vi "EC_Applied_XYZ_MM_BR_RES_2_NC_GR_pxi_Acc3_preset_LIM4.vi"() -> ()   [LabVIEW 2009]
uses:
  <vilib>/Utility/file.llb/Read From Spreadsheet File (I64).vi
  <vilib>/Utility/file.llb/Read From Spreadsheet File (string).vi
  <vilib>/Instr/_visa.llb/VISA Configure Serial Port (Instr).vi
  <vilib>/Utility/file.llb/Write To Spreadsheet File (I64).vi
  <vilib>/Utility/file.llb/Write To Spreadsheet File (string).vi
panel:
  out "R Velocity MVdeg/sec":dbl format="%.3f"
  out "R Position MV deg":dbl
  out "Z Velocity MV mm/sec":dbl format="%.3f"
  out "Z Position MV mm":dbl
  out "Y Velocity MV mm/sec":dbl format="%.3f"
  out "Y Position MV mm":dbl
  out "X Velocity MV mm/sec":dbl format="%.3f"
  out "X Position MV mm":dbl
  out "Presets":i32[][](array[numeric])
  in  "stop":bool
  in  "Tab Control 3":enum32{"Status", "Reset"}(tab)
  out "Y in Range":bool
  out "Y Scan":bool
  out "Y in Motion":bool
  out "Y Backlash corr":bool
  out "X  in Range":bool
  out "X Scan":bool
  out "X  in Motion":bool
  out "X Backlash corr":bool
  out "Z in Range":bool
  out "Z Scan":bool
  out "Z in Motion":bool
  out "Z Backlash corr":bool
  out "R in Range":bool
  out "R Scan":bool
  out "R in Motion":bool
  out "R Backlash corr":bool
  out "X Ready":bool
  out "Y Ready":bool
  out "Z Ready":bool
  out "R Ready":bool
  in  "Reset Y Position mm":dbl
  out "Reset Y Motor Steps":i32
  in  "Reset X Position mm":dbl
  out "Reset X Motor Steps":i32
  in  "Reset Z Position mm":dbl
  out "Reset Z Motor Steps":i32
  in  "Reset R Position deg":dbl
  out "Reset R Motor Steps":i32
  in  "Reset":bool
  in  "Tab Control 2":enum32{"mm", "step"}(tab)
  in  "X Scan Length SP mm":dbl
  in  "X Scan Velocity SP mm/sec":dbl
  in  "X Scan set":bool
  in  "Y Scan Length SP mm":dbl
  in  "Y Scan Velocity SP mm/sec":dbl
  in  "Y Scan set":bool
  in  "Z Scan Length SP mm":dbl
  in  "Z Scan Velocity SP mm/sec":dbl
  in  "Z Scan set":bool
  in  "R Scan Length SP deg":dbl
  in  "R Scan Velocity SP deg/sec":dbl
  in  "R Scan set":bool
  in  "X Scan Velocity SP steps/sec":i32=1 min=1 max=102400 step=1
  in  "X Scan Length SP steps":i32 min=-500000 max=500000 step=100
  out "X Scan length MV mm":dbl
  out "X Scan velocity MV mm/sec":dbl format="%#_6f"
  in  "Y Scan Velocity SP steps/sec":i32=1 min=1 max=102400 step=1
  in  "Y Scan Length SP steps":i32 min=-1000000 max=0 step=100
  out "Y Scan length MV mm":dbl
  out "Y Scan velocity MV mm/sec":dbl format="%#_6f"
  in  "Z Scan Velocity SP steps/sec":i32=1 min=1 max=102400 step=1
  in  "Z Scan Length SP steps":i32 min=-204724 max=102195276 step=100
  out "Z Scan length MV mm":dbl
  out "Z Scan velocity MV mm/sec":dbl format="%#_6f"
  in  "R Scan Velocity SP steps/sec":i32=1 min=1 max=102400 step=1
  in  "R Scan Length SP steps":i32 min=-6144000 max=0 step=100
  out "R Scan length MV deg":dbl
  out "R Scan velocity MV deg/sec":dbl format="%#_6f"
  out "atan Y/Z":dbl
  in  "Tab Control":enum32{"mm", "preset", "step"}(tab)
  in  "X Position SP mm":dbl
  in  "X Velocity SP mm/sec":dbl
  in  "X Move Set":bool
  in  "Y Move Set":bool
  in  "Y Position SP mm":dbl
  in  "Y Velocity SP mm/sec":dbl
  in  "Z Position SP mm":dbl
  in  "Z Velocity SP mm/sec":dbl
  in  "Z Move Set":bool
  in  "R Position SP deg":dbl
  in  "R Velocity SP deg/sec":dbl
  in  "R Move Set":bool
  in  "Add Button":bool
  in  "String":string
  in  "Delete Button":bool
  in  "Preset positions":i32(ring)
  in  "Set Button":bool
  in  "X Velocity SP step/sec":i32 min=1 max=50000
  in  "Y Velocity SP step/sec":i32 min=1 max=50000
  in  "Z Velocity SP step/sec":i32 min=1 max=5000
  in  "R Velocity SP step/sec":i32 min=1 max=10000
  in  "Y Step SP":i32=-20000 min=-750000 max=750000 step=500
  in  "X Step SP":i32=-20000 min=-750000 max=750000 step=500
  in  "Z Step SP":i32=-20000 min=0 max=102400000 step=500
  in  "R Step SP":i32=-20000 min=-6144000 max=0 step=500
  out "X Step PV":i32 max=2000
  out "Y Step PV":i32 max=2000
  out "Z Step PV":i32 max=2000
  out "R Step PV":i32 max=2000
  out "X Scan Duration":dbl
  out "Y Scan Duration":dbl
  out "Z Scan Duration":dbl
  out "R Scan Duration":dbl
  out "R Backlash steps/sec":i32
  out "R Backlash":i32
  out "R Holding Current %":i32
  out "R Run Current %":i32
  out "R offset deg":dbl
  out "R deg/rev":dbl
  out "R steps/rev":u32
  out "R velocity PV step/sec":i32
  out "R MINPOS":i32=-94296
  out "R MAXPOS":i32=-34296
  out "R COM PORT":refnum<visa-resource-name>="COM5"
  in  "R Scan OK":bool
  in  "R Go":bool
  out "R Position deg PV":dbl
  out "Z COM PORT":refnum<visa-resource-name>="COM5"
  out "Z Backlash steps/sec":i32
  out "Z Backlash":i32
  out "Z Holding Current %":i32
  out "Z Run Current %":i32
  out "Z offset mm":dbl
  out "Z mm/rev":dbl
  out "Z steps/rev":u32
  out "Z  velocity PV step/sec":i32
  out "Z MINPOS":i32=-94296
  out "Z MAXPOS":i32=-34296
  in  "Z Scan OK":bool
  in  "Z Go":bool
  out "Z Position mm PV":dbl
  out "X Position mm PV":dbl
  out "X velocity PV step/sec":i32
  in  "X Scan OK":bool
  in  "X Go":bool
  out "X Backlash steps/sec":i32
  out "X Backlash":i32
  out "X Holding Current %":i32
  out "X Run Current %":i32
  out "X offset mm":dbl
  out "X mm/rev":dbl
  out "X steps/rev":u32
  out "X MAXPOS":i32=-34296
  out "X MINPOS":i32=-94296
  out "X COM PORT":refnum<visa-resource-name>="COM5"
  out "Y Backlash steps/sec":i32
  out "Y Backlash":i32
  out "Y Holding Current %":i32
  out "Y Run Current %":i32
  in  "Scan Cancel":bool
  out "Y Position mm PV":dbl
  out "Y offset mm":dbl
  out "Y mm/rev":dbl
  out "Y steps/rev":u32
  out "Y velocity PV step/sec":i32
  in  "Y Scan OK":bool
  in  "Scan Go":bool
  in  "Stop":bool
  in  "Y Go":bool
  out "Y MINPOS":i32=-94296
  out "Y MAXPOS":i32=-34296
  out "Y COM PORT":refnum<visa-resource-name>="COM5"
  # "Current position"
  # "Goto position"
  # "RX"
  # "RY"
  # "RZ"
  # "RR"
  # "L"
  # "M"
  # "B"
  # "S"
  # "R"
  # "Preset position"
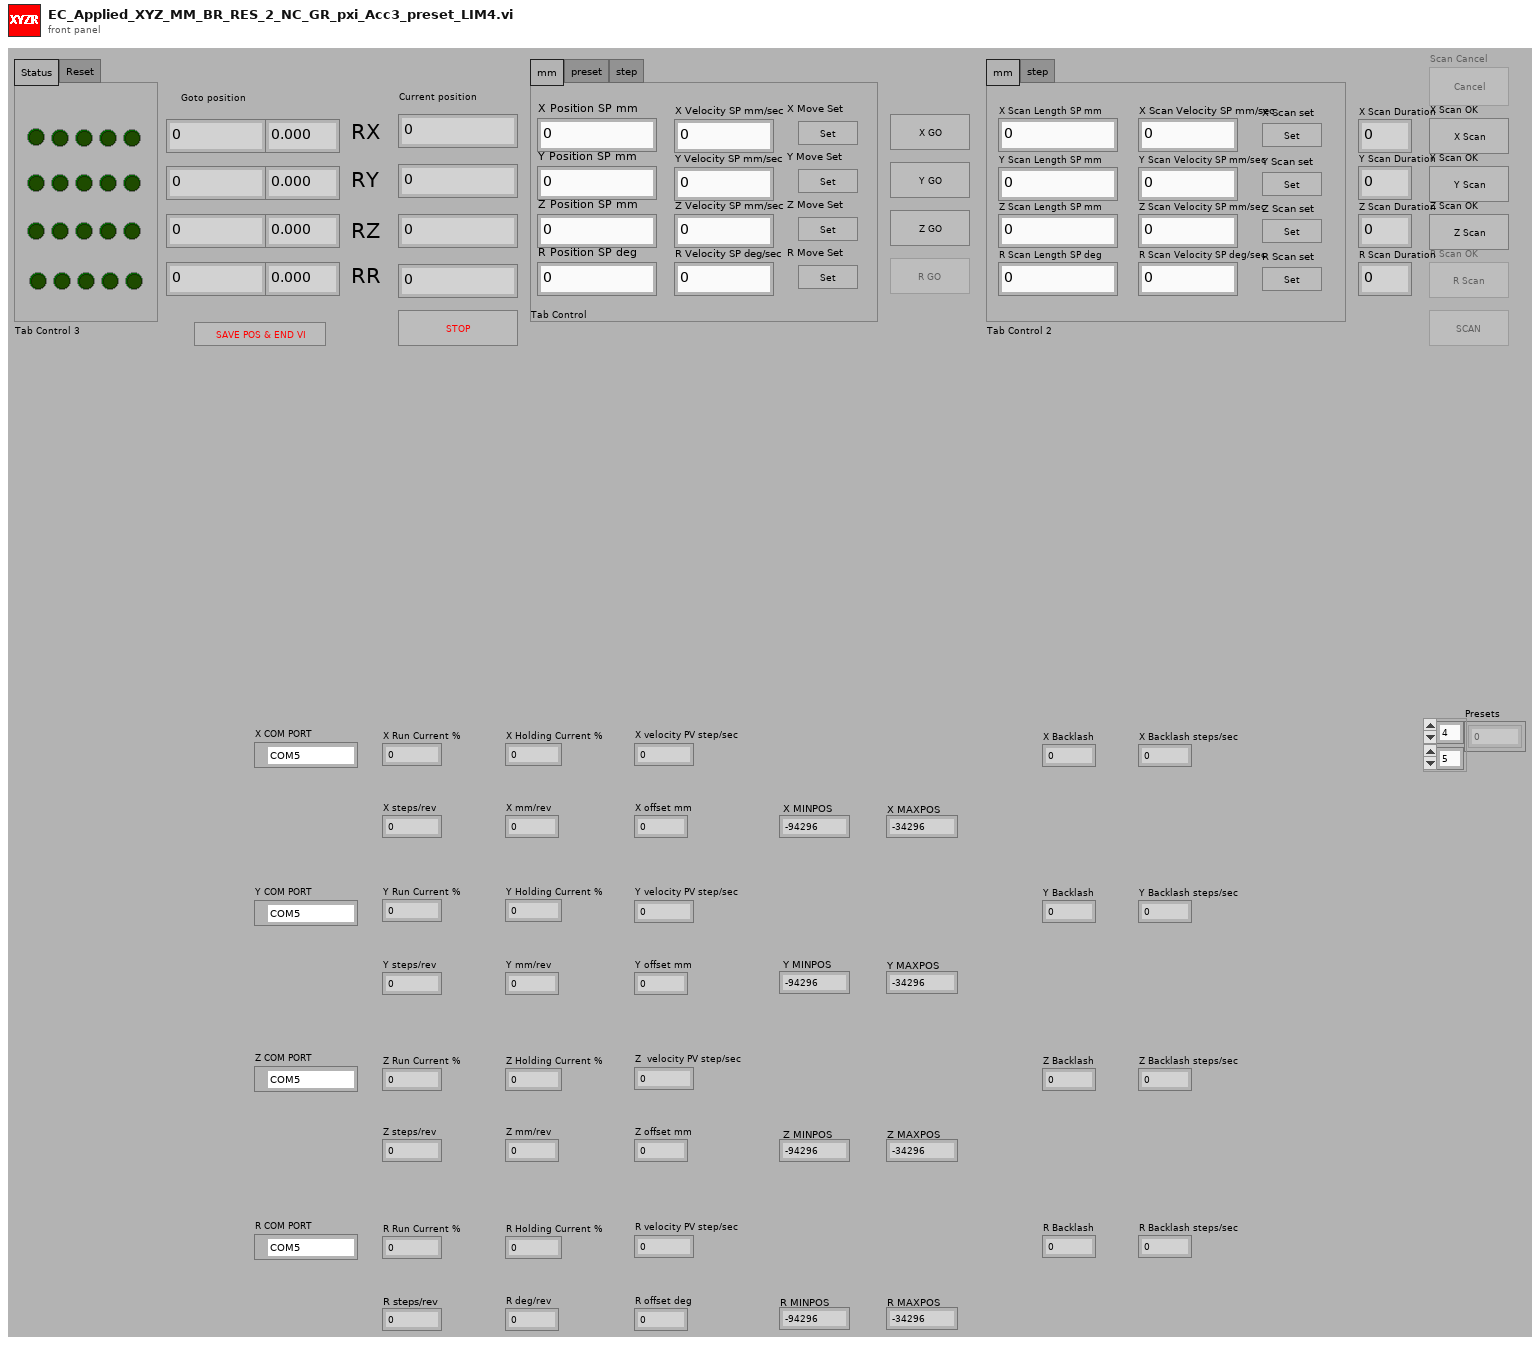
[diagram p1: front panel]
types:
  T1 = enum16{"Power-up Signature", "Accel Rate", "Accel Max", "Bit Rate", "Buffer Status", "Change Current", "Commence Jogging", "Change Jog Speed", "Continue", "Define Address", "Distance for FC,FM,FO,FY", "Decel Rate", "Distance or Position", "Define Limits", "Encoder Deadband", "Encoder Function", "Encoder Position", "Encoder Ratio", "Feed to Length with Speed Change", "Feed to Length", "Feed to Sensor with Mask Dist", "Feed to Length & Set Output", "Feed to Position", "Feed to Sensor", "Feed to Sensor w/safety", "Follow Handwheel", "Immediate Distance?", "Immediate Encoder?", "Immediate Low Output", "Immediate High Output", "Immediate Position?", "Input Status?", "Jog Accel/Decel", "Jog Disable", "Jog Enable", "Jog Speed", "Motor Disable", "Motor Enable", "Microstep Resolution", "Power up Current", "Power up Mode", "Pause", "Request Status", "Revision Level?", "Seek Home", "Stop Jogging", "Stop & Kill Buffer", "Set Output", "Set ABS Position", "Send String", "Stop", "Velocity for Speed Change", "Velocity Setting", "Wait for Input", "Wait Time"}
  T2 = enum8{"Enabled", "Disabled", "Disabled and Grayed Out"}
  T3 = cluster{"first row[0]":i64, "first row[1]":i64, "first row[2]":i64, "first row[3]":i64, "first row[4]":i64, "first row[5]":i64, "first row[6]":i64, "first row[7]":i64, "first row[8]":i64}
  T4 = cluster{"Value[0]":i32, "Value[1]":i32, "Value[2]":i32, "Value[3]":i32, "Value[4]":i32, "Value[5]":i32, "Value[6]":i32, "Value[7]":i32, "Value[8]":i32}
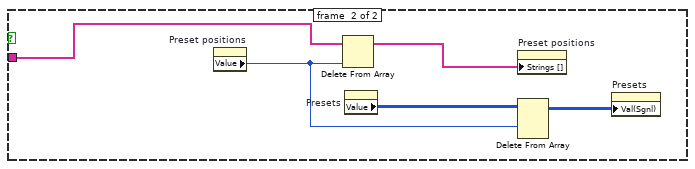
[diagram p2: hidden frame]
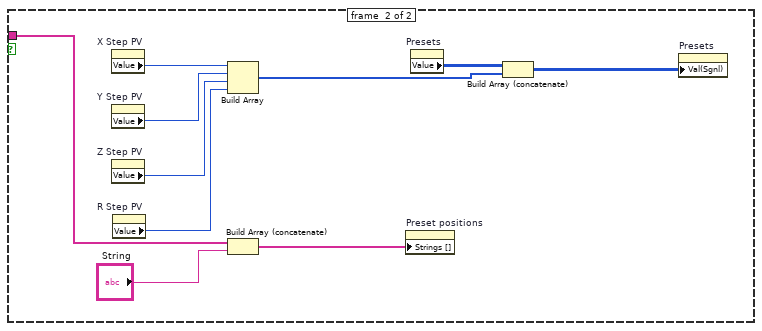
[diagram p3: hidden frame]
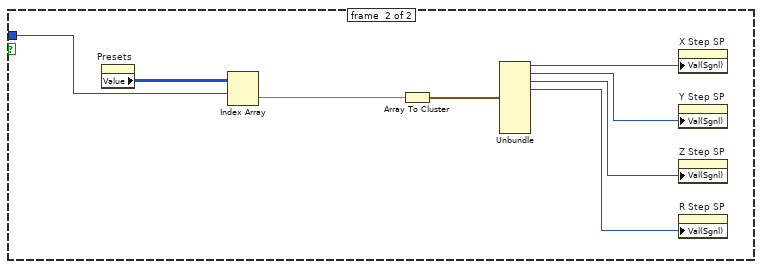
[diagram p4: hidden frame]
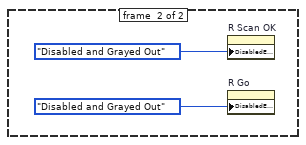
[diagram p5: hidden frame]
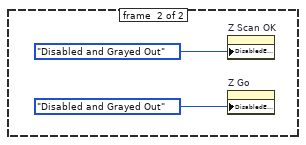
[diagram p8: hidden frame]
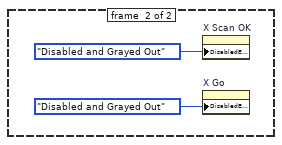
[diagram p11: hidden frame]
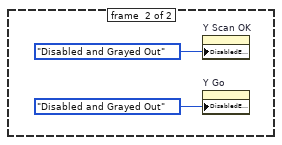
[diagram p14: hidden frame]
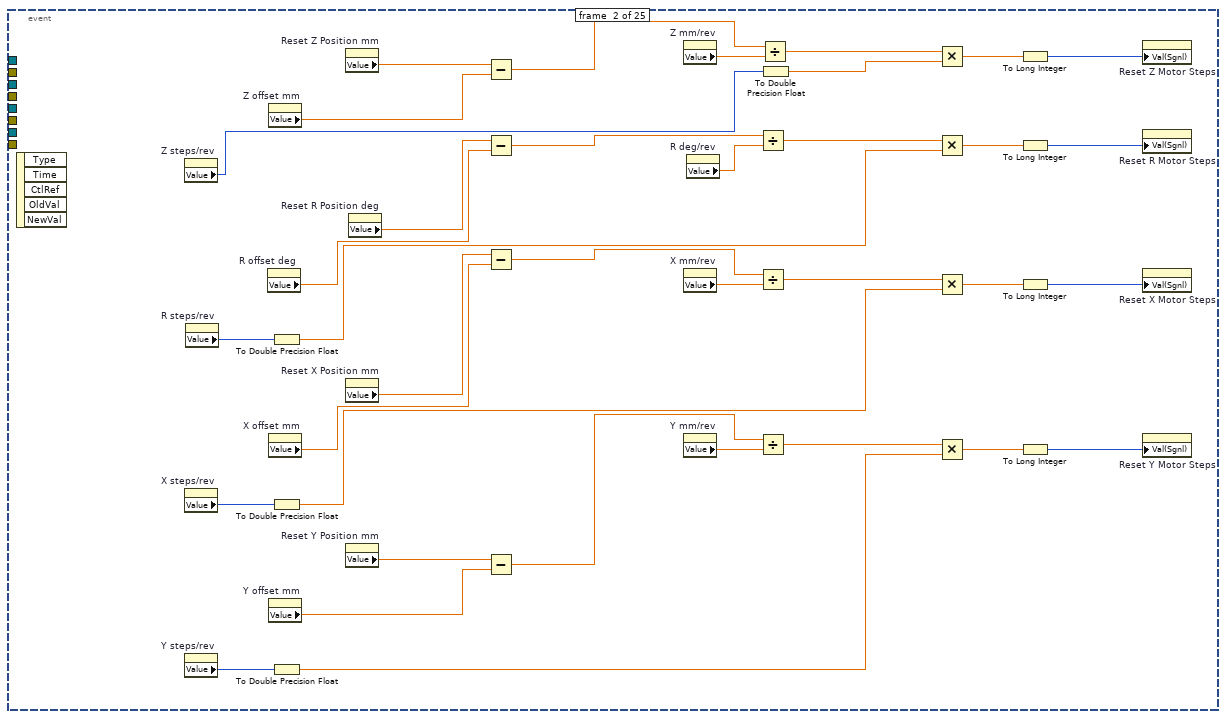
[diagram p17: hidden frame]
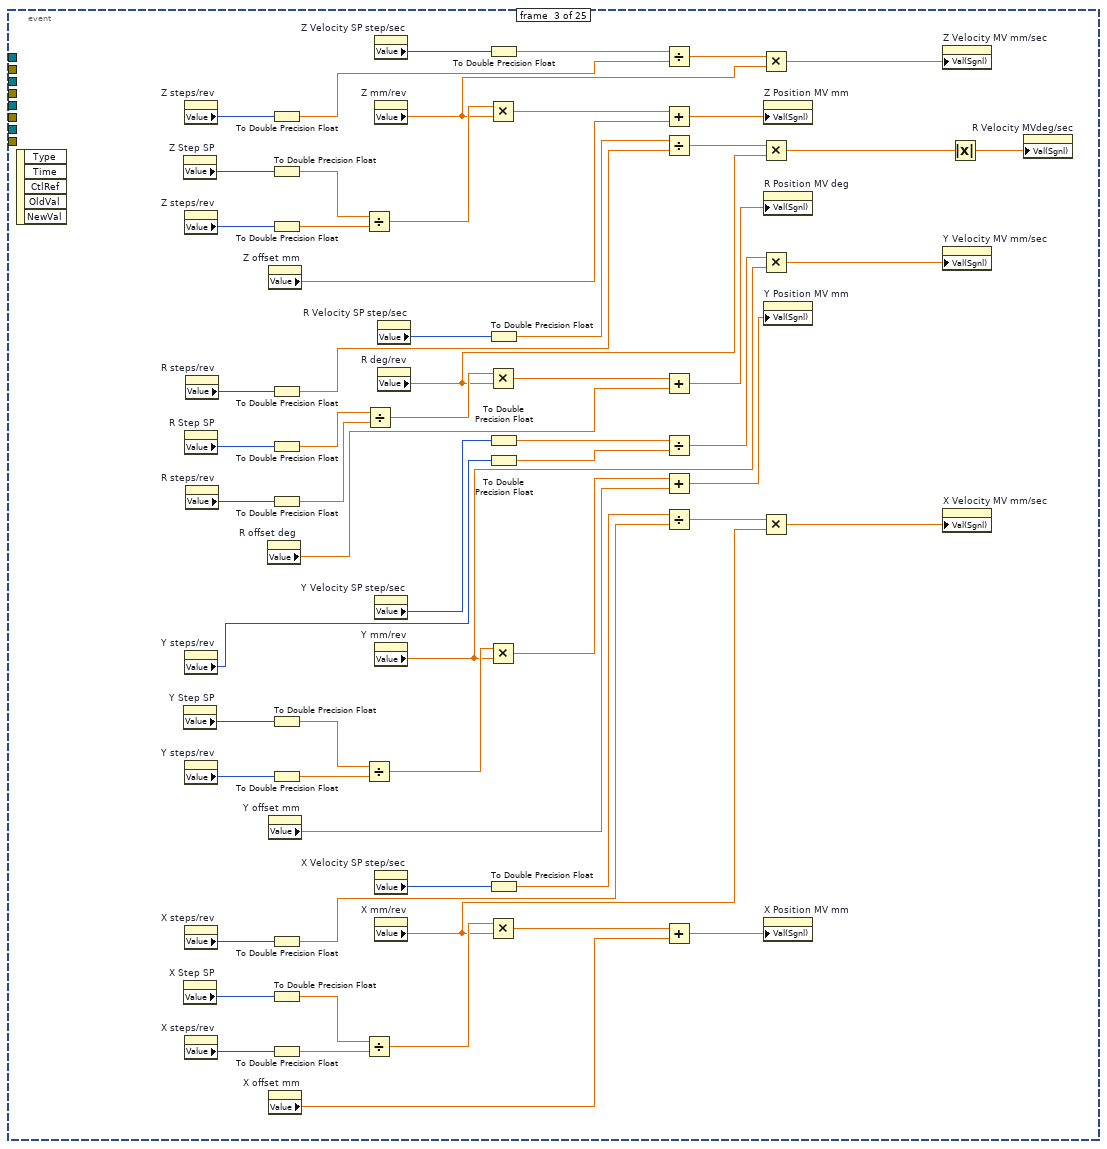
[diagram p18: hidden frame]
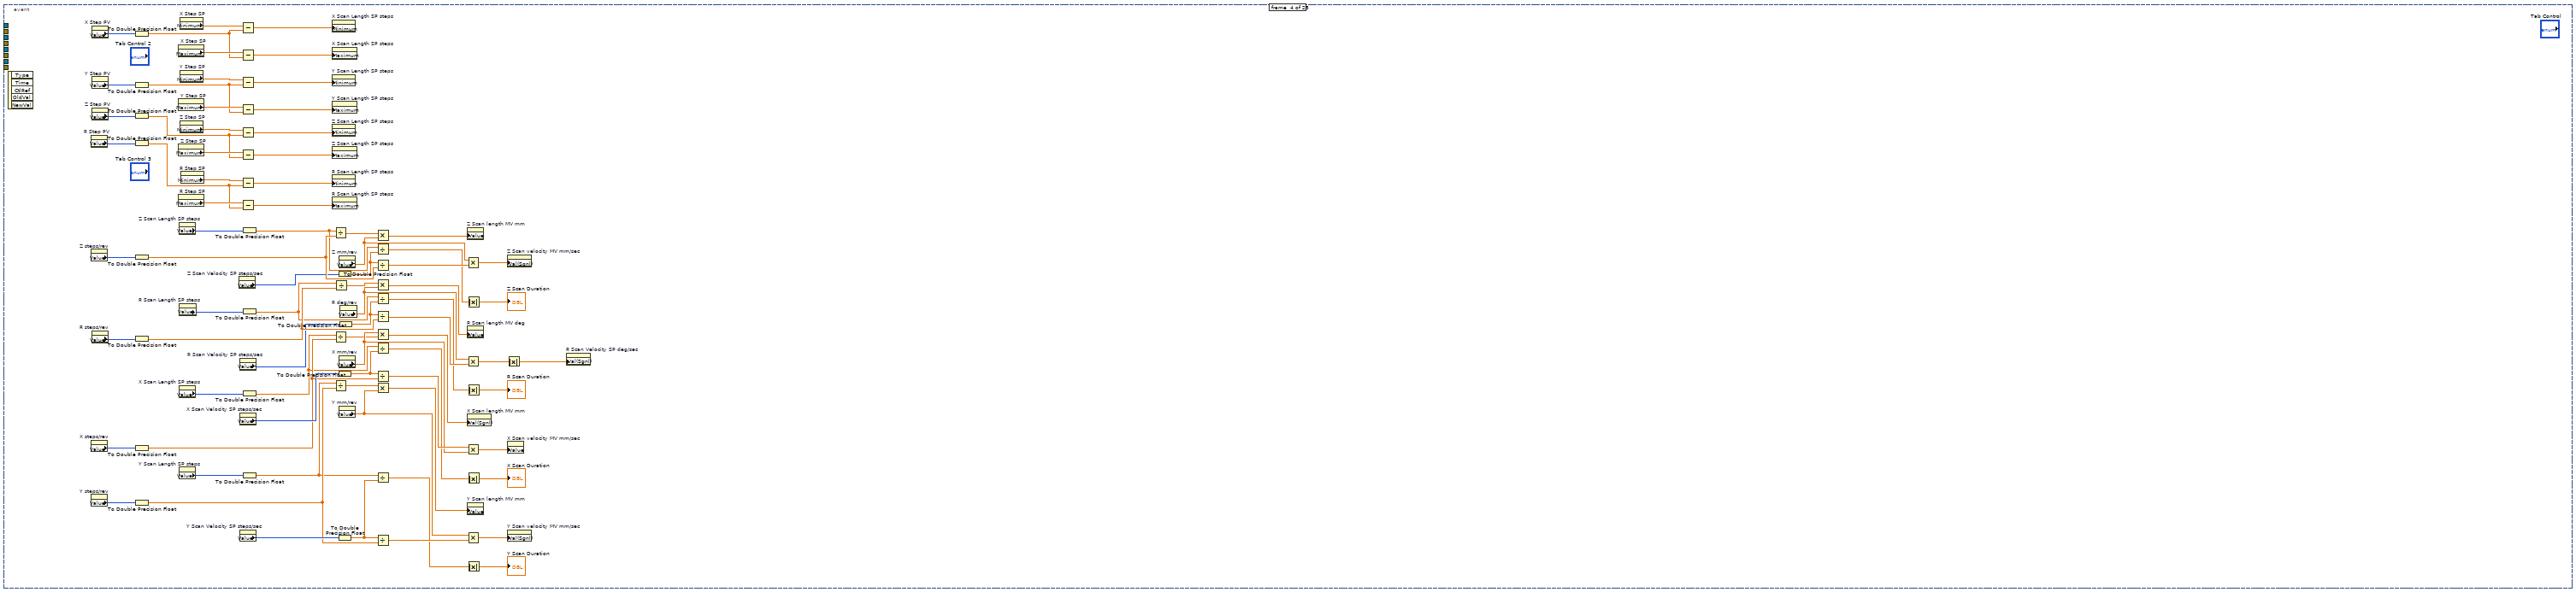
[diagram p19: hidden frame]
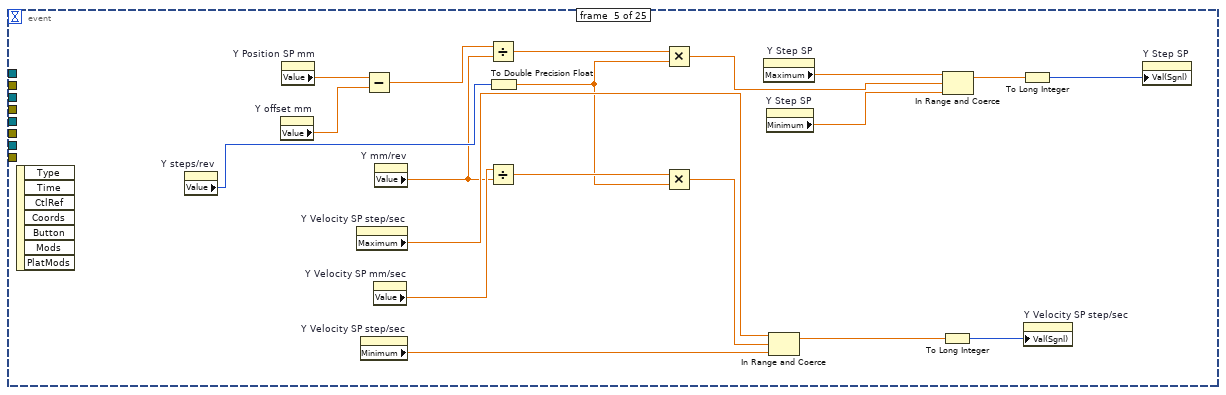
[diagram p20: hidden frame]
diagram:
  w24 = 0 ("dimension size")
  n1 = flat-sequence {
    tunnel: [w93] -> w10
    tunnel: [w92] -> w9
    tunnel: w10 -> [w107]
    tunnel: w9 -> [w106]
    tunnel: [w105] -> w8
    tunnel: [w104] -> w7
    tunnel: [w115] -> w64
    tunnel: [w114] -> w63
    tunnel: w8 -> [w117]
    tunnel: w7 -> [w116]
    tunnel: w64 -> [w132]
    tunnel: w63 -> [w131]
    tunnel: [w133] -> w62
    tunnel: [w134] -> w61
    tunnel: [w135] -> w6
    tunnel: [w146] -> w55
    tunnel: [w147] -> w56
    tunnel: w62 -> [w147]
    tunnel: w61 -> [w146]
    tunnel: w6 -> [w144]
    frame #0 {
      "Z Run Current %" <- 100 ("Z Run Current %")
      "Z Holding Current %" <- 50 ("Z Holding Current %")
    }
    frame #1 {
      "Z Backlash steps/sec" <- 1000 ("Z Backlash steps/sec")
      "Z Backlash" <- -5000 ("Z Backlash")
    }
    frame #2 {
      w83 = 2.54 ("Z mm/rev")
      w82 = u32 20000 ("step/rev")
      w84 = 5000 ("Value (Signaling)")
      n2 = property on="Z Scan Velocity SP mm/sec" class="DigNum (strict)"("Val(Sgnl)"=0.1 ("Value (Signaling)")) -> ()  [unwired: 2 in, 2 out]
      n3 = property on="Z Velocity SP step/sec" class="DigNum (strict)"("Val(Sgnl)"=w84) -> ()  [unwired: 2 in, 2 out]
      n4 = property on="Z Velocity SP step/sec" class="DigNum (strict)"("Minimum"=1.0 ("Data Entry Limits:Minimum")) -> ()  [unwired: 2 in, 2 out]
      n5 = To Double Precision Float(number=w84) -> (double precision float=w88:dbl)
      n6 = To Double Precision Float(number=w82) -> (double precision float=w87:dbl)
      n7 = property on="Z Velocity SP step/sec" class="DigNum (strict)"("Maximum"=w88) -> ()  [unwired: 2 in, 2 out]
      n8 = Divide(x=w88, y=w87) -> (x/y=w85:dbl)
      n9 = Multiply(x=w85, y=w83) -> (x*y=w86:dbl)
      n10 = property on="Z Velocity SP mm/sec" class="DigNum (strict)"("Val(Sgnl)"=w86) -> ()  [unwired: 2 in, 2 out]
      "Z mm/rev" <- w83
      "Z steps/rev" <- w82
    }
    frame #3 {
      w90 = 0 ("lower limit")
      w89 = 102400000 ("upper limit")
      n11 = property on="Z Step SP" class="DigNum (strict)"("Minimum"=w90) -> ()  [unwired: 2 in, 2 out]
      n12 = property on="Z Step SP" class="DigNum (strict)"("Maximum"=w89) -> ()  [unwired: 2 in, 2 out]
      "Z offset mm" <- 0.0 ("Z offset mm")
      "Z MINPOS" <- w90
      "Z MAXPOS" <- w89
    }
    frame #4 {
      w100 = refnum<visa-resource-name> "COM15" ("COM PORT")
      w98 = u16 0 items=["None", "XON/XOFF", "RTS/CTS", "XON/XOFF & RTS/CTS", "DTR/DSR", "XON/XOFF & DTR/DSR"] ("flow control (0:none)")
      w97 = u16 10 items=["1.0"=10, "1.5"=15, "2.0"=20] ("stop bits (10: 1 bit)")
      # "Stop bits"
      n13 = call-poly "VISA Configure Serial Port"("VISA resource name"=w100, "timeout (10sec)"=u32 10000, "baud rate (9600)"=u32 9600, "data bits (8)"=u16 8, "parity (0:none)"=enum16{"None", "Odd", "Even", "Mark", "Space"}."None", "stop bits (10: 1 bit)"=w97, "flow control (0:none)"=w98) -> ("VISA resource name out"=w93:refnum<visa-resource-name>, "error out"=w92:errorcluster)  [unwired: 7 in]
      "Z COM PORT" <- w100
    }
    frame #5 {
      # "Run Current %"
      n14 = property on="Z Run Current %" class="DigNum (strict)"() -> ("Value"=w108:i32)  [unwired: 2 in, 2 out]
      n15 = Divide(x=w108, y=100) -> (x/y=w109:dbl)
      n16 = Multiply(x=w109, y=3.5) -> (x*y=w103:dbl)
      n17 = Number To Fractional String(number=w103) -> (F-format string=w110:string)  [unwired: 3 in]
      n18 = call "Applied Send Command.vi"("error in (no error)"=w106, "Extra"=w110, "Command"=T1."Change Current", "VISA resource name"=w107) -> ("error out"=w104:errorcluster, "VISA resource name out"=w105:refnum<visa-resource-name>)  [unwired: 3 in, 1 out]
    }
    frame #6 {
      # "VELOCITY"
      n19 = property on="Z steps/rev" class="DigNum (strict)"() -> ("Value"=w113:u32)  [unwired: 2 in, 2 out]
      n20 = property on="Z Velocity SP step/sec" class="DigNum (strict)"() -> ("Value"=w112:i32)  [unwired: 2 in, 2 out]
      n21 = Divide(x=w112, y=w113) -> (x/y=w120:dbl)
      n22 = Number To Fractional String(number=w120) -> (F-format string=w122:string)  [unwired: 3 in]
      n23 = call "Applied Send Command.vi"("error in (no error)"=w116, "Extra"=w122, "Command"=T1."Velocity Setting", "VISA resource name"=w117) -> ("error out"=w123:errorcluster, "VISA resource name out"=w130:refnum<visa-resource-name>)  [unwired: 3 in, 1 out]
      n24 = call "Time Delay2"("error in (no error)"=w123, "Delay Time (s)"=0.1) -> ("error out"=w128:errorcluster)  [unwired: 9 in]
      n25 = call "Applied Send Command.vi"("error in (no error)"=w128, "Extra"="", "Command"=T1."Velocity Setting", "VISA resource name"=w130) -> ("error out"=w114:errorcluster, "read buffer"=w126:string, "VISA resource name out"=w115:refnum<visa-resource-name>)  [unwired: 3 in]
      n26 = Fract/Exp String To Number(string=w126, offset=3) -> (number=w121:dbl)  [unwired: 2 in, 1 out]
      n27 = Multiply(x=w121, y=w113) -> (x*y=w118:dbl)
      n28 = property on="Z  velocity PV step/sec" class="DigNum (strict)"("Val(Sgnl)"=w118) -> ()  [unwired: 2 in, 2 out]
    }
    frame #7 {
      # "GET CURRENT POSITION"
      n29 = call "Applied Send Command.vi"("error in (no error)"=w131, "Extra"="", "Command"=T1."Immediate Position?", "VISA resource name"=w132) -> ("error out"=w137:errorcluster, "read buffer"=w139:string, "VISA resource name out"=w133:refnum<visa-resource-name>)  [unwired: 3 in]
      n30 = call "Time Delay8"("error in (no error)"=w137, "Delay Time (s)"=0.1) -> ("error out"=w134:errorcluster)  [unwired: 9 in]
      n31 = Hexadecimal String To Number(string=w139, offset=3) -> (number=w135:u32)  [unwired: 1 in, 1 out]
    }
    frame #8 {
      n32 = property on="Z Step SP" class="DigNum (strict)"() -> ("Maximum"=w143:dbl)  [unwired: 2 in, 2 out]
      n33 = property on="Z Step SP" class="DigNum (strict)"("Val(Sgnl)"=w144) -> ()  [unwired: 2 in, 2 out]
      n34 = property on="Z Step SP" class="DigNum (strict)"() -> ("Minimum"=w142:dbl)  [unwired: 2 in, 2 out]
      n35 = In Range and Coerce(upper limit=w143, x=w144, lower limit=w142) -> (In Range?=w145:bool)  [unwired: 1 out]
      n36 = property on="Z in Range" class="Bool (strict)"("Val(Sgnl)"=w145) -> ()  [unwired: 2 in, 2 out]
    }
  }
  n37 = flat-sequence {
    tunnel: [w166] -> w3
    tunnel: [w165] -> w2
    tunnel: [w180] -> w5
    tunnel: [w179] -> w4
    tunnel: w3 -> [w178]
    tunnel: w2 -> [w177]
    tunnel: [w187] -> w60
    tunnel: [w188] -> w59
    tunnel: w5 -> [w185]
    tunnel: w4 -> [w186]
    tunnel: w60 -> [w205]
    tunnel: w59 -> [w204]
    tunnel: [w206] -> w58
    tunnel: [w208] -> w57
    tunnel: [w207] -> w1
    tunnel: [w219] -> w53
    tunnel: [w220] -> w54
    tunnel: w58 -> [w219]
    tunnel: w57 -> [w217]
    tunnel: w1 -> [w220]
    frame #0 {
      "R Run Current %" <- 100 ("R Run Current %")
      "R Holding Current %" <- 50 ("R Holding Current %")
    }
    frame #1 {
      "R Backlash" <- -12800 ("R Backlash")
      "R Backlash steps/sec" <- 6400 ("R Backlash steps/sec")
    }
    frame #2 {
      w156 = -3.0 ("R deg/rev")
      w158 = u32 20000 ("step/rev")
      w154 = 10000 ("Value (Signaling)")
      n38 = property on="R Velocity SP step/sec" class="DigNum (strict)"("Minimum"=1.0 ("Data Entry Limits:Minimum")) -> ()  [unwired: 2 in, 2 out]
      n39 = property on="R Velocity SP step/sec" class="DigNum (strict)"("Val(Sgnl)"=w154) -> ()  [unwired: 2 in, 2 out]
      n40 = property on="R Velocity SP deg/sec" class="DigNum (strict)"("Val(Sgnl)"=0.1 ("Value (Signaling)")) -> ()  [unwired: 2 in, 2 out]
      n41 = To Double Precision Float(number=w154) -> (double precision float=w152:dbl)
      n42 = To Double Precision Float(number=w158) -> (double precision float=w157:dbl)
      n43 = property on="R Velocity SP step/sec" class="DigNum (strict)"("Maximum"=w152) -> ()  [unwired: 2 in, 2 out]
      n44 = Divide(x=w152, y=w157) -> (x/y=w153:dbl)
      n45 = Multiply(x=w153, y=w156) -> (x*y=w155:dbl)
      n46 = Absolute Value(x=w155) -> (abs(x)=w160:dbl)
      n47 = property on="R Velocity SP deg/sec" class="DigNum (strict)"("Val(Sgnl)"=w160) -> ()  [unwired: 2 in, 2 out]
      "R deg/rev" <- w156
      "R steps/rev" <- w158
    }
    frame #3 {
      w163 = 0 ("upper limit")
      w164 = -6144000 ("lower limit")
      n48 = property on="R Step SP" class="DigNum (strict)"("Minimum"=w164) -> ()  [unwired: 2 in, 2 out]
      n49 = property on="R Step SP" class="DigNum (strict)"("Maximum"=w163) -> ()  [unwired: 2 in, 2 out]
      "R MINPOS" <- w163
      "R MAXPOS" <- w164
      "R offset deg" <- 0.0 ("R offset deg")
    }
    frame #4 {
      w173 = refnum<visa-resource-name> "COM12" ("COM PORT")
      w171 = u16 0 items=["None", "XON/XOFF", "RTS/CTS", "XON/XOFF & RTS/CTS", "DTR/DSR", "XON/XOFF & DTR/DSR"] ("flow control (0:none)")
      w170 = u16 10 items=["1.0"=10, "1.5"=15, "2.0"=20] ("stop bits (10: 1 bit)")
      # "Stop bits"
      n50 = call-poly "VISA Configure Serial Port"("VISA resource name"=w173, "timeout (10sec)"=u32 10000, "baud rate (9600)"=u32 9600, "data bits (8)"=u16 8, "parity (0:none)"=enum16{"None", "Odd", "Even", "Mark", "Space"}."None", "stop bits (10: 1 bit)"=w170, "flow control (0:none)"=w171) -> ("VISA resource name out"=w166:refnum<visa-resource-name>, "error out"=w165:errorcluster)  [unwired: 7 in]
      "R COM PORT" <- w173
    }
    frame #5 {
      # "Run Current %"
      n51 = property on="R Run Current %" class="DigNum (strict)"() -> ("Value"=w181:i32)  [unwired: 2 in, 2 out]
      n52 = Divide(x=w181, y=100) -> (x/y=w182:dbl)
      n53 = Multiply(x=w182, y=3.5) -> (x*y=w176:dbl)
      n54 = Number To Fractional String(number=w176) -> (F-format string=w183:string)  [unwired: 3 in]
      n55 = call "Applied Send Command.vi"("error in (no error)"=w177, "Extra"=w183, "Command"=T1."Change Current", "VISA resource name"=w178) -> ("error out"=w179:errorcluster, "VISA resource name out"=w180:refnum<visa-resource-name>)  [unwired: 3 in, 1 out]
    }
    frame #6 {
      # "VELOCITY"
      n56 = property on="R steps/rev" class="DigNum (strict)"() -> ("Value"=w191:u32)  [unwired: 2 in, 2 out]
      n57 = property on="R Velocity SP step/sec" class="DigNum (strict)"() -> ("Value"=w189:i32)  [unwired: 2 in, 2 out]
      n58 = Divide(x=w189, y=w191) -> (x/y=w193:dbl)
      n59 = Number To Fractional String(number=w193) -> (F-format string=w195:string)  [unwired: 3 in]
      n60 = call "Applied Send Command.vi"("error in (no error)"=w186, "Extra"=w195, "Command"=T1."Velocity Setting", "VISA resource name"=w185) -> ("error out"=w196:errorcluster, "VISA resource name out"=w203:refnum<visa-resource-name>)  [unwired: 3 in, 1 out]
      n61 = call "Time Delay43"("error in (no error)"=w196, "Delay Time (s)"=0.1) -> ("error out"=w201:errorcluster)  [unwired: 9 in]
      n62 = call "Applied Send Command.vi"("error in (no error)"=w201, "Extra"="", "Command"=T1."Velocity Setting", "VISA resource name"=w203) -> ("error out"=w188:errorcluster, "read buffer"=w199:string, "VISA resource name out"=w187:refnum<visa-resource-name>)  [unwired: 3 in]
      n63 = Fract/Exp String To Number(string=w199, offset=3) -> (number=w194:dbl)  [unwired: 2 in, 1 out]
      n64 = Multiply(x=w194, y=w191) -> (x*y=w190:dbl)
      n65 = property on="R velocity PV step/sec" class="DigNum (strict)"("Val(Sgnl)"=w190) -> ()  [unwired: 2 in, 2 out]
    }
    frame #7 {
      # "GET CURRENT POSITION"
      n66 = call "Applied Send Command.vi"("error in (no error)"=w204, "Extra"="", "Command"=T1."Immediate Position?", "VISA resource name"=w205) -> ("error out"=w210:errorcluster, "read buffer"=w212:string, "VISA resource name out"=w207:refnum<visa-resource-name>)  [unwired: 3 in]
      n67 = call "Time Delay42"("error in (no error)"=w210, "Delay Time (s)"=0.1) -> ("error out"=w206:errorcluster)  [unwired: 9 in]
      n68 = Hexadecimal String To Number(string=w212, offset=3) -> (number=w208:u32)  [unwired: 1 in, 1 out]
    }
    frame #8 {
      n69 = property on="R Step SP" class="DigNum (strict)"() -> ("Maximum"=w215:dbl)  [unwired: 2 in, 2 out]
      n70 = property on="R Step SP" class="DigNum (strict)"("Val(Sgnl)"=w217) -> ()  [unwired: 2 in, 2 out]
      n71 = property on="R Step SP" class="DigNum (strict)"() -> ("Minimum"=w216:dbl)  [unwired: 2 in, 2 out]
      n72 = In Range and Coerce(upper limit=w215, x=w217, lower limit=w216) -> (In Range?=w218:bool)  [unwired: 1 out]
      n73 = property on="R in Range" class="Bool (strict)"("Val(Sgnl)"=w218) -> ()  [unwired: 2 in, 2 out]
    }
  }
  n74 = flat-sequence {
    frame #0 {
      n75 = property on="X Scan" class="Bool (strict)"("Val(Sgnl)"=FALSE ("Value (Signaling)")) -> ()  [unwired: 2 in, 2 out]
      n76 = property on="Y Scan" class="Bool (strict)"("Val(Sgnl)"=FALSE ("Value (Signaling)")) -> ()  [unwired: 2 in, 2 out]
      n77 = property on="Z Scan" class="Bool (strict)"("Val(Sgnl)"=FALSE ("Value (Signaling)")) -> ()  [unwired: 2 in, 2 out]
      n78 = property on="R Scan" class="Bool (strict)"("Val(Sgnl)"=FALSE ("Value (Signaling)")) -> ()  [unwired: 2 in, 2 out]
      n79 = property on="Scan Go" class="Bool"("DisabledEnum"=T2."Disabled and Grayed Out" ("Disabled")) -> ()  [unwired: 2 in, 2 out]
      n80 = property on="Scan Cancel" class="Bool"("DisabledEnum"=T2."Disabled and Grayed Out" ("Disabled")) -> ()  [unwired: 2 in, 2 out]
    }
    frame #1 {
      n81 = property on="Y Backlash corr" class="Bool (strict)"("Val(Sgnl)"=FALSE ("Value (Signaling)")) -> ()  [unwired: 2 in, 2 out]
      n82 = property on="R Backlash corr" class="Bool (strict)"("Val(Sgnl)"=FALSE ("Value (Signaling)")) -> ()  [unwired: 2 in, 2 out]
      n83 = property on="X Backlash corr" class="Bool (strict)"("Val(Sgnl)"=FALSE ("Value (Signaling)")) -> ()  [unwired: 2 in, 2 out]
      n84 = property on="Z Backlash corr" class="Bool (strict)"("Val(Sgnl)"=FALSE ("Value (Signaling)")) -> ()  [unwired: 2 in, 2 out]
    }
  }
  n85 = flat-sequence {
    tunnel: [w248] -> w18
    tunnel: [w247] -> w17
    tunnel: w18 -> [w262]
    tunnel: w17 -> [w261]
    tunnel: [w260] -> w16
    tunnel: [w259] -> w15
    tunnel: w16 -> [w270]
    tunnel: w15 -> [w269]
    tunnel: [w268] -> w14
    tunnel: [w267] -> w13
    tunnel: [w287] -> w68
    tunnel: w14 -> [w290]
    tunnel: w13 -> [w289]
    tunnel: [w288] -> w12
    tunnel: [w286] -> w11
    tunnel: [w299] -> w74
    tunnel: [w302] -> w75
    tunnel: w68 -> [w299]
    tunnel: w12 -> [w302]
    tunnel: w11 -> [w300]
    frame #0 {
      "Y Run Current %" <- 100 ("Run Current %")
      "Y Holding Current %" <- 50 ("Holding Current %")
    }
    frame #1 {
      "Y Backlash" <- 5000 ("Backlash2")
      "Y Backlash steps/sec" <- 10000 ("Value (Signaling)")
    }
    frame #2 {
      w238 = 0.21167 ("MM/rev")
      w241 = u32 20000 ("step/rev")
      w236 = 50000 ("Value (Signaling)")
      n86 = property on="Y Velocity SP step/sec" class="DigNum (strict)"("Minimum"=1.0 ("Data Entry Limits:Minimum")) -> ()  [unwired: 2 in, 2 out]
      n87 = property on="Y Scan Velocity SP mm/sec" class="DigNum (strict)"("Val(Sgnl)"=0.1 ("Value (Signaling)")) -> ()  [unwired: 2 in, 2 out]
      n88 = property on="Y Velocity SP step/sec" class="DigNum (strict)"("Val(Sgnl)"=w236) -> ()  [unwired: 2 in, 2 out]
      n89 = To Double Precision Float(number=w236) -> (double precision float=w242:dbl)
      n90 = To Double Precision Float(number=w241) -> (double precision float=w240:dbl)
      n91 = property on="Y Velocity SP step/sec" class="DigNum (strict)"("Maximum"=w242) -> ()  [unwired: 2 in, 2 out]
      n92 = Divide(x=w242, y=w240) -> (x/y=w237:dbl)
      n93 = Multiply(x=w237, y=w238) -> (x*y=w239:dbl)
      n94 = property on="Y Velocity SP mm/sec" class="DigNum (strict)"("Val(Sgnl)"=w239) -> ()  [unwired: 2 in, 2 out]
      "Y steps/rev" <- w241
      "Y mm/rev" <- w238
    }
    frame #3 {
      w245 = -800000 ("lower limit")
      w246 = 800000 ("upper limit")
      n95 = property on="Y Step SP" class="DigNum (strict)"("Minimum"=w245) -> ()  [unwired: 2 in, 2 out]
      n96 = property on="Y Step SP" class="DigNum (strict)"("Maximum"=w246) -> ()  [unwired: 2 in, 2 out]
      "Y MAXPOS" <- w246
      "Y MINPOS" <- w245
      "Y offset mm" <- 0.0 ("offset")
    }
    frame #4 {
      w255 = refnum<visa-resource-name> "COM14" ("COM PORT")
      w253 = u16 0 items=["None", "XON/XOFF", "RTS/CTS", "XON/XOFF & RTS/CTS", "DTR/DSR", "XON/XOFF & DTR/DSR"] ("flow control (0:none)")
      w252 = u16 10 items=["1.0"=10, "1.5"=15, "2.0"=20] ("stop bits (10: 1 bit)")
      # "Stop bits"
      n97 = call-poly "VISA Configure Serial Port"("VISA resource name"=w255, "timeout (10sec)"=u32 10000, "baud rate (9600)"=u32 9600, "data bits (8)"=u16 8, "parity (0:none)"=enum16{"None", "Odd", "Even", "Mark", "Space"}."None", "stop bits (10: 1 bit)"=w252, "flow control (0:none)"=w253) -> ("VISA resource name out"=w248:refnum<visa-resource-name>, "error out"=w247:errorcluster)  [unwired: 7 in]
      "Y COM PORT" <- w255
    }
    frame #5 {
      n98 = property on="Y Run Current %" class="DigNum (strict)"() -> ("Value"=w263:i32)  [unwired: 2 in, 2 out]
      n99 = Divide(x=w263, y=100) -> (x/y=w264:dbl)
      n100 = Multiply(x=w264, y=3.5) -> (x*y=w258:dbl)
      n101 = Number To Fractional String(number=w258) -> (F-format string=w265:string)  [unwired: 3 in]
      n102 = call "Applied Send Command.vi"("error in (no error)"=w261, "Extra"=w265, "Command"=T1."Change Current", "VISA resource name"=w262) -> ("error out"=w259:errorcluster, "VISA resource name out"=w260:refnum<visa-resource-name>)  [unwired: 3 in, 1 out]
    }
    frame #6 {
      # "VELOCITY"
      n103 = property on="Y steps/rev" class="DigNum (strict)"() -> ("Value"=w274:u32)  [unwired: 2 in, 2 out]
      n104 = property on="Y Velocity SP step/sec" class="DigNum (strict)"() -> ("Value"=w271:i32)  [unwired: 2 in, 2 out]
      n105 = Divide(x=w271, y=w274) -> (x/y=w273:dbl)
      n106 = Number To Fractional String(number=w273) -> (F-format string=w277:string)  [unwired: 3 in]
      n107 = call "Applied Send Command.vi"("error in (no error)"=w269, "Extra"=w277, "Command"=T1."Velocity Setting", "VISA resource name"=w270) -> ("error out"=w278:errorcluster, "VISA resource name out"=w285:refnum<visa-resource-name>)  [unwired: 3 in, 1 out]
      n108 = call "Time Delay36"("error in (no error)"=w278, "Delay Time (s)"=0.1) -> ("error out"=w283:errorcluster)  [unwired: 9 in]
      n109 = call "Applied Send Command.vi"("error in (no error)"=w283, "Extra"="", "Command"=T1."Velocity Setting", "VISA resource name"=w285) -> ("error out"=w267:errorcluster, "read buffer"=w281:string, "VISA resource name out"=w268:refnum<visa-resource-name>)  [unwired: 3 in]
      n110 = Fract/Exp String To Number(string=w281, offset=3) -> (number=w276:dbl)  [unwired: 2 in, 1 out]
      n111 = Multiply(x=w276, y=w274) -> (x*y=w275:dbl)
      n112 = property on="Y velocity PV step/sec" class="DigNum (strict)"("Val(Sgnl)"=w275) -> ()  [unwired: 2 in, 2 out]
    }
    frame #7 {
      # "GET CURRENT POSITION"
      n113 = call "Applied Send Command.vi"("error in (no error)"=w289, "Extra"="", "Command"=T1."Immediate Position?", "VISA resource name"=w290) -> ("error out"=w292:errorcluster, "read buffer"=w294:string, "VISA resource name out"=w288:refnum<visa-resource-name>)  [unwired: 3 in]
      n114 = call "Time Delay37"("error in (no error)"=w292, "Delay Time (s)"=0.1) -> ("error out"=w287:errorcluster)  [unwired: 9 in]
      n115 = Hexadecimal String To Number(string=w294, offset=3) -> (number=w286:u32)  [unwired: 1 in, 1 out]
    }
    frame #8 {
      n116 = property on="Y Step SP" class="DigNum (strict)"() -> ("Maximum"=w298:dbl)  [unwired: 2 in, 2 out]
      n117 = property on="Y Step SP" class="DigNum (strict)"("Val(Sgnl)"=w300) -> ()  [unwired: 2 in, 2 out]
      n118 = property on="Y Step SP" class="DigNum (strict)"() -> ("Minimum"=w297:dbl)  [unwired: 2 in, 2 out]
      n119 = In Range and Coerce(upper limit=w298, x=w300, lower limit=w297) -> (In Range?=w301:bool)  [unwired: 1 out]
      n120 = property on="Y in Range" class="Bool (strict)"("Val(Sgnl)"=w301) -> ()  [unwired: 2 in, 2 out]
    }
  }
  n121 = flat-sequence {
    tunnel: [w320] -> w23
    tunnel: [w319] -> w22
    tunnel: w23 -> [w337]
    tunnel: w22 -> [w336]
    tunnel: [w335] -> w21
    tunnel: [w334] -> w20
    tunnel: [w340] -> w73
    tunnel: w21 -> [w348]
    tunnel: w20 -> [w347]
    tunnel: [w341] -> w19
    tunnel: w73 -> [w362]
    tunnel: [w361] -> w67
    tunnel: [w359] -> w66
    tunnel: [w364] -> w65
    tunnel: w19 -> [w363]
    tunnel: [w373] -> w71
    tunnel: [w374] -> w72
    tunnel: w67 -> [w374]
    tunnel: w66 -> [w373]
    tunnel: w65 -> [w369]
    frame #0 {
      "X Run Current %" <- 100 ("Run Current %")
      "X Holding Current %" <- 50 ("Holding Current %")
    }
    frame #1 {
      "X Backlash steps/sec" <- 10000 ("Value (Signaling)")
      "X Backlash" <- 5000 ("Backlash2")
    }
    frame #2 {
      w309 = 0.21167 ("MM/rev")
      w312 = u32 20000 ("step/rev")
      w307 = 50000 ("Value (Signaling)")
      n122 = property on="X Velocity SP step/sec" class="DigNum (strict)"("Minimum"=1.0 ("Data Entry Limits:Minimum")) -> ()  [unwired: 2 in, 2 out]
      n123 = property on="X Velocity SP step/sec" class="DigNum (strict)"("Val(Sgnl)"=w307) -> ()  [unwired: 2 in, 2 out]
      n124 = property on="X Scan Velocity SP mm/sec" class="DigNum (strict)"("Val(Sgnl)"=0.1 ("Value (Signaling)")) -> ()  [unwired: 2 in, 2 out]
      n125 = To Double Precision Float(number=w307) -> (double precision float=w313:dbl)
      n126 = To Double Precision Float(number=w312) -> (double precision float=w311:dbl)
      n127 = property on="X Velocity SP step/sec" class="DigNum (strict)"("Maximum"=w313) -> ()  [unwired: 2 in, 2 out]
      n128 = Divide(x=w313, y=w311) -> (x/y=w308:dbl)
      n129 = Multiply(x=w308, y=w309) -> (x*y=w310:dbl)
      n130 = property on="X Velocity SP mm/sec" class="DigNum (strict)"("Val(Sgnl)"=w310) -> ()  [unwired: 2 in, 2 out]
      "X steps/rev" <- w312
      "X mm/rev" <- w309
    }
    frame #3 {
      w318 = -750000 ("lower limit")
      w317 = 750000 ("upper limit")
      n131 = property on="X Step SP" class="DigNum (strict)"("Minimum"=w318) -> ()  [unwired: 2 in, 2 out]
      n132 = property on="X Step SP" class="DigNum (strict)"("Maximum"=w317) -> ()  [unwired: 2 in, 2 out]
      "X offset mm" <- 0.0 ("offset")
      "X MAXPOS" <- w317
      "X MINPOS" <- w318
    }
    frame #4 {
      w327 = refnum<visa-resource-name> "COM13" ("COM PORT")
      w325 = u16 0 items=["None", "XON/XOFF", "RTS/CTS", "XON/XOFF & RTS/CTS", "DTR/DSR", "XON/XOFF & DTR/DSR"] ("flow control (0:none)")
      w324 = u16 10 items=["1.0"=10, "1.5"=15, "2.0"=20] ("stop bits (10: 1 bit)")
      # "Stop bits"
      n133 = call-poly "VISA Configure Serial Port"("VISA resource name"=w327, "timeout (10sec)"=u32 10000, "baud rate (9600)"=u32 9600, "data bits (8)"=u16 8, "parity (0:none)"=enum16{"None", "Odd", "Even", "Mark", "Space"}."None", "stop bits (10: 1 bit)"=w324, "flow control (0:none)"=w325) -> ("VISA resource name out"=w320:refnum<visa-resource-name>, "error out"=w319:errorcluster)  [unwired: 7 in]
      "X COM PORT" <- w327
    }
    frame #5 {
      n134 = property on="X Run Current" class="DigNum (strict)"() -> ("Value"=w332:i32)  [unwired: 2 in, 2 out]
      n135 = Divide(x=w332, y=100) -> (x/y=w329:dbl)
      n136 = Multiply(x=3.5 ("y"), y=w329) -> (x*y=w331:dbl)
      n137 = Number To Fractional String(number=w331) -> (F-format string=w333:string)  [unwired: 3 in]
      n138 = call "Applied Send Command.vi"("error in (no error)"=w336, "Extra"=w333, "Command"=T1."Change Current", "VISA resource name"=w337) -> ("error out"=w335:errorcluster, "VISA resource name out"=w334:refnum<visa-resource-name>)  [unwired: 3 in, 1 out]
    }
    frame #6 {
      # "VELOCITY"
      n139 = property on="X steps/rev" class="DigNum (strict)"() -> ("Value"=w343:u32)  [unwired: 2 in, 2 out]
      n140 = property on="X Velocity SP step/sec" class="DigNum (strict)"() -> ("Value"=w344:i32)  [unwired: 2 in, 2 out]
      n141 = Divide(x=w344, y=w343) -> (x/y=w342:dbl)
      n142 = Number To Fractional String(number=w342) -> (F-format string=w349:string)  [unwired: 3 in]
      n143 = call "Applied Send Command.vi"("error in (no error)"=w348, "Extra"=w349, "Command"=T1."Velocity Setting", "VISA resource name"=w347) -> ("error out"=w350:errorcluster, "VISA resource name out"=w357:refnum<visa-resource-name>)  [unwired: 3 in, 1 out]
      n144 = call "Time Delay30"("error in (no error)"=w350, "Delay Time (s)"=0.1) -> ("error out"=w355:errorcluster)  [unwired: 9 in]
      n145 = call "Applied Send Command.vi"("error in (no error)"=w355, "Extra"="", "Command"=T1."Velocity Setting", "VISA resource name"=w357) -> ("error out"=w340:errorcluster, "read buffer"=w353:string, "VISA resource name out"=w341:refnum<visa-resource-name>)  [unwired: 3 in]
      n146 = Fract/Exp String To Number(string=w353, offset=3) -> (number=w346:dbl)  [unwired: 2 in, 1 out]
      n147 = Multiply(x=w346, y=w343) -> (x*y=w345:dbl)
      n148 = property on="X velocity PV step/sec" class="DigNum (strict)"("Val(Sgnl)"=w345) -> ()  [unwired: 2 in, 2 out]
    }
    frame #7 {
      # "GET CURRENT POSITION"
      n149 = call "Applied Send Command.vi"("error in (no error)"=w362, "Extra"="", "Command"=T1."Immediate Position?", "VISA resource name"=w363) -> ("error out"=w360:errorcluster, "read buffer"=w366:string, "VISA resource name out"=w361:refnum<visa-resource-name>)  [unwired: 3 in]
      n150 = call "Time Delay13"("error in (no error)"=w360, "Delay Time (s)"=0.1) -> ("error out"=w359:errorcluster)  [unwired: 9 in]
      n151 = Hexadecimal String To Number(string=w366, offset=3) -> (number=w364:u32)  [unwired: 1 in, 1 out]
    }
    frame #8 {
      n152 = property on="X Step SP" class="DigNum (strict)"() -> ("Maximum"=w372:dbl)  [unwired: 2 in, 2 out]
      n153 = property on="X Step SP" class="DigNum (strict)"("Val(Sgnl)"=w369) -> ()  [unwired: 2 in, 2 out]
      n154 = property on="X Step SP" class="DigNum (strict)"() -> ("Minimum"=w371:dbl)  [unwired: 2 in, 2 out]
      n155 = In Range and Coerce(upper limit=w372, x=w369, lower limit=w371) -> (In Range?=w370:bool)  [unwired: 1 out]
      n156 = property on="X  in Range" class="Bool (strict)"("Val(Sgnl)"=w370) -> ()  [unwired: 2 in, 2 out]
    }
  }
  n157 = call-poly <vilib>:"Read From Spreadsheet File.vi"("file path (dialog if empty)"=path "S:/LV codes/SCL2/POS.TXT") -> ("first row"=w42:i64[])  [unwired: 6 in, 4 out]
  n158 = call-poly <vilib>:"Read From Spreadsheet File.vi"("file path (dialog if empty)"=path "S:/LV codes/SCL2/PRESET.TXT") -> ("all rows"=w30:string[][])  [unwired: 6 in, 4 out]
  n159 = Array To Cluster(array=w42) -> (cluster=w41:T3)
  n160 = Transpose 2D Array(2D array=w30) -> (transposed array=w31:string[][])
  n161 = Unbundle(w41) -> ("first row[0]"=w39:i64, "first row[1]"=w38:i64, "first row[2]"=w37:i64, "first row[3]"=w36:i64)  [unwired: 5 out]
  n162 = Delete From Array(array=w31, index (row)=0) -> (deleted portion=w32:string[], array with subset deleted=w34:string[][])  [unwired: 2 in]
  n163 = property on="Reset X Motor Steps" class="DigNum (strict)"("Val(Sgnl)"=w39) -> ()  [unwired: 2 in, 2 out]
  n164 = property on="Reset Y Motor Steps" class="DigNum (strict)"("Val(Sgnl)"=w38) -> ()  [unwired: 2 in, 2 out]
  n165 = property on="Reset Z Motor Steps" class="DigNum (strict)"("Val(Sgnl)"=w37) -> ()  [unwired: 2 in, 2 out]
  n166 = property on="Reset R Motor Steps" class="DigNum (strict)"("Val(Sgnl)"=w36) -> ()  [unwired: 2 in, 2 out]
  n167 = Transpose 2D Array(2D array=w34) -> (transposed array=w35:string[][])
  n168 = property on="Preset positions" class="Ring (strict)"("Strings []"=w32) -> ()  [unwired: 2 in, 2 out]
  n169 = Decimal String To Number(string=w35) -> (number=w33:i32[][])  [unwired: 2 in, 1 out]
  n170 = Initialize Array(w24, w24, 4 ("dimension size")) -> (w27:i32[][])
  n171 = Build Array (concatenate)(w27, w33) -> (→"Presets":i32[][])
  n172 = while {
    tunnel: w75 -> [w393]
    tunnel: w74 -> [w396]
    tunnel: [w397] -> w49
    tunnel: [w395] -> w50
    tunnel: w72 -> [w392]
    tunnel: w71 -> [w391]
    tunnel: [w390] -> w70
    tunnel: [w389] -> w69
    tunnel: w56 -> [w388]
    tunnel: w55 -> [w387]
    tunnel: [w386] -> w52
    tunnel: [w385] -> w51
    tunnel: w54 -> [w384]
    tunnel: w53 -> [w383]
    tunnel: [w382] -> w48
    tunnel: [w381] -> w47
    stop <- "stop" stop-if-true
    n173 = flat-sequence {
      frame #0 {
      }
      frame #1 {
      }
    }
    n174 = flat-sequence {
      frame #0 {
      }
      frame #1 {
      }
    }
    n175 = property on="Preset positions" class="Ring (strict)"() -> ("Strings []"=w377:string[])  [unwired: 2 in, 2 out]
    n176 = event shown="[0] Timeout" {
      selector: _ -> [_ _ _ _ _ _ _ _ _ _ _ _ _ _ _ _ _ _ _ _ _ _ _ _ _]
      dyn-events: _ -> [_ _ _ _ _ _ _ _ _ _ _ _ _ _ _ _ _ _ _ _ _ _ _ _ _]
      timeout: 200 -> [_ _ _ _ _ _ _ _ _ _ _ _ _ _ _ _ _ _ _ _ _ _ _ _ _]
      tunnel: w396 -> [w507 _ _ _ _ _ _ _ _ _ _ _ w1237 _ _ _ _ w1530 _ _ w1634 w1650 w1694 w1782 w1927]
      tunnel: [w506 _ _ _ _ _ _ _ _ _ _ _ w1243 _ _ _ _ w1528 _ _ w1634 w1648 w1696 w1776 w1925] -> w397
      tunnel: w393 -> [w449 _ _ _ _ _ _ _ _ _ _ _ w1238 _ _ _ _ w1529 _ _ w1635 w1651 w1695 w1783 w1928]
      tunnel: [w505 _ _ _ _ _ _ _ _ _ _ _ w1244 _ _ _ _ w1525 _ _ w1635 w1649 w1697 w1777 w1926] -> w395
      tunnel: w392 -> [w448 _ _ _ _ _ _ _ _ _ _ _ _ _ _ w1431 w1491 _ _ _ _ w1645 w1687 w1785 w1924]
      tunnel: w391 -> [w482 _ _ _ _ _ _ _ _ _ _ _ _ _ _ w1430 w1490 _ _ _ _ w1644 w1686 w1784 w1923]
      tunnel: [w481 _ _ _ _ _ _ _ _ _ _ _ _ _ _ w1429 w1489 _ _ _ _ w1647 w1685 w1771 w1922] -> w390
      tunnel: [w480 _ _ _ _ _ _ _ _ _ _ _ _ _ _ w1428 w1488 _ _ _ _ w1646 w1684 w1770 w1921] -> w389
      tunnel: w388 -> [w454 _ _ _ _ _ _ _ _ _ _ _ _ w1300 _ _ _ _ w1563 _ _ w1643 w1681 w1781 w1920]
      tunnel: w387 -> [w457 _ _ _ _ _ _ _ _ _ _ _ _ w1299 _ _ _ _ w1562 _ _ w1642 w1680 w1780 w1919]
      tunnel: [w456 _ _ _ _ _ _ _ _ _ _ _ _ w1297 _ _ _ _ w1560 _ _ w1641 w1679 w1775 w1916] -> w386
      tunnel: [w455 _ _ _ _ _ _ _ _ _ _ _ _ w1298 _ _ _ _ w1561 _ _ w1640 w1678 w1774 w1915] -> w385
      tunnel: w384 -> [w453 _ _ _ _ _ _ _ _ _ _ _ _ _ w1364 _ _ _ _ w1600 _ w1639 w1675 w1779 w1918]
      tunnel: w383 -> [w452 _ _ _ _ _ _ _ _ _ _ _ _ _ w1363 _ _ _ _ w1599 _ w1638 w1674 w1778 w1917]
      tunnel: [w451 _ _ _ _ _ _ _ _ _ _ _ _ _ w1361 _ _ _ _ w1598 _ w1637 w1673 w1773 w1914] -> w382
      tunnel: [w450 _ _ _ _ _ _ _ _ _ _ _ _ _ w1362 _ _ _ _ w1597 _ w1636 w1672 w1772 w1913] -> w381
      event #0 {
        n177 = event-data() -> ()  [unwired: 1 in, 2 out]
        n178 = property on="X Step SP" class="DigNum (strict)"() -> ("Maximum"=w432:dbl)  [unwired: 2 in, 2 out]
        n179 = property on="Y Step SP" class="DigNum (strict)"() -> ("Maximum"=w437:dbl)  [unwired: 2 in, 2 out]
        n180 = flat-sequence {
          tunnel: [w616] -> w479
          tunnel: [w629] -> w478
          tunnel: [w639] -> w477
          tunnel: [w609] -> w476
          tunnel: w454 -> [w624]
          tunnel: w457 -> [w625]
          tunnel: w479 -> [w649]
          tunnel: [w649] -> w475
          tunnel: w478 -> [w648]
          tunnel: [w648] -> w474
          tunnel: w477 -> [w647]
          tunnel: [w647] -> w473
          tunnel: w476 -> [w644]
          tunnel: [w644] -> w472
          tunnel: w475 -> [w656]
          tunnel: [w657] -> w471
          tunnel: w474 -> [w659]
          tunnel: [w658] -> w470
          tunnel: w473 -> [w655]
          tunnel: [w654] -> w469
          tunnel: w472 -> [w654]
          tunnel: w471 -> [w669]
          tunnel: w470 -> [w670]
          tunnel: w469 -> [w672]
          tunnel: [w668] -> w455
          tunnel: [w667] -> w456
          frame #0 {
            w628 = 0.2 ("Delay Time (s)")
            n181 = property on="Z Step SP" class="DigNum (strict)"() -> ("Maximum"=w641:dbl)  [unwired: 2 in, 2 out]
            n182 = property on="Z Step SP" class="DigNum (strict)"() -> ("Minimum"=w643:dbl)  [unwired: 2 in, 2 out]
            n183 = property on="Z steps/rev" class="DigNum (strict)"() -> ("Value"=w637:u32)  [unwired: 2 in, 2 out]
            n184 = property on="Z offset mm" class="DigNum (strict)"() -> ("Value"=w633:dbl)  [unwired: 2 in, 2 out]
            n185 = To Long Integer(number=w641) -> (32bit integer=w640:i32)
            n186 = To Long Integer(number=w643) -> (32bit integer=w642:i32)
            n187 = To Double Precision Float(number=w637) -> (double precision float=w638:dbl)
            n188 = call "Applied Send Command.vi"("error in (no error)"=w625, "Command"=T1."Immediate Position?", "VISA resource name"=w624) -> ("error out"=w623:errorcluster, "read buffer"=w620:string, "VISA resource name out"=w618:refnum<visa-resource-name>)  [unwired: 4 in]
            n189 = call "Time Delay17"("error in (no error)"=w623, "Delay Time (s)"=w628) -> ("error out"=w608:errorcluster)  [unwired: 9 in]
            n190 = Hexadecimal String To Number(string=w620, offset=3) -> (number=w621:u32)  [unwired: 1 in, 1 out]
            n191 = To Long Integer(number=w621) -> (32bit integer=w631:i32)
            n192 = call "Applied Send Command.vi"("error in (no error)"=w608, "Command"=T1."Request Status", "VISA resource name"=w618) -> ("error out"=w617:errorcluster, "read buffer"=w613:string, "VISA resource name out"=w616:refnum<visa-resource-name>)  [unwired: 4 in]
            n193 = property on="Z Step PV" class="DigNum (strict)"("Val(Sgnl)"=w631) -> ()  [unwired: 2 in, 2 out]
            n194 = call "Time Delay16"("error in (no error)"=w617, "Delay Time (s)"=w628) -> ("error out"=w629:errorcluster)  [unwired: 9 in]
            n195 = String Subset(string=w613, offset (0)=0, length (rest)=1 ("length (rest)")) -> (substring=w610:string)
            n196 = In Range and Coerce(upper limit=w640, x=w631, lower limit=w642) -> (In Range?=w639:bool)  [unwired: 1 out]
            n197 = To Double Precision Float(number=w631) -> (double precision float=w632:dbl)
            n198 = Not Equal?(x=w610, y="R") -> (x != y?=w609:bool)
            n199 = Equal?(x=w610, y="R") -> (x = y?=w627:bool)
            n200 = property on="Z in Motion" class="Bool (strict)"("Val(Sgnl)"=w609) -> ()  [unwired: 2 in, 2 out]
            n201 = property on="Z in Range" class="Bool (strict)"("Val(Sgnl)"=w639) -> ()  [unwired: 2 in, 2 out]
            n202 = property on="Z Ready" class="Bool (strict)"("Val(Sgnl)"=w627) -> ()  [unwired: 2 in, 2 out]
            n203 = Divide(x=w632, y=w638) -> (x/y=w636:dbl)
            n204 = property on="Z mm/rev" class="DigNum (strict)"() -> ("Value"=w635:dbl)  [unwired: 2 in, 2 out]
            n205 = Multiply(x=w636, y=w635) -> (x*y=w634:dbl)
            n206 = Add(x=w634, y=w633) -> (x+y=w630:dbl)
            n207 = property on="Z Position mm PV" class="DigNum (strict)"("Val(Sgnl)"=w630) -> ()  [unwired: 2 in, 2 out]
          }
          frame #1 {
            n208 = property on="Z Scan" class="Bool (strict)"() -> ("Value"=w645:bool)  [unwired: 2 in, 2 out]
            n209 = Or(x=w644, y=w645) -> (x .or. y?=w646:bool)
            n210 = case shown="True" w646 {
              frame #0 {
                n211 = property on="Z Scan OK" class="Bool"("DisabledEnum"=T2."Enabled" ("Disabled")) -> ()  [unwired: 2 in, 2 out]
                n212 = property on="Z Go" class="Bool"("DisabledEnum"=T2."Enabled" ("Disabled")) -> ()  [unwired: 2 in, 2 out]
              }
              frame #1 {
                n213 = property on="Z Scan OK" class="Bool"("DisabledEnum"=T2."Disabled and Grayed Out" ("Disabled")) -> ()  [unwired: 2 in, 2 out]
                n214 = property on="Z Go" class="Bool"("DisabledEnum"=T2."Disabled and Grayed Out" ("Disabled")) -> ()  [unwired: 2 in, 2 out]
              }
            }
          }
          frame #2 {
            n215 = case shown="False" w655 {
              tunnel: w656 -> [w663 w666]
              tunnel: [w661 w666] -> w657
              tunnel: [w660 w665] -> w658
              tunnel: w659 -> [w662 w665]
              frame #0 {
                n216 = call "Applied Send Command.vi"("error in (no error)"=w662, "Command"=T1."Stop & Kill Buffer", "VISA resource name"=w663) -> ("error out"=w660:errorcluster, "VISA resource name out"=w661:refnum<visa-resource-name>)  [unwired: 4 in, 1 out]
              }
              frame #1 {
              }
            }
          }
          frame #3 {
            n217 = property on="Z Backlash corr" class="Bool (strict)"() -> ("Value"=w673:bool)  [unwired: 2 in, 2 out]
            n218 = Implies(1:w672, 2:w673) -> (0:w671:bool)
            n219 = case shown="False" w671 {
              tunnel: w670 -> [w674 w706]
              tunnel: w669 -> [w675 w707]
              tunnel: [w676 w706] -> w668
              tunnel: [w677 w707] -> w667
              frame #0 {
                w703 = 0.1 ("Delay Time (s)")
                # "Backlash"
                # "Backlash"
                n220 = property on="Z Backlash" class="DigNum (strict)"() -> ("Value"=w681:i32)  [unwired: 2 in, 2 out]
                n221 = To Long Integer(number=w681) -> (32bit integer=w684:i32)
                n222 = property on="Z Backlash corr" class="Bool (strict)"("Val(Sgnl)"=FALSE ("Value (Signaling)")) -> ()  [unwired: 2 in, 2 out]
                n223 = Number To Decimal String(number=w681) -> (decimal integer string=w689:string)  [unwired: 1 in]
                n224 = Negate(x=w684) -> (-x=w683:i32)
                n225 = property on="Z Backlash steps/sec" class="DigNum (strict)"() -> ("Value"=w680:i32)  [unwired: 2 in, 2 out]
                n226 = Number To Decimal String(number=w683) -> (decimal integer string=w690:string)  [unwired: 1 in]
                n227 = property on="Z steps/rev" class="DigNum (strict)"() -> ("Value"=w679:u32)  [unwired: 2 in, 2 out]
                n228 = Divide(x=w680, y=w679) -> (x/y=w704:dbl)
                n229 = Number To Fractional String(number=w704) -> (F-format string=w705:string)  [unwired: 3 in]
                n230 = call "Applied Send Command.vi"("error in (no error)"=w674, "Extra"=w705, "Command"=T1."Velocity Setting", "VISA resource name"=w675) -> ("error out"=w701:errorcluster, "VISA resource name out"=w694:refnum<visa-resource-name>)  [unwired: 3 in, 1 out]
                n231 = call "Time Delay47"("error in (no error)"=w701, "Delay Time (s)"=w703) -> ("error out"=w702:errorcluster)  [unwired: 9 in]
                n232 = call "Applied Send Command.vi"("error in (no error)"=w702, "Extra"=w689, "Command"=T1."Distance or Position", "VISA resource name"=w694) -> ("error out"=w695:errorcluster, "VISA resource name out"=w688:refnum<visa-resource-name>)  [unwired: 3 in, 1 out]
                n233 = call "Time Delay44"("error in (no error)"=w695, "Delay Time (s)"=w703) -> ("error out"=w696:errorcluster)  [unwired: 9 in]
                n234 = call "Applied Send Command.vi"("error in (no error)"=w696, "Command"=T1."Feed to Length", "VISA resource name"=w688) -> ("error out"=w697:errorcluster, "VISA resource name out"=w691:refnum<visa-resource-name>)  [unwired: 4 in, 1 out]
                n235 = call "Time Delay45"("error in (no error)"=w697, "Delay Time (s)"=w703) -> ("error out"=w698:errorcluster)  [unwired: 9 in]
                n236 = call "Applied Send Command.vi"("error in (no error)"=w698, "Extra"=w690, "Command"=T1."Distance or Position", "VISA resource name"=w691) -> ("error out"=w699:errorcluster, "VISA resource name out"=w692:refnum<visa-resource-name>)  [unwired: 3 in, 1 out]
                n237 = call "Time Delay46"("error in (no error)"=w699, "Delay Time (s)"=w703) -> ("error out"=w700:errorcluster)  [unwired: 9 in]
                n238 = call "Applied Send Command.vi"("error in (no error)"=w700, "Command"=T1."Feed to Length", "VISA resource name"=w692) -> ("error out"=w676:errorcluster, "VISA resource name out"=w677:refnum<visa-resource-name>)  [unwired: 4 in, 1 out]
              }
              frame #1 {
              }
            }
          }
        }
        n239 = flat-sequence {
          tunnel: [w517] -> w468
          tunnel: [w529] -> w467
          tunnel: [w539] -> w466
          tunnel: [w508] -> w465
          tunnel: w453 -> [w526]
          tunnel: w452 -> [w525]
          tunnel: w468 -> [w549]
          tunnel: [w549] -> w464
          tunnel: w467 -> [w548]
          tunnel: [w548] -> w463
          tunnel: w466 -> [w547]
          tunnel: [w547] -> w462
          tunnel: w465 -> [w544]
          tunnel: [w544] -> w461
          tunnel: w464 -> [w556]
          tunnel: [w557] -> w460
          tunnel: w463 -> [w559]
          tunnel: [w558] -> w459
          tunnel: w462 -> [w555]
          tunnel: [w554] -> w458
          tunnel: w461 -> [w554]
          tunnel: w460 -> [w569]
          tunnel: w459 -> [w570]
          tunnel: w458 -> [w572]
          tunnel: [w568] -> w450
          tunnel: [w567] -> w451
          frame #0 {
            w528 = 0.2 ("Delay Time (s)")
            n240 = property on="R Step SP" class="DigNum (strict)"() -> ("Maximum"=w541:dbl)  [unwired: 2 in, 2 out]
            n241 = property on="R Step SP" class="DigNum (strict)"() -> ("Minimum"=w543:dbl)  [unwired: 2 in, 2 out]
            n242 = property on="R steps/rev" class="DigNum (strict)"() -> ("Value"=w537:u32)  [unwired: 2 in, 2 out]
            n243 = property on="R offset deg" class="DigNum (strict)"() -> ("Value"=w533:dbl)  [unwired: 2 in, 2 out]
            n244 = To Long Integer(number=w541) -> (32bit integer=w540:i32)
            n245 = To Long Integer(number=w543) -> (32bit integer=w542:i32)
            n246 = To Double Precision Float(number=w537) -> (double precision float=w538:dbl)
            n247 = call "Applied Send Command.vi"("error in (no error)"=w525, "Command"=T1."Immediate Position?", "VISA resource name"=w526) -> ("error out"=w521:errorcluster, "read buffer"=w522:string, "VISA resource name out"=w519:refnum<visa-resource-name>)  [unwired: 4 in]
            n248 = call "Time Delay21"("error in (no error)"=w521, "Delay Time (s)"=w528) -> ("error out"=w518:errorcluster)  [unwired: 9 in]
            n249 = Hexadecimal String To Number(string=w522, offset=3) -> (number=w523:u32)  [unwired: 1 in, 1 out]
            n250 = To Long Integer(number=w523) -> (32bit integer=w531:i32)
            n251 = call "Applied Send Command.vi"("error in (no error)"=w518, "Command"=T1."Request Status", "VISA resource name"=w519) -> ("error out"=w516:errorcluster, "read buffer"=w513:string, "VISA resource name out"=w517:refnum<visa-resource-name>)  [unwired: 4 in]
            n252 = property on="R Step PV" class="DigNum (strict)"("Val(Sgnl)"=w531) -> ()  [unwired: 2 in, 2 out]
            n253 = call "Time Delay20"("error in (no error)"=w516, "Delay Time (s)"=w528) -> ("error out"=w529:errorcluster)  [unwired: 9 in]
            n254 = String Subset(string=w513, offset (0)=0, length (rest)=1 ("length (rest)")) -> (substring=w509:string)
            n255 = In Range and Coerce(upper limit=w540, x=w531, lower limit=w542) -> (In Range?=w539:bool)  [unwired: 1 out]
            n256 = To Double Precision Float(number=w531) -> (double precision float=w532:dbl)
            n257 = Not Equal?(x=w509, y="R") -> (x != y?=w508:bool)
            n258 = Equal?(x=w509, y="R") -> (x = y?=w510:bool)
            n259 = property on="R in Motion" class="Bool (strict)"("Val(Sgnl)"=w508) -> ()  [unwired: 2 in, 2 out]
            n260 = property on="R in Range" class="Bool (strict)"("Val(Sgnl)"=w539) -> ()  [unwired: 2 in, 2 out]
            n261 = property on="R Ready" class="Bool (strict)"("Val(Sgnl)"=w510) -> ()  [unwired: 2 in, 2 out]
            n262 = Divide(x=w532, y=w538) -> (x/y=w536:dbl)
            n263 = property on="R deg/rev" class="DigNum (strict)"() -> ("Value"=w535:dbl)  [unwired: 2 in, 2 out]
            n264 = Multiply(x=w536, y=w535) -> (x*y=w534:dbl)
            n265 = Add(x=w534, y=w533) -> (x+y=w530:dbl)
            n266 = property on="R Position deg PV" class="DigNum (strict)"("Val(Sgnl)"=w530) -> ()  [unwired: 2 in, 2 out]
          }
          frame #1 {
            n267 = property on="R Scan" class="Bool (strict)"() -> ("Value"=w545:bool)  [unwired: 2 in, 2 out]
            n268 = Or(x=w544, y=w545) -> (x .or. y?=w546:bool)
            n269 = case shown="True" w546 {
              frame #0 {
                n270 = property on="R Scan OK" class="Bool"("DisabledEnum"=T2."Enabled" ("Disabled")) -> ()  [unwired: 2 in, 2 out]
                n271 = property on="R Go" class="Bool"("DisabledEnum"=T2."Enabled" ("Disabled")) -> ()  [unwired: 2 in, 2 out]
              }
              frame #1 {
                n272 = property on="R Scan OK" class="Bool"("DisabledEnum"=T2."Disabled and Grayed Out" ("Disabled")) -> ()  [unwired: 2 in, 2 out]
                n273 = property on="R Go" class="Bool"("DisabledEnum"=T2."Disabled and Grayed Out" ("Disabled")) -> ()  [unwired: 2 in, 2 out]
              }
            }
          }
          frame #2 {
            n274 = case shown="False" w555 {
              tunnel: w556 -> [w563 w566]
              tunnel: [w561 w566] -> w557
              tunnel: [w560 w565] -> w558
              tunnel: w559 -> [w562 w565]
              frame #0 {
                n275 = call "Applied Send Command.vi"("error in (no error)"=w562, "Command"=T1."Stop & Kill Buffer", "VISA resource name"=w563) -> ("error out"=w560:errorcluster, "VISA resource name out"=w561:refnum<visa-resource-name>)  [unwired: 4 in, 1 out]
              }
              frame #1 {
              }
            }
          }
          frame #3 {
            n276 = property on="R Backlash corr" class="Bool (strict)"() -> ("Value"=w573:bool)  [unwired: 2 in, 2 out]
            n277 = Implies(1:w572, 2:w573) -> (0:w571:bool)
            n278 = case shown="False" w571 {
              tunnel: w570 -> [w577 w606]
              tunnel: w569 -> [w576 w607]
              tunnel: [w574 w606] -> w568
              tunnel: [w575 w607] -> w567
              frame #0 {
                w584 = 0.1 ("Delay Time (s)")
                # "Backlash"
                # "Backlash"
                n279 = property on="R Backlash" class="DigNum (strict)"() -> ("Value"=w578:i32)  [unwired: 2 in, 2 out]
                n280 = To Long Integer(number=w578) -> (32bit integer=w603:i32)
                n281 = property on="R Backlash corr" class="Bool (strict)"("Val(Sgnl)"=FALSE ("Value (Signaling)")) -> ()  [unwired: 2 in, 2 out]
                n282 = Number To Decimal String(number=w578) -> (decimal integer string=w598:string)  [unwired: 1 in]
                n283 = Negate(x=w603) -> (-x=w604:i32)
                n284 = property on="R Backlash steps/sec" class="DigNum (strict)"() -> ("Value"=w581:i32)  [unwired: 2 in, 2 out]
                n285 = Number To Decimal String(number=w604) -> (decimal integer string=w597:string)  [unwired: 1 in]
                n286 = property on="R steps/rev" class="DigNum (strict)"() -> ("Value"=w579:u32)  [unwired: 2 in, 2 out]
                n287 = Divide(x=w581, y=w579) -> (x/y=w580:dbl)
                n288 = Number To Fractional String(number=w580) -> (F-format string=w583:string)  [unwired: 3 in]
                n289 = call "Applied Send Command.vi"("error in (no error)"=w577, "Extra"=w583, "Command"=T1."Velocity Setting", "VISA resource name"=w576) -> ("error out"=w586:errorcluster, "VISA resource name out"=w593:refnum<visa-resource-name>)  [unwired: 3 in, 1 out]
                n290 = call "Time Delay49"("error in (no error)"=w586, "Delay Time (s)"=w584) -> ("error out"=w585:errorcluster)  [unwired: 9 in]
                n291 = call "Applied Send Command.vi"("error in (no error)"=w585, "Extra"=w598, "Command"=T1."Distance or Position", "VISA resource name"=w593) -> ("error out"=w592:errorcluster, "VISA resource name out"=w599:refnum<visa-resource-name>)  [unwired: 3 in, 1 out]
                n292 = call "Time Delay18"("error in (no error)"=w592, "Delay Time (s)"=w584) -> ("error out"=w591:errorcluster)  [unwired: 9 in]
                n293 = call "Applied Send Command.vi"("error in (no error)"=w591, "Command"=T1."Feed to Length", "VISA resource name"=w599) -> ("error out"=w590:errorcluster, "VISA resource name out"=w596:refnum<visa-resource-name>)  [unwired: 4 in, 1 out]
                n294 = call "Time Delay19"("error in (no error)"=w590, "Delay Time (s)"=w584) -> ("error out"=w589:errorcluster)  [unwired: 9 in]
                n295 = call "Applied Send Command.vi"("error in (no error)"=w589, "Extra"=w597, "Command"=T1."Distance or Position", "VISA resource name"=w596) -> ("error out"=w588:errorcluster, "VISA resource name out"=w595:refnum<visa-resource-name>)  [unwired: 3 in, 1 out]
                n296 = call "Time Delay48"("error in (no error)"=w588, "Delay Time (s)"=w584) -> ("error out"=w587:errorcluster)  [unwired: 9 in]
                n297 = call "Applied Send Command.vi"("error in (no error)"=w587, "Command"=T1."Feed to Length", "VISA resource name"=w595) -> ("error out"=w574:errorcluster, "VISA resource name out"=w575:refnum<visa-resource-name>)  [unwired: 4 in, 1 out]
              }
              frame #1 {
              }
            }
          }
        }
        n298 = property on="X Step SP" class="DigNum (strict)"() -> ("Minimum"=w433:dbl)  [unwired: 2 in, 2 out]
        n299 = property on="Y Step SP" class="DigNum (strict)"() -> ("Minimum"=w436:dbl)  [unwired: 2 in, 2 out]
        n300 = property on="X Step PV" class="DigNum (strict)"() -> ("Value"=w431:i32)  [unwired: 2 in, 2 out]
        n301 = property on="Y Step PV" class="DigNum (strict)"() -> ("Value"=w430:i32)  [unwired: 2 in, 2 out]
        n302 = Subtract(x=w432, y=w433) -> (x-y=w434:dbl)
        n303 = Absolute Value(x=w431) -> (abs(x)=w428:i32)
        n304 = Absolute Value(x=w430) -> (abs(x)=w429:i32)
        n305 = Subtract(x=w437, y=w436) -> (x-y=w438:dbl)
        n306 = property on="Y Scan Length SP steps" class="DigNum (strict)"() -> ("Value"=w440:i32)  [unwired: 2 in, 2 out]
        n307 = property on="Z Scan Length SP steps" class="DigNum (strict)"() -> ("Value"=w441:i32)  [unwired: 2 in, 2 out]
        n308 = Multiply(x=w428, y=w429) -> (x*y=w423:i32)
        n309 = Divide(x=w438, y=2.0) -> (x/y=w426:dbl)
        n310 = Divide(x=w434, y=2.0) -> (x/y=w427:dbl)
        n311 = Absolute Value(x=w426) -> (abs(x)=w424:dbl)
        n312 = Absolute Value(x=w427) -> (abs(x)=w425:dbl)
        n313 = Divide(x=w440, y=w441) -> (x/y=w442:dbl)
        n314 = Multiply(x=w424, y=w425) -> (x*y=w422:dbl)
        n315 = Inverse Tangent(1:w442) -> (0:w443:dbl)
        n316 = Less Or Equal?(x=w423, y=w422) -> (x <= y?=w421:bool)
        n317 = Divide(x=w443, y=6.283185307179586) -> (x/y=w444:dbl)
        n318 = flat-sequence {
          tunnel: [w720] -> w493
          tunnel: [w731] -> w492
          tunnel: [w709] -> w491
          tunnel: [w716] -> w490
          tunnel: w448 -> [w727]
          tunnel: w482 -> [w715]
          tunnel: w432 -> [w711]
          tunnel: w433 -> [w710]
          tunnel: w421 -> [w708]
          tunnel: w493 -> [w751]
          tunnel: [w751] -> w489
          tunnel: w492 -> [w750]
          tunnel: [w750] -> w488
          tunnel: w491 -> [w749]
          tunnel: [w749] -> w487
          tunnel: w490 -> [w746]
          tunnel: [w746] -> w486
          tunnel: w489 -> [w760]
          tunnel: [w757] -> w485
          tunnel: w488 -> [w759]
          tunnel: [w758] -> w484
          tunnel: w487 -> [w756]
          tunnel: [w761] -> w483
          tunnel: w486 -> [w761]
          tunnel: w485 -> [w772]
          tunnel: w484 -> [w773]
          tunnel: w483 -> [w774]
          tunnel: [w771] -> w480
          tunnel: [w770] -> w481
          frame #0 {
            w730 = 0.2 ("Delay Time (s)")
            n319 = To Long Integer(number=w711) -> (32bit integer=w743:i32)
            n320 = To Long Integer(number=w710) -> (32bit integer=w744:i32)
            n321 = property on="X steps/rev" class="DigNum (strict)"() -> ("Value"=w740:u32)  [unwired: 2 in, 2 out]
            n322 = property on="X offset mm" class="DigNum (strict)"() -> ("Value"=w736:dbl)  [unwired: 2 in, 2 out]
            n323 = To Double Precision Float(number=w740) -> (double precision float=w741:dbl)
            n324 = call "Applied Send Command.vi"("error in (no error)"=w715, "Command"=T1."Immediate Position?", "VISA resource name"=w727) -> ("error out"=w725:errorcluster, "read buffer"=w726:string, "VISA resource name out"=w721:refnum<visa-resource-name>)  [unwired: 4 in]
            n325 = call "Time Delay12"("error in (no error)"=w725, "Delay Time (s)"=w730) -> ("error out"=w718:errorcluster)  [unwired: 9 in]
            n326 = Hexadecimal String To Number(string=w726, offset=3) -> (number=w732:u32)  [unwired: 1 in, 1 out]
            n327 = To Long Integer(number=w732) -> (32bit integer=w734:i32)
            n328 = call "Applied Send Command.vi"("error in (no error)"=w718, "Command"=T1."Request Status", "VISA resource name"=w721) -> ("error out"=w719:errorcluster, "read buffer"=w723:string, "VISA resource name out"=w720:refnum<visa-resource-name>)  [unwired: 4 in]
            n329 = property on="X Step PV" class="DigNum (strict)"("Val(Sgnl)"=w734) -> ()  [unwired: 2 in, 2 out]
            n330 = call "Time Delay11"("error in (no error)"=w719, "Delay Time (s)"=w730) -> ("error out"=w731:errorcluster)  [unwired: 9 in]
            n331 = String Subset(string=w723, offset (0)=0, length (rest)=1 ("length (rest)")) -> (substring=w712:string)
            n332 = In Range and Coerce(upper limit=w743, x=w734, lower limit=w744) -> (In Range?=w742:bool)  [unwired: 1 out]
            n333 = To Double Precision Float(number=w734) -> (double precision float=w735:dbl)
            n334 = Not Equal?(x=w712, y="R") -> (x != y?=w716:bool)
            n335 = Equal?(x=w712, y="R") -> (x = y?=w729:bool)
            n336 = property on="X  in Motion" class="Bool (strict)"("Val(Sgnl)"=w716) -> ()  [unwired: 2 in, 2 out]
            n337 = property on="X Ready" class="Bool (strict)"("Val(Sgnl)"=w729) -> ()  [unwired: 2 in, 2 out]
            n338 = Divide(x=w735, y=w741) -> (x/y=w739:dbl)
            n339 = And(x=w708, y=w742) -> (x .and. y?=w709:bool)
            n340 = property on="X  in Range" class="Bool (strict)"("Val(Sgnl)"=w709) -> ()  [unwired: 2 in, 2 out]
            n341 = property on="X mm/rev" class="DigNum (strict)"() -> ("Value"=w738:dbl)  [unwired: 2 in, 2 out]
            n342 = Multiply(x=w739, y=w738) -> (x*y=w737:dbl)
            n343 = Add(x=w737, y=w736) -> (x+y=w733:dbl)
            n344 = property on="X Position mm PV" class="DigNum (strict)"("Val(Sgnl)"=w733) -> ()  [unwired: 2 in, 2 out]
          }
          frame #1 {
            n345 = property on="X Scan" class="Bool (strict)"() -> ("Value"=w747:bool)  [unwired: 2 in, 2 out]
            n346 = Or(x=w746, y=w747) -> (x .or. y?=w748:bool)
            n347 = case shown="True" w748 {
              frame #0 {
                n348 = property on="X Scan OK" class="Bool"("DisabledEnum"=T2."Enabled" ("Disabled")) -> ()  [unwired: 2 in, 2 out]
                n349 = property on="X Go" class="Bool"("DisabledEnum"=T2."Enabled" ("Disabled")) -> ()  [unwired: 2 in, 2 out]
              }
              frame #1 {
                n350 = property on="X Scan OK" class="Bool"("DisabledEnum"=T2."Disabled and Grayed Out" ("Disabled")) -> ()  [unwired: 2 in, 2 out]
                n351 = property on="X Go" class="Bool"("DisabledEnum"=T2."Disabled and Grayed Out" ("Disabled")) -> ()  [unwired: 2 in, 2 out]
              }
            }
          }
          frame #2 {
            n352 = case shown="False" w756 {
              tunnel: w760 -> [w763 w768]
              tunnel: [w765 w768] -> w757
              tunnel: [w766 w767] -> w758
              tunnel: w759 -> [w762 w767]
              frame #0 {
                n353 = call "Applied Send Command.vi"("error in (no error)"=w762, "Command"=T1."Stop & Kill Buffer", "VISA resource name"=w763) -> ("error out"=w766:errorcluster, "VISA resource name out"=w765:refnum<visa-resource-name>)  [unwired: 4 in, 1 out]
              }
              frame #1 {
              }
            }
          }
          frame #3 {
            n354 = property on="X Backlash corr" class="Bool (strict)"() -> ("Value"=w775:bool)  [unwired: 2 in, 2 out]
            n355 = Implies(1:w774, 2:w775) -> (0:w769:bool)
            n356 = case shown="False" w769 {
              tunnel: w773 -> [w789 w808]
              tunnel: w772 -> [w790 w809]
              tunnel: [w792 w808] -> w771
              tunnel: [w791 w809] -> w770
              frame #0 {
                w780 = 0.1 ("Delay Time (s)")
                # "Backlash"
                n357 = property on="X Backlash" class="DigNum (strict)"() -> ("Value"=w795:i32)  [unwired: 2 in, 2 out]
                n358 = To Long Integer(number=w795) -> (32bit integer=w804:i32)
                n359 = property on="X Backlash corr" class="Bool (strict)"("Val(Sgnl)"=FALSE ("Value (Signaling)")) -> ()  [unwired: 2 in, 2 out]
                n360 = Number To Decimal String(number=w795) -> (decimal integer string=w799:string)  [unwired: 1 in]
                n361 = Negate(x=w804) -> (-x=w805:i32)
                n362 = property on="X Backlash steps/sec" class="DigNum (strict)"() -> ("Value"=w779:i32)  [unwired: 2 in, 2 out]
                n363 = Number To Decimal String(number=w805) -> (decimal integer string=w798:string)  [unwired: 1 in]
                n364 = property on="X steps/rev" class="DigNum (strict)"() -> ("Value"=w778:u32)  [unwired: 2 in, 2 out]
                n365 = Divide(x=w779, y=w778) -> (x/y=w777:dbl)
                n366 = Number To Fractional String(number=w777) -> (F-format string=w776:string)  [unwired: 3 in]
                n367 = call "Applied Send Command.vi"("error in (no error)"=w789, "Extra"=w776, "Command"=T1."Velocity Setting", "VISA resource name"=w790) -> ("error out"=w782:errorcluster, "VISA resource name out"=w793:refnum<visa-resource-name>)  [unwired: 3 in, 1 out]
                n368 = call "Time Delay35"("error in (no error)"=w782, "Delay Time (s)"=w780) -> ("error out"=w781:errorcluster)  [unwired: 9 in]
                n369 = call "Applied Send Command.vi"("error in (no error)"=w781, "Extra"=w799, "Command"=T1."Distance or Position", "VISA resource name"=w793) -> ("error out"=w788:errorcluster, "VISA resource name out"=w800:refnum<visa-resource-name>)  [unwired: 3 in, 1 out]
                n370 = call "Time Delay32"("error in (no error)"=w788, "Delay Time (s)"=w780) -> ("error out"=w787:errorcluster)  [unwired: 9 in]
                n371 = call "Applied Send Command.vi"("error in (no error)"=w787, "Command"=T1."Feed to Length", "VISA resource name"=w800) -> ("error out"=w786:errorcluster, "VISA resource name out"=w797:refnum<visa-resource-name>)  [unwired: 4 in, 1 out]
                n372 = call "Time Delay33"("error in (no error)"=w786, "Delay Time (s)"=w780) -> ("error out"=w785:errorcluster)  [unwired: 9 in]
                n373 = call "Applied Send Command.vi"("error in (no error)"=w785, "Extra"=w798, "Command"=T1."Distance or Position", "VISA resource name"=w797) -> ("error out"=w784:errorcluster, "VISA resource name out"=w796:refnum<visa-resource-name>)  [unwired: 3 in, 1 out]
                n374 = call "Time Delay34"("error in (no error)"=w784, "Delay Time (s)"=w780) -> ("error out"=w783:errorcluster)  [unwired: 9 in]
                n375 = call "Applied Send Command.vi"("error in (no error)"=w783, "Command"=T1."Feed to Length", "VISA resource name"=w796) -> ("error out"=w792:errorcluster, "VISA resource name out"=w791:refnum<visa-resource-name>)  [unwired: 4 in, 1 out]
              }
              frame #1 {
              }
            }
          }
        }
        n376 = flat-sequence {
          tunnel: w507 -> [w826]
          tunnel: w449 -> [w827]
          tunnel: [w823] -> w504
          tunnel: [w833] -> w502
          tunnel: [w812] -> w500
          tunnel: [w814] -> w498
          tunnel: w437 -> [w813]
          tunnel: w436 -> [w810]
          tunnel: w421 -> [w811]
          tunnel: w504 -> [w853]
          tunnel: [w853] -> w503
          tunnel: w502 -> [w852]
          tunnel: [w852] -> w501
          tunnel: w500 -> [w851]
          tunnel: [w851] -> w499
          tunnel: w498 -> [w848]
          tunnel: [w848] -> w494
          tunnel: w503 -> [w860]
          tunnel: [w861] -> w497
          tunnel: w501 -> [w863]
          tunnel: [w862] -> w496
          tunnel: w499 -> [w859]
          tunnel: [w858] -> w495
          tunnel: w494 -> [w858]
          tunnel: w497 -> [w873]
          tunnel: w496 -> [w874]
          tunnel: w495 -> [w876]
          tunnel: [w872] -> w506
          tunnel: [w871] -> w505
          frame #0 {
            w832 = 0.2 ("Delay Time (s)")
            n377 = To Long Integer(number=w813) -> (32bit integer=w845:i32)
            n378 = To Long Integer(number=w810) -> (32bit integer=w846:i32)
            n379 = property on="Y steps/rev" class="DigNum (strict)"() -> ("Value"=w842:u32)  [unwired: 2 in, 2 out]
            n380 = property on="Y offset mm" class="DigNum (strict)"() -> ("Value"=w838:dbl)  [unwired: 2 in, 2 out]
            n381 = To Double Precision Float(number=w842) -> (double precision float=w843:dbl)
            n382 = call "Applied Send Command.vi"("error in (no error)"=w826, "Command"=T1."Immediate Position?", "VISA resource name"=w827) -> ("error out"=w829:errorcluster, "read buffer"=w830:string, "VISA resource name out"=w824:refnum<visa-resource-name>)  [unwired: 4 in]
            n383 = call "Time Delay4"("error in (no error)"=w829, "Delay Time (s)"=w832) -> ("error out"=w822:errorcluster)  [unwired: 9 in]
            n384 = Hexadecimal String To Number(string=w830, offset=3) -> (number=w834:u32)  [unwired: 1 in, 1 out]
            n385 = To Long Integer(number=w834) -> (32bit integer=w836:i32)
            n386 = call "Applied Send Command.vi"("error in (no error)"=w822, "Command"=T1."Request Status", "VISA resource name"=w824) -> ("error out"=w821:errorcluster, "read buffer"=w818:string, "VISA resource name out"=w823:refnum<visa-resource-name>)  [unwired: 4 in]
            n387 = property on="Y Step PV" class="DigNum (strict)"("Val(Sgnl)"=w836) -> ()  [unwired: 2 in, 2 out]
            n388 = call "Time Delay3"("error in (no error)"=w821, "Delay Time (s)"=w832) -> ("error out"=w833:errorcluster)  [unwired: 9 in]
            n389 = String Subset(string=w818, offset (0)=0, length (rest)=1 ("length (rest)")) -> (substring=w816:string)
            n390 = In Range and Coerce(upper limit=w845, x=w836, lower limit=w846) -> (In Range?=w844:bool)  [unwired: 1 out]
            n391 = To Double Precision Float(number=w836) -> (double precision float=w837:dbl)
            n392 = Not Equal?(x=w816, y="R") -> (x != y?=w814:bool)
            n393 = Equal?(x=w816, y="R") -> (x = y?=w831:bool)
            n394 = property on="Y in Motion" class="Bool (strict)"("Val(Sgnl)"=w814) -> ()  [unwired: 2 in, 2 out]
            n395 = property on="Y Ready" class="Bool (strict)"("Val(Sgnl)"=w831) -> ()  [unwired: 2 in, 2 out]
            n396 = Divide(x=w837, y=w843) -> (x/y=w841:dbl)
            n397 = And(x=w844, y=w811) -> (x .and. y?=w812:bool)
            n398 = property on="Y in Range" class="Bool (strict)"("Val(Sgnl)"=w812) -> ()  [unwired: 2 in, 2 out]
            n399 = property on="Y mm/rev" class="DigNum (strict)"() -> ("Value"=w840:dbl)  [unwired: 2 in, 2 out]
            n400 = Multiply(x=w841, y=w840) -> (x*y=w839:dbl)
            n401 = Add(x=w839, y=w838) -> (x+y=w835:dbl)
            n402 = property on="Y Position mm PV" class="DigNum (strict)"("Val(Sgnl)"=w835) -> ()  [unwired: 2 in, 2 out]
          }
          frame #1 {
            n403 = property on="Y Scan" class="Bool (strict)"() -> ("Value"=w849:bool)  [unwired: 2 in, 2 out]
            n404 = Or(x=w848, y=w849) -> (x .or. y?=w850:bool)
            n405 = case shown="True" w850 {
              frame #0 {
                n406 = property on="Y Scan OK" class="Bool"("DisabledEnum"=T2."Enabled" ("Disabled")) -> ()  [unwired: 2 in, 2 out]
                n407 = property on="Y Go" class="Bool"("DisabledEnum"=T2."Enabled" ("Disabled")) -> ()  [unwired: 2 in, 2 out]
              }
              frame #1 {
                n408 = property on="Y Scan OK" class="Bool"("DisabledEnum"=T2."Disabled and Grayed Out" ("Disabled")) -> ()  [unwired: 2 in, 2 out]
                n409 = property on="Y Go" class="Bool"("DisabledEnum"=T2."Disabled and Grayed Out" ("Disabled")) -> ()  [unwired: 2 in, 2 out]
              }
            }
          }
          frame #2 {
            n410 = case shown="False" w859 {
              tunnel: w860 -> [w865 w870]
              tunnel: [w867 w870] -> w861
              tunnel: [w866 w869] -> w862
              tunnel: w863 -> [w864 w869]
              frame #0 {
                n411 = call "Applied Send Command.vi"("error in (no error)"=w864, "Command"=T1."Stop & Kill Buffer", "VISA resource name"=w865) -> ("error out"=w866:errorcluster, "VISA resource name out"=w867:refnum<visa-resource-name>)  [unwired: 4 in, 1 out]
              }
              frame #1 {
              }
            }
          }
          frame #3 {
            n412 = property on="Y Backlash corr" class="Bool (strict)"() -> ("Value"=w877:bool)  [unwired: 2 in, 2 out]
            n413 = Implies(1:w876, 2:w877) -> (0:w875:bool)
            n414 = case shown="False" w875 {
              tunnel: w874 -> [w880 w909]
              tunnel: w873 -> [w881 w910]
              tunnel: [w878 w909] -> w872
              tunnel: [w879 w910] -> w871
              frame #0 {
                w887 = 0.1 ("Delay Time (s)")
                # "Backlash"
                n415 = property on="Y Backlash" class="DigNum (strict)"() -> ("Value"=w882:i32)  [unwired: 2 in, 2 out]
                n416 = To Long Integer(number=w882) -> (32bit integer=w905:i32)
                n417 = property on="Y Backlash corr" class="Bool (strict)"("Val(Sgnl)"=FALSE ("Value (Signaling)")) -> ()  [unwired: 2 in, 2 out]
                n418 = Number To Decimal String(number=w882) -> (decimal integer string=w900:string)  [unwired: 1 in]
                n419 = Negate(x=w905) -> (-x=w906:i32)
                n420 = property on="Y Backlash steps/sec" class="DigNum (strict)"() -> ("Value"=w883:i32)  [unwired: 2 in, 2 out]
                n421 = Number To Decimal String(number=w906) -> (decimal integer string=w899:string)  [unwired: 1 in]
                n422 = property on="Y steps/rev" class="DigNum (strict)"() -> ("Value"=w886:u32)  [unwired: 2 in, 2 out]
                n423 = Divide(x=w883, y=w886) -> (x/y=w885:dbl)
                n424 = Number To Fractional String(number=w885) -> (F-format string=w884:string)  [unwired: 3 in]
                n425 = call "Applied Send Command.vi"("error in (no error)"=w880, "Extra"=w884, "Command"=T1."Velocity Setting", "VISA resource name"=w881) -> ("error out"=w889:errorcluster, "VISA resource name out"=w895:refnum<visa-resource-name>)  [unwired: 3 in, 1 out]
                n426 = call "Time Delay41"("error in (no error)"=w889, "Delay Time (s)"=w887) -> ("error out"=w888:errorcluster)  [unwired: 9 in]
                n427 = call "Applied Send Command.vi"("error in (no error)"=w888, "Extra"=w900, "Command"=T1."Distance or Position", "VISA resource name"=w895) -> ("error out"=w894:errorcluster, "VISA resource name out"=w901:refnum<visa-resource-name>)  [unwired: 3 in, 1 out]
                n428 = call "Time Delay38"("error in (no error)"=w894, "Delay Time (s)"=w887) -> ("error out"=w893:errorcluster)  [unwired: 9 in]
                n429 = call "Applied Send Command.vi"("error in (no error)"=w893, "Command"=T1."Feed to Length", "VISA resource name"=w901) -> ("error out"=w892:errorcluster, "VISA resource name out"=w898:refnum<visa-resource-name>)  [unwired: 4 in, 1 out]
                n430 = call "Applied Send Command.vi"("Extra"=w899, "Command"=T1."Distance or Position", "VISA resource name"=w898) -> ("error out"=w891:errorcluster, "VISA resource name out"=w897:refnum<visa-resource-name>)  [unwired: 4 in, 1 out]
                n431 = call "Time Delay39"("error in (no error)"=w892, "Delay Time (s)"=w887) -> ()  [unwired: 9 in, 1 out]
                n432 = call "Time Delay40"("error in (no error)"=w891, "Delay Time (s)"=w887) -> ("error out"=w890:errorcluster)  [unwired: 9 in]
                n433 = call "Applied Send Command.vi"("error in (no error)"=w890, "Command"=T1."Feed to Length", "VISA resource name"=w897) -> ("error out"=w878:errorcluster, "VISA resource name out"=w879:refnum<visa-resource-name>)  [unwired: 4 in, 1 out]
              }
              frame #1 {
              }
            }
          }
        }
        n434 = Multiply(x=360.0, y=w444) -> (x*y=w447:dbl)
        n435 = property on="atan Y/Z" class="DigNum (strict)"("Val(Sgnl)"=w447) -> ()  [unwired: 2 in, 2 out]
      }
      event #1 {
        n436 = event-data() -> ()  [unwired: 1 in, 5 out]
        n437 = property on="Z steps/rev" class="DigNum (strict)"() -> ("Value"=w922:u32)  [unwired: 2 in, 2 out]
        n438 = property on="X steps/rev" class="DigNum (strict)"() -> ("Value"=w931:u32)  [unwired: 2 in, 2 out]
        n439 = property on="Y steps/rev" class="DigNum (strict)"() -> ("Value"=w940:u32)  [unwired: 2 in, 2 out]
        n440 = property on="R steps/rev" class="DigNum (strict)"() -> ("Value"=w913:u32)  [unwired: 2 in, 2 out]
        n441 = property on="R offset deg" class="DigNum (strict)"() -> ("Value"=w911:dbl)  [unwired: 2 in, 2 out]
        n442 = property on="Z offset mm" class="DigNum (strict)"() -> ("Value"=w920:dbl)  [unwired: 2 in, 2 out]
        n443 = property on="X offset mm" class="DigNum (strict)"() -> ("Value"=w929:dbl)  [unwired: 2 in, 2 out]
        n444 = property on="Y offset mm" class="DigNum (strict)"() -> ("Value"=w938:dbl)  [unwired: 2 in, 2 out]
        n445 = To Double Precision Float(number=w913) -> (double precision float=w916:dbl)
        n446 = To Double Precision Float(number=w931) -> (double precision float=w934:dbl)
        n447 = To Double Precision Float(number=w940) -> (double precision float=w943:dbl)
        n448 = property on="Reset Z Position mm" class="DigNum (strict)"() -> ("Value"=w928:dbl)  [unwired: 2 in, 2 out]
        n449 = property on="Reset X Position mm" class="DigNum (strict)"() -> ("Value"=w937:dbl)  [unwired: 2 in, 2 out]
        n450 = property on="Reset Y Position mm" class="DigNum (strict)"() -> ("Value"=w946:dbl)  [unwired: 2 in, 2 out]
        n451 = property on="Reset R Position deg" class="DigNum (strict)"() -> ("Value"=w919:dbl)  [unwired: 2 in, 2 out]
        n452 = Subtract(x=w928, y=w920) -> (x-y=w927:dbl)
        n453 = Subtract(x=w919, y=w911) -> (x-y=w918:dbl)
        n454 = Subtract(x=w937, y=w929) -> (x-y=w936:dbl)
        n455 = Subtract(x=w946, y=w938) -> (x-y=w945:dbl)
        n456 = property on="Z mm/rev" class="DigNum (strict)"() -> ("Value"=w921:dbl)  [unwired: 2 in, 2 out]
        n457 = property on="X mm/rev" class="DigNum (strict)"() -> ("Value"=w930:dbl)  [unwired: 2 in, 2 out]
        n458 = property on="Y mm/rev" class="DigNum (strict)"() -> ("Value"=w939:dbl)  [unwired: 2 in, 2 out]
        n459 = property on="R deg/rev" class="DigNum (strict)"() -> ("Value"=w912:dbl)  [unwired: 2 in, 2 out]
        n460 = Divide(x=w918, y=w912) -> (x/y=w917:dbl)
        n461 = Divide(x=w936, y=w930) -> (x/y=w935:dbl)
        n462 = Divide(x=w945, y=w939) -> (x/y=w944:dbl)
        n463 = Divide(x=w927, y=w921) -> (x/y=w926:dbl)
        n464 = To Double Precision Float(number=w922) -> (double precision float=w925:dbl)
        n465 = Multiply(x=w926, y=w925) -> (x*y=w924:dbl)
        n466 = Multiply(x=w917, y=w916) -> (x*y=w915:dbl)
        n467 = Multiply(x=w935, y=w934) -> (x*y=w933:dbl)
        n468 = Multiply(x=w944, y=w943) -> (x*y=w942:dbl)
        n469 = To Long Integer(number=w924) -> (32bit integer=w923:i32)
        n470 = To Long Integer(number=w915) -> (32bit integer=w914:i32)
        n471 = To Long Integer(number=w933) -> (32bit integer=w932:i32)
        n472 = To Long Integer(number=w942) -> (32bit integer=w941:i32)
        n473 = property on="Reset Z Motor Steps" class="DigNum (strict)"("Val(Sgnl)"=w923) -> ()  [unwired: 2 in, 2 out]
        n474 = property on="Reset R Motor Steps" class="DigNum (strict)"("Val(Sgnl)"=w914) -> ()  [unwired: 2 in, 2 out]
        n475 = property on="Reset X Motor Steps" class="DigNum (strict)"("Val(Sgnl)"=w932) -> ()  [unwired: 2 in, 2 out]
        n476 = property on="Reset Y Motor Steps" class="DigNum (strict)"("Val(Sgnl)"=w941) -> ()  [unwired: 2 in, 2 out]
      }
      event #2 {
        n477 = event-data() -> ()  [unwired: 1 in, 5 out]
        n478 = property on="Z Step SP" class="DigNum (strict)"() -> ("Value"=w963:i32)  [unwired: 2 in, 2 out]
        n479 = property on="Y Step SP" class="DigNum (strict)"() -> ("Value"=w979:i32)  [unwired: 2 in, 2 out]
        n480 = property on="X Step SP" class="DigNum (strict)"() -> ("Value"=w971:i32)  [unwired: 2 in, 2 out]
        n481 = property on="Z steps/rev" class="DigNum (strict)"() -> ("Value"=w990:u32)  [unwired: 2 in, 2 out]
        n482 = property on="Z steps/rev" class="DigNum (strict)"() -> ("Value"=w961:u32)  [unwired: 2 in, 2 out]
        n483 = property on="R Step SP" class="DigNum (strict)"() -> ("Value"=w955:i32)  [unwired: 2 in, 2 out]
        n484 = property on="Y steps/rev" class="DigNum (strict)"() -> ("Value"=w1002:u32)  [unwired: 2 in, 2 out]
        n485 = property on="Y steps/rev" class="DigNum (strict)"() -> ("Value"=w977:u32)  [unwired: 2 in, 2 out]
        n486 = property on="X steps/rev" class="DigNum (strict)"() -> ("Value"=w996:u32)  [unwired: 2 in, 2 out]
        n487 = property on="X steps/rev" class="DigNum (strict)"() -> ("Value"=w969:u32)  [unwired: 2 in, 2 out]
        n488 = property on="R steps/rev" class="DigNum (strict)"() -> ("Value"=w984:u32)  [unwired: 2 in, 2 out]
        n489 = property on="R steps/rev" class="DigNum (strict)"() -> ("Value"=w953:u32)  [unwired: 2 in, 2 out]
        n490 = property on="R offset deg" class="DigNum (strict)"() -> ("Value"=w952:dbl)  [unwired: 2 in, 2 out]
        n491 = property on="Z offset mm" class="DigNum (strict)"() -> ("Value"=w960:dbl)  [unwired: 2 in, 2 out]
        n492 = property on="Y offset mm" class="DigNum (strict)"() -> ("Value"=w976:dbl)  [unwired: 2 in, 2 out]
        n493 = property on="X offset mm" class="DigNum (strict)"() -> ("Value"=w968:dbl)  [unwired: 2 in, 2 out]
        n494 = To Double Precision Float(number=w990) -> (double precision float=w995:dbl)
        n495 = To Double Precision Float(number=w963) -> (double precision float=w964:dbl)
        n496 = To Double Precision Float(number=w961) -> (double precision float=w967:dbl)
        n497 = To Double Precision Float(number=w984) -> (double precision float=w989:dbl)
        n498 = To Double Precision Float(number=w955) -> (double precision float=w956:dbl)
        n499 = To Double Precision Float(number=w953) -> (double precision float=w959:dbl)
        n500 = To Double Precision Float(number=w979) -> (double precision float=w980:dbl)
        n501 = To Double Precision Float(number=w977) -> (double precision float=w983:dbl)
        n502 = To Double Precision Float(number=w996) -> (double precision float=w1001:dbl)
        n503 = To Double Precision Float(number=w971) -> (double precision float=w972:dbl)
        n504 = To Double Precision Float(number=w969) -> (double precision float=w975:dbl)
        n505 = Divide(x=w964, y=w967) -> (x/y=w966:dbl)
        n506 = Divide(x=w980, y=w983) -> (x/y=w982:dbl)
        n507 = Divide(x=w972, y=w975) -> (x/y=w974:dbl)
        n508 = Divide(x=w956, y=w959) -> (x/y=w958:dbl)
        n509 = property on="Z Velocity SP step/sec" class="DigNum (strict)"() -> ("Value"=w992:i32)  [unwired: 2 in, 2 out]
        n510 = property on="Z mm/rev" class="DigNum (strict)"() -> ("Value"=w950:dbl)  [unwired: 2 in, 2 out]
        n511 = property on="Y Velocity SP step/sec" class="DigNum (strict)"() -> ("Value"=w1004:i32)  [unwired: 2 in, 2 out]
        n512 = property on="Y mm/rev" class="DigNum (strict)"() -> ("Value"=w948:dbl)  [unwired: 2 in, 2 out]
        n513 = property on="X Velocity SP step/sec" class="DigNum (strict)"() -> ("Value"=w998:i32)  [unwired: 2 in, 2 out]
        n514 = property on="X mm/rev" class="DigNum (strict)"() -> ("Value"=w949:dbl)  [unwired: 2 in, 2 out]
        n515 = property on="R Velocity SP step/sec" class="DigNum (strict)"() -> ("Value"=w986:i32)  [unwired: 2 in, 2 out]
        n516 = property on="R deg/rev" class="DigNum (strict)"() -> ("Value"=w951:dbl)  [unwired: 2 in, 2 out]
        n517 = Multiply(x=w966, y=w950) -> (x*y=w965:dbl)
        n518 = Multiply(x=w958, y=w951) -> (x*y=w957:dbl)
        n519 = Multiply(x=w982, y=w948) -> (x*y=w981:dbl)
        n520 = Multiply(x=w974, y=w949) -> (x*y=w973:dbl)
        n521 = To Double Precision Float(number=w992) -> (double precision float=w993:dbl)
        n522 = To Double Precision Float(number=w986) -> (double precision float=w987:dbl)
        n523 = To Double Precision Float(number=w1004) -> (double precision float=w1005:dbl)
        n524 = To Double Precision Float(number=w1002) -> (double precision float=w1007:dbl)
        n525 = To Double Precision Float(number=w998) -> (double precision float=w999:dbl)
        n526 = Divide(x=w993, y=w995) -> (x/y=w994:dbl)
        n527 = Add(x=w965, y=w960) -> (x+y=w962:dbl)
        n528 = Divide(x=w987, y=w989) -> (x/y=w988:dbl)
        n529 = Add(x=w957, y=w952) -> (x+y=w954:dbl)
        n530 = Divide(x=w1005, y=w1007) -> (x/y=w1006:dbl)
        n531 = Add(x=w981, y=w976) -> (x+y=w978:dbl)
        n532 = Divide(x=w999, y=w1001) -> (x/y=w1000:dbl)
        n533 = Add(x=w973, y=w968) -> (x+y=w970:dbl)
        n534 = Multiply(x=w994, y=w950) -> (x*y=w991:dbl)
        n535 = Multiply(x=w988, y=w951) -> (x*y=w985:dbl)
        n536 = Multiply(x=w1006, y=w948) -> (x*y=w1003:dbl)
        n537 = Multiply(x=w1000, y=w949) -> (x*y=w997:dbl)
        n538 = property on="Z Position MV mm" class="DigNum (strict)"("Val(Sgnl)"=w962) -> ()  [unwired: 2 in, 2 out]
        n539 = property on="R Position MV deg" class="DigNum (strict)"("Val(Sgnl)"=w954) -> ()  [unwired: 2 in, 2 out]
        n540 = property on="Y Position MV mm" class="DigNum (strict)"("Val(Sgnl)"=w978) -> ()  [unwired: 2 in, 2 out]
        n541 = property on="X Position MV mm" class="DigNum (strict)"("Val(Sgnl)"=w970) -> ()  [unwired: 2 in, 2 out]
        n542 = property on="Z Velocity MV mm/sec" class="DigNum (strict)"("Val(Sgnl)"=w991) -> ()  [unwired: 2 in, 2 out]
        n543 = property on="Y Velocity MV mm/sec" class="DigNum (strict)"("Val(Sgnl)"=w1003) -> ()  [unwired: 2 in, 2 out]
        n544 = property on="X Velocity MV mm/sec" class="DigNum (strict)"("Val(Sgnl)"=w997) -> ()  [unwired: 2 in, 2 out]
        n545 = Absolute Value(x=w985) -> (abs(x)=w947:dbl)
        n546 = property on="R Velocity MVdeg/sec" class="DigNum (strict)"("Val(Sgnl)"=w947) -> ()  [unwired: 2 in, 2 out]
      }
      event #3 {
        n547 = event-data() -> ()  [unwired: 1 in, 5 out]
        n548 = property on="R Step PV" class="DigNum (strict)"() -> ("Value"=w1035:i32)  [unwired: 2 in, 2 out]
        n549 = property on="Z steps/rev" class="DigNum (strict)"() -> ("Value"=w1051:u32)  [unwired: 2 in, 2 out]
        n550 = property on="X steps/rev" class="DigNum (strict)"() -> ("Value"=w1078:u32)  [unwired: 2 in, 2 out]
        n551 = property on="Y steps/rev" class="DigNum (strict)"() -> ("Value"=w1064:u32)  [unwired: 2 in, 2 out]
        n552 = property on="X Step PV" class="DigNum (strict)"() -> ("Value"=w1076:i32)  [unwired: 2 in, 2 out]
        n553 = property on="Y Step PV" class="DigNum (strict)"() -> ("Value"=w1062:i32)  [unwired: 2 in, 2 out]
        n554 = property on="Z Step PV" class="DigNum (strict)"() -> ("Value"=w1049:i32)  [unwired: 2 in, 2 out]
        n555 = property on="R steps/rev" class="DigNum (strict)"() -> ("Value"=w1037:u32)  [unwired: 2 in, 2 out]
        n556 = To Double Precision Float(number=w1076) -> (double precision float=w1029:dbl)
        n557 = To Double Precision Float(number=w1062) -> (double precision float=w1028:dbl)
        n558 = To Double Precision Float(number=w1049) -> (double precision float=w1027:dbl)
        n559 = To Double Precision Float(number=w1035) -> (double precision float=w1026:dbl)
        n560 = To Double Precision Float(number=w1051) -> (double precision float=w1048:dbl)
        n561 = To Double Precision Float(number=w1037) -> (double precision float=w1034:dbl)
        n562 = To Double Precision Float(number=w1078) -> (double precision float=w1075:dbl)
        n563 = To Double Precision Float(number=w1064) -> (double precision float=w1019:dbl)
        n564 = property on="X Step SP" class="DigNum (strict)"() -> ("Maximum"=w1082:dbl)  [unwired: 2 in, 2 out]
        n565 = property on="Y Step SP" class="DigNum (strict)"() -> ("Maximum"=w1068:dbl)  [unwired: 2 in, 2 out]
        n566 = property on="Z Step SP" class="DigNum (strict)"() -> ("Maximum"=w1055:dbl)  [unwired: 2 in, 2 out]
        n567 = property on="R Step SP" class="DigNum (strict)"() -> ("Maximum"=w1043:dbl)  [unwired: 2 in, 2 out]
        n568 = property on="Z Scan Length SP steps" class="DigNum (strict)"() -> ("Value"=w1052:i32)  [unwired: 2 in, 2 out]
        n569 = property on="X Scan Length SP steps" class="DigNum (strict)"() -> ("Value"=w1074:i32)  [unwired: 2 in, 2 out]
        n570 = property on="Y Scan Length SP steps" class="DigNum (strict)"() -> ("Value"=w1065:i32)  [unwired: 2 in, 2 out]
        n571 = property on="R Scan Length SP steps" class="DigNum (strict)"() -> ("Value"=w1038:i32)  [unwired: 2 in, 2 out]
        n572 = property on="X Step SP" class="DigNum (strict)"() -> ("Minimum"=w1083:dbl)  [unwired: 2 in, 2 out]
        n573 = property on="Y Step SP" class="DigNum (strict)"() -> ("Minimum"=w1069:dbl)  [unwired: 2 in, 2 out]
        n574 = property on="Z Step SP" class="DigNum (strict)"() -> ("Minimum"=w1056:dbl)  [unwired: 2 in, 2 out]
        n575 = property on="R Step SP" class="DigNum (strict)"() -> ("Minimum"=w1040:dbl)  [unwired: 2 in, 2 out]
        n576 = property on="Z Scan Velocity SP steps/sec" class="DigNum (strict)"() -> ("Value"=w1047:i32)  [unwired: 2 in, 2 out]
        n577 = property on="R Scan Velocity SP steps/sec" class="DigNum (strict)"() -> ("Value"=w1033:i32)  [unwired: 2 in, 2 out]
        n578 = property on="X Scan Velocity SP steps/sec" class="DigNum (strict)"() -> ("Value"=w1079:i32)  [unwired: 2 in, 2 out]
        n579 = property on="Y Scan Velocity SP steps/sec" class="DigNum (strict)"() -> ("Value"=w1061:i32)  [unwired: 2 in, 2 out]
        n580 = Subtract(x=w1083, y=w1029) -> (x-y=w1084:dbl)
        n581 = Subtract(x=w1082, y=w1029) -> (x-y=w1081:dbl)
        n582 = Subtract(x=w1069, y=w1028) -> (x-y=w1070:dbl)
        n583 = Subtract(x=w1068, y=w1028) -> (x-y=w1067:dbl)
        n584 = Subtract(x=w1056, y=w1027) -> (x-y=w1057:dbl)
        n585 = Subtract(x=w1055, y=w1027) -> (x-y=w1054:dbl)
        n586 = Subtract(x=w1040, y=w1026) -> (x-y=w1041:dbl)
        n587 = Subtract(x=w1043, y=w1026) -> (x-y=w1042:dbl)
        n588 = To Double Precision Float(number=w1052) -> (double precision float=w1025:dbl)
        n589 = To Double Precision Float(number=w1038) -> (double precision float=w1023:dbl)
        n590 = To Double Precision Float(number=w1074) -> (double precision float=w1014:dbl)
        n591 = To Double Precision Float(number=w1065) -> (double precision float=w1018:dbl)
        n592 = property on="X Scan Length SP steps" class="DigNum (strict)"("Minimum"=w1084) -> ()  [unwired: 2 in, 2 out]
        n593 = property on="X Scan Length SP steps" class="DigNum (strict)"("Maximum"=w1081) -> ()  [unwired: 2 in, 2 out]
        n594 = property on="Y Scan Length SP steps" class="DigNum (strict)"("Minimum"=w1070) -> ()  [unwired: 2 in, 2 out]
        n595 = property on="Y Scan Length SP steps" class="DigNum (strict)"("Maximum"=w1067) -> ()  [unwired: 2 in, 2 out]
        n596 = property on="Z Scan Length SP steps" class="DigNum (strict)"("Minimum"=w1057) -> ()  [unwired: 2 in, 2 out]
        n597 = property on="Z Scan Length SP steps" class="DigNum (strict)"("Maximum"=w1054) -> ()  [unwired: 2 in, 2 out]
        n598 = property on="R Scan Length SP steps" class="DigNum (strict)"("Minimum"=w1041) -> ()  [unwired: 2 in, 2 out]
        n599 = property on="R Scan Length SP steps" class="DigNum (strict)"("Maximum"=w1042) -> ()  [unwired: 2 in, 2 out]
        n600 = Divide(x=w1025, y=w1048) -> (x/y=w1053:dbl)
        n601 = Divide(x=w1014, y=w1075) -> (x/y=w1073:dbl)
        n602 = Divide(x=w1018, y=w1019) -> (x/y=w1066:dbl)
        n603 = Divide(x=w1023, y=w1034) -> (x/y=w1039:dbl)
        n604 = To Double Precision Float(number=w1047) -> (double precision float=w1024:dbl)
        n605 = To Double Precision Float(number=w1079) -> (double precision float=w1013:dbl)
        n606 = To Double Precision Float(number=w1061) -> (double precision float=w1017:dbl)
        n607 = To Double Precision Float(number=w1033) -> (double precision float=w1022:dbl)
        n608 = property on="Z mm/rev" class="DigNum (strict)"() -> ("Value"=w1050:dbl)  [unwired: 2 in, 2 out]
        n609 = property on="X mm/rev" class="DigNum (strict)"() -> ("Value"=w1077:dbl)  [unwired: 2 in, 2 out]
        n610 = property on="Y mm/rev" class="DigNum (strict)"() -> ("Value"=w1063:dbl)  [unwired: 2 in, 2 out]
        n611 = property on="R deg/rev" class="DigNum (strict)"() -> ("Value"=w1036:dbl)  [unwired: 2 in, 2 out]
        n612 = Multiply(x=w1053, y=w1050) -> (x*y=w1045:dbl)
        n613 = Divide(x=w1025, y=w1024) -> (x/y=w1020:dbl)
        n614 = Divide(x=w1024, y=w1048) -> (x/y=w1046:dbl)
        n615 = Multiply(x=w1039, y=w1036) -> (x*y=w1031:dbl)
        n616 = Divide(x=w1023, y=w1022) -> (x/y=w1021:dbl)
        n617 = Divide(x=w1022, y=w1034) -> (x/y=w1032:dbl)
        n618 = Multiply(x=w1077, y=w1073) -> (x*y=w1071:dbl)
        n619 = Divide(x=w1014, y=w1013) -> (x/y=w1015:dbl)
        n620 = Divide(x=w1013, y=w1075) -> (x/y=w1080:dbl)
        n621 = Multiply(x=w1066, y=w1063) -> (x*y=w1059:dbl)
        n622 = Divide(x=w1018, y=w1017) -> (x/y=w1016:dbl)
        n623 = Divide(x=w1017, y=w1019) -> (x/y=w1060:dbl)
        n624 = Multiply(x=w1050, y=w1046) -> (x*y=w1044:dbl)
        n625 = Multiply(x=w1036, y=w1032) -> (x*y=w1030:dbl)
        n626 = Multiply(x=w1080, y=w1077) -> (x*y=w1072:dbl)
        n627 = Multiply(x=w1063, y=w1060) -> (x*y=w1058:dbl)
        n628 = Absolute Value(x=w1020) -> (abs(x)=→"Z Scan Duration":dbl)
        n629 = Absolute Value(x=w1021) -> (abs(x)=→"R Scan Duration":dbl)
        n630 = Absolute Value(x=w1015) -> (abs(x)=→"X Scan Duration":dbl)
        n631 = Absolute Value(x=w1016) -> (abs(x)=→"Y Scan Duration":dbl)
        n632 = property on="Z Scan length MV mm" class="DigNum (strict)"("Value"=w1045) -> ()  [unwired: 2 in, 2 out]
        n633 = property on="R Scan length MV deg" class="DigNum (strict)"("Value"=w1031) -> ()  [unwired: 2 in, 2 out]
        n634 = property on="X Scan length MV mm" class="DigNum (strict)"("Val(Sgnl)"=w1071) -> ()  [unwired: 2 in, 2 out]
        n635 = property on="Y Scan length MV mm" class="DigNum (strict)"("Value"=w1059) -> ()  [unwired: 2 in, 2 out]
        n636 = Absolute Value(x=w1030) -> (abs(x)=w1012:dbl)
        n637 = property on="Z Scan velocity MV mm/sec" class="DigNum (strict)"("Val(Sgnl)"=w1044) -> ()  [unwired: 2 in, 2 out]
        n638 = property on="X Scan velocity MV mm/sec" class="DigNum (strict)"("Value"=w1072) -> ()  [unwired: 2 in, 2 out]
        n639 = property on="Y Scan velocity MV mm/sec" class="DigNum (strict)"("Val(Sgnl)"=w1058) -> ()  [unwired: 2 in, 2 out]
        n640 = property on="R Scan Velocity SP deg/sec" class="DigNum (strict)"("Val(Sgnl)"=w1012) -> ()  [unwired: 2 in, 2 out]
      }
      event #4 {
        n641 = event-data() -> ()  [unwired: 1 in, 7 out]
        n642 = property on="Y steps/rev" class="DigNum (strict)"() -> ("Value"=w1101:u32)  [unwired: 2 in, 2 out]
        n643 = property on="Y offset mm" class="DigNum (strict)"() -> ("Value"=w1099:dbl)  [unwired: 2 in, 2 out]
        n644 = property on="Y Position SP mm" class="DigNum (strict)"() -> ("Value"=w1098:dbl)  [unwired: 2 in, 2 out]
        n645 = property on="Y Velocity SP step/sec" class="DigNum (strict)"() -> ("Maximum"=w1088:dbl)  [unwired: 2 in, 2 out]
        n646 = property on="Y Velocity SP step/sec" class="DigNum (strict)"() -> ("Minimum"=w1087:dbl)  [unwired: 2 in, 2 out]
        n647 = Subtract(x=w1098, y=w1099) -> (x-y=w1102:dbl)
        n648 = property on="Y Velocity SP mm/sec" class="DigNum (strict)"() -> ("Value"=w1092:dbl)  [unwired: 2 in, 2 out]
        n649 = property on="Y mm/rev" class="DigNum (strict)"() -> ("Value"=w1085:dbl)  [unwired: 2 in, 2 out]
        n650 = Divide(x=w1102, y=w1085) -> (x/y=w1103:dbl)
        n651 = Divide(x=w1092, y=w1085) -> (x/y=w1093:dbl)
        n652 = To Double Precision Float(number=w1101) -> (double precision float=w1086:dbl)
        n653 = Multiply(x=w1103, y=w1086) -> (x*y=w1097:dbl)
        n654 = Multiply(x=w1093, y=w1086) -> (x*y=w1090:dbl)
        n655 = property on="Y Step SP" class="DigNum (strict)"() -> ("Maximum"=w1095:dbl)  [unwired: 2 in, 2 out]
        n656 = property on="Y Step SP" class="DigNum (strict)"() -> ("Minimum"=w1094:dbl)  [unwired: 2 in, 2 out]
        n657 = In Range and Coerce(upper limit=w1088, x=w1090, lower limit=w1087) -> (coerced(x)=w1089:dbl)  [unwired: 1 out]
        n658 = To Long Integer(number=w1089) -> (32bit integer=w1091:i32)
        n659 = In Range and Coerce(upper limit=w1095, x=w1097, lower limit=w1094) -> (coerced(x)=w1096:dbl)  [unwired: 1 out]
        n660 = To Long Integer(number=w1096) -> (32bit integer=w1100:i32)
        n661 = property on="Y Velocity SP step/sec" class="DigNum (strict)"("Val(Sgnl)"=w1091) -> ()  [unwired: 2 in, 2 out]
        n662 = property on="Y Step SP" class="DigNum (strict)"("Val(Sgnl)"=w1100) -> ()  [unwired: 2 in, 2 out]
      }
      event #5 {
        n663 = event-data() -> ()  [unwired: 1 in, 7 out]
        n664 = property on="X steps/rev" class="DigNum (strict)"() -> ("Value"=w1120:u32)  [unwired: 2 in, 2 out]
        n665 = property on="X offset mm" class="DigNum (strict)"() -> ("Value"=w1118:dbl)  [unwired: 2 in, 2 out]
        n666 = property on="X Position SP mm" class="DigNum (strict)"() -> ("Value"=w1117:dbl)  [unwired: 2 in, 2 out]
        n667 = property on="X Velocity SP step/sec" class="DigNum (strict)"() -> ("Maximum"=w1107:dbl)  [unwired: 2 in, 2 out]
        n668 = property on="X Velocity SP step/sec" class="DigNum (strict)"() -> ("Minimum"=w1106:dbl)  [unwired: 2 in, 2 out]
        n669 = Subtract(x=w1117, y=w1118) -> (x-y=w1121:dbl)
        n670 = property on="X Velocity SP mm/sec" class="DigNum (strict)"() -> ("Value"=w1111:dbl)  [unwired: 2 in, 2 out]
        n671 = property on="X mm/rev" class="DigNum (strict)"() -> ("Value"=w1104:dbl)  [unwired: 2 in, 2 out]
        n672 = Divide(x=w1121, y=w1104) -> (x/y=w1122:dbl)
        n673 = Divide(x=w1111, y=w1104) -> (x/y=w1112:dbl)
        n674 = To Double Precision Float(number=w1120) -> (double precision float=w1105:dbl)
        n675 = Multiply(x=w1122, y=w1105) -> (x*y=w1116:dbl)
        n676 = Multiply(x=w1112, y=w1105) -> (x*y=w1109:dbl)
        n677 = property on="X Step SP" class="DigNum (strict)"() -> ("Maximum"=w1114:dbl)  [unwired: 2 in, 2 out]
        n678 = property on="X Step SP" class="DigNum (strict)"() -> ("Minimum"=w1113:dbl)  [unwired: 2 in, 2 out]
        n679 = In Range and Coerce(upper limit=w1107, x=w1109, lower limit=w1106) -> (coerced(x)=w1108:dbl)  [unwired: 1 out]
        n680 = To Long Integer(number=w1108) -> (32bit integer=w1110:i32)
        n681 = In Range and Coerce(upper limit=w1114, x=w1116, lower limit=w1113) -> (coerced(x)=w1115:dbl)  [unwired: 1 out]
        n682 = To Long Integer(number=w1115) -> (32bit integer=w1119:i32)
        n683 = property on="X Velocity SP step/sec" class="DigNum (strict)"("Val(Sgnl)"=w1110) -> ()  [unwired: 2 in, 2 out]
        n684 = property on="X Step SP" class="DigNum (strict)"("Val(Sgnl)"=w1119) -> ()  [unwired: 2 in, 2 out]
      }
      event #6 {
        n685 = event-data() -> ()  [unwired: 1 in, 7 out]
        n686 = property on="Z steps/rev" class="DigNum (strict)"() -> ("Value"=w1137:u32)  [unwired: 2 in, 2 out]
        n687 = property on="Z offset mm" class="DigNum (strict)"() -> ("Value"=w1135:dbl)  [unwired: 2 in, 2 out]
        n688 = property on="Z Position SP mm" class="DigNum (strict)"() -> ("Value"=w1134:dbl)  [unwired: 2 in, 2 out]
        n689 = property on="Z Velocity SP step/sec" class="DigNum (strict)"() -> ("Maximum"=w1124:dbl)  [unwired: 2 in, 2 out]
        n690 = property on="Z Velocity SP step/sec" class="DigNum (strict)"() -> ("Minimum"=w1123:dbl)  [unwired: 2 in, 2 out]
        n691 = Subtract(x=w1134, y=w1135) -> (x-y=w1138:dbl)
        n692 = property on="Z Velocity SP mm/sec" class="DigNum (strict)"() -> ("Value"=w1128:dbl)  [unwired: 2 in, 2 out]
        n693 = property on="Z mm/rev" class="DigNum (strict)"() -> ("Value"=w1140:dbl)  [unwired: 2 in, 2 out]
        n694 = Divide(x=w1138, y=w1140) -> (x/y=w1139:dbl)
        n695 = Divide(x=w1128, y=w1140) -> (x/y=w1129:dbl)
        n696 = To Double Precision Float(number=w1137) -> (double precision float=w1141:dbl)
        n697 = Multiply(x=w1139, y=w1141) -> (x*y=w1133:dbl)
        n698 = Multiply(x=w1129, y=w1141) -> (x*y=w1126:dbl)
        n699 = property on="Z Step SP" class="DigNum (strict)"() -> ("Maximum"=w1131:dbl)  [unwired: 2 in, 2 out]
        n700 = property on="Z Step SP" class="DigNum (strict)"() -> ("Minimum"=w1130:dbl)  [unwired: 2 in, 2 out]
        n701 = In Range and Coerce(upper limit=w1124, x=w1126, lower limit=w1123) -> (coerced(x)=w1125:dbl)  [unwired: 1 out]
        n702 = To Long Integer(number=w1125) -> (32bit integer=w1127:i32)
        n703 = In Range and Coerce(upper limit=w1131, x=w1133, lower limit=w1130) -> (coerced(x)=w1132:dbl)  [unwired: 1 out]
        n704 = To Long Integer(number=w1132) -> (32bit integer=w1136:i32)
        n705 = property on="Z Velocity SP step/sec" class="DigNum (strict)"("Val(Sgnl)"=w1127) -> ()  [unwired: 2 in, 2 out]
        n706 = property on="Z Step SP" class="DigNum (strict)"("Val(Sgnl)"=w1136) -> ()  [unwired: 2 in, 2 out]
      }
      event #7 {
        n707 = event-data() -> ()  [unwired: 1 in, 7 out]
        n708 = property on="R steps/rev" class="DigNum (strict)"() -> ("Value"=w1159:u32)  [unwired: 2 in, 2 out]
        n709 = property on="R offset deg" class="DigNum (strict)"() -> ("Value"=w1157:dbl)  [unwired: 2 in, 2 out]
        n710 = property on="R Position SP deg" class="DigNum (strict)"() -> ("Value"=w1156:dbl)  [unwired: 2 in, 2 out]
        n711 = property on="R Velocity SP step/sec" class="DigNum (strict)"() -> ("Maximum"=w1146:dbl)  [unwired: 2 in, 2 out]
        n712 = property on="R Velocity SP step/sec" class="DigNum (strict)"() -> ("Minimum"=w1145:dbl)  [unwired: 2 in, 2 out]
        n713 = Subtract(x=w1156, y=w1157) -> (x-y=w1160:dbl)
        n714 = property on="R Velocity SP deg/sec" class="DigNum (strict)"() -> ("Value"=w1150:dbl)  [unwired: 2 in, 2 out]
        n715 = property on="R deg/rev" class="DigNum (strict)"() -> ("Value"=w1143:dbl)  [unwired: 2 in, 2 out]
        n716 = Divide(x=w1160, y=w1143) -> (x/y=w1161:dbl)
        n717 = Divide(x=w1150, y=w1143) -> (x/y=w1151:dbl)
        n718 = To Double Precision Float(number=w1159) -> (double precision float=w1144:dbl)
        n719 = Multiply(x=w1161, y=w1144) -> (x*y=w1155:dbl)
        n720 = Multiply(x=w1151, y=w1144) -> (x*y=w1148:dbl)
        n721 = property on="R Step SP" class="DigNum (strict)"() -> ("Maximum"=w1153:dbl)  [unwired: 2 in, 2 out]
        n722 = property on="R Step SP" class="DigNum (strict)"() -> ("Minimum"=w1152:dbl)  [unwired: 2 in, 2 out]
        n723 = Absolute Value(x=w1148) -> (abs(x)=w1142:dbl)
        n724 = In Range and Coerce(upper limit=w1153, x=w1155, lower limit=w1152) -> (coerced(x)=w1154:dbl)  [unwired: 1 out]
        n725 = In Range and Coerce(upper limit=w1146, x=w1142, lower limit=w1145) -> (coerced(x)=w1147:dbl)  [unwired: 1 out]
        n726 = To Long Integer(number=w1154) -> (32bit integer=w1158:i32)
        n727 = To Long Integer(number=w1147) -> (32bit integer=w1149:i32)
        n728 = property on="R Step SP" class="DigNum (strict)"("Val(Sgnl)"=w1158) -> ()  [unwired: 2 in, 2 out]
        n729 = property on="R Velocity SP step/sec" class="DigNum (strict)"("Val(Sgnl)"=w1149) -> ()  [unwired: 2 in, 2 out]
      }
      event #8 {
        n730 = event-data() -> ()  [unwired: 1 in, 7 out]
        n731 = property on="Y steps/rev" class="DigNum (strict)"() -> ("Value"=w1177:u32)  [unwired: 2 in, 2 out]
        n732 = To Double Precision Float(number=w1177) -> (double precision float=w1163:dbl)
        n733 = property on="Y mm/rev" class="DigNum (strict)"() -> ("Value"=w1162:dbl)  [unwired: 2 in, 2 out]
        n734 = property on="Y Scan Length SP mm" class="DigNum (strict)"() -> ("Value"=w1175:dbl)  [unwired: 2 in, 2 out]
        n735 = property on="Y Scan Velocity SP mm/sec" class="DigNum (strict)"() -> ("Value"=w1169:dbl)  [unwired: 2 in, 2 out]
        n736 = property on="Y Scan Velocity SP steps/sec" class="DigNum (strict)"() -> ("Maximum"=w1165:dbl)  [unwired: 2 in, 2 out]
        n737 = property on="Y Scan Velocity SP steps/sec" class="DigNum (strict)"() -> ("Minimum"=w1164:dbl)  [unwired: 2 in, 2 out]
        n738 = Divide(x=w1175, y=w1162) -> (x/y=w1178:dbl)
        n739 = Divide(x=w1169, y=w1162) -> (x/y=w1170:dbl)
        n740 = Multiply(x=w1178, y=w1163) -> (x*y=w1174:dbl)
        n741 = Multiply(x=w1170, y=w1163) -> (x*y=w1167:dbl)
        n742 = property on="Y Step SP" class="DigNum (strict)"() -> ("Maximum"=w1171:dbl)  [unwired: 2 in, 2 out]
        n743 = property on="Y Step SP" class="DigNum (strict)"() -> ("Minimum"=w1172:dbl)  [unwired: 2 in, 2 out]
        n744 = In Range and Coerce(upper limit=w1165, x=w1167, lower limit=w1164) -> (coerced(x)=w1166:dbl)  [unwired: 1 out]
        n745 = To Long Integer(number=w1166) -> (32bit integer=w1168:i32)
        n746 = In Range and Coerce(upper limit=w1171, x=w1174, lower limit=w1172) -> (coerced(x)=w1173:dbl)  [unwired: 1 out]
        n747 = To Long Integer(number=w1173) -> (32bit integer=w1176:i32)
        n748 = property on="Y Scan Velocity SP steps/sec" class="DigNum (strict)"("Val(Sgnl)"=w1168) -> ()  [unwired: 2 in, 2 out]
        n749 = property on="Y Scan Length SP steps" class="DigNum (strict)"("Val(Sgnl)"=w1176) -> ()  [unwired: 2 in, 2 out]
      }
      event #9 {
        n750 = event-data() -> ()  [unwired: 1 in, 7 out]
        n751 = property on="X steps/rev" class="DigNum (strict)"() -> ("Value"=w1194:u32)  [unwired: 2 in, 2 out]
        n752 = To Double Precision Float(number=w1194) -> (double precision float=w1180:dbl)
        n753 = property on="X mm/rev" class="DigNum (strict)"() -> ("Value"=w1179:dbl)  [unwired: 2 in, 2 out]
        n754 = property on="X Scan Length SP mm" class="DigNum (strict)"() -> ("Value"=w1192:dbl)  [unwired: 2 in, 2 out]
        n755 = property on="X Scan Velocity SP mm/sec" class="DigNum (strict)"() -> ("Value"=w1186:dbl)  [unwired: 2 in, 2 out]
        n756 = property on="X Scan Velocity SP steps/sec" class="DigNum (strict)"() -> ("Maximum"=w1182:dbl)  [unwired: 2 in, 2 out]
        n757 = property on="X Scan Velocity SP steps/sec" class="DigNum (strict)"() -> ("Minimum"=w1181:dbl)  [unwired: 2 in, 2 out]
        n758 = Divide(x=w1192, y=w1179) -> (x/y=w1195:dbl)
        n759 = Divide(x=w1186, y=w1179) -> (x/y=w1187:dbl)
        n760 = Multiply(x=w1195, y=w1180) -> (x*y=w1191:dbl)
        n761 = Multiply(x=w1187, y=w1180) -> (x*y=w1184:dbl)
        n762 = property on="X Step SP" class="DigNum (strict)"() -> ("Maximum"=w1188:dbl)  [unwired: 2 in, 2 out]
        n763 = property on="X Step SP" class="DigNum (strict)"() -> ("Minimum"=w1189:dbl)  [unwired: 2 in, 2 out]
        n764 = In Range and Coerce(upper limit=w1182, x=w1184, lower limit=w1181) -> (coerced(x)=w1183:dbl)  [unwired: 1 out]
        n765 = To Long Integer(number=w1183) -> (32bit integer=w1185:i32)
        n766 = In Range and Coerce(upper limit=w1188, x=w1191, lower limit=w1189) -> (coerced(x)=w1190:dbl)  [unwired: 1 out]
        n767 = To Long Integer(number=w1190) -> (32bit integer=w1193:i32)
        n768 = property on="X Scan Velocity SP steps/sec" class="DigNum (strict)"("Val(Sgnl)"=w1185) -> ()  [unwired: 2 in, 2 out]
        n769 = property on="X Scan Length SP steps" class="DigNum (strict)"("Val(Sgnl)"=w1193) -> ()  [unwired: 2 in, 2 out]
      }
      event #10 {
        n770 = event-data() -> ()  [unwired: 1 in, 7 out]
        n771 = property on="Z steps/rev" class="DigNum (strict)"() -> ("Value"=w1211:u32)  [unwired: 2 in, 2 out]
        n772 = To Double Precision Float(number=w1211) -> (double precision float=w1197:dbl)
        n773 = property on="Z mm/rev" class="DigNum (strict)"() -> ("Value"=w1196:dbl)  [unwired: 2 in, 2 out]
        n774 = property on="Z Scan Length SP mm" class="DigNum (strict)"() -> ("Value"=w1209:dbl)  [unwired: 2 in, 2 out]
        n775 = property on="Z Scan Velocity SP mm/sec" class="DigNum (strict)"() -> ("Value"=w1203:dbl)  [unwired: 2 in, 2 out]
        n776 = property on="Z Scan Velocity SP steps/sec" class="DigNum (strict)"() -> ("Maximum"=w1199:dbl)  [unwired: 2 in, 2 out]
        n777 = property on="Z Scan Velocity SP steps/sec" class="DigNum (strict)"() -> ("Minimum"=w1198:dbl)  [unwired: 2 in, 2 out]
        n778 = Divide(x=w1209, y=w1196) -> (x/y=w1212:dbl)
        n779 = Divide(x=w1203, y=w1196) -> (x/y=w1204:dbl)
        n780 = Multiply(x=w1212, y=w1197) -> (x*y=w1208:dbl)
        n781 = Multiply(x=w1204, y=w1197) -> (x*y=w1201:dbl)
        n782 = property on="Z Step SP" class="DigNum (strict)"() -> ("Maximum"=w1205:dbl)  [unwired: 2 in, 2 out]
        n783 = property on="Z Step SP" class="DigNum (strict)"() -> ("Minimum"=w1206:dbl)  [unwired: 2 in, 2 out]
        n784 = In Range and Coerce(upper limit=w1199, x=w1201, lower limit=w1198) -> (coerced(x)=w1200:dbl)  [unwired: 1 out]
        n785 = To Long Integer(number=w1200) -> (32bit integer=w1202:i32)
        n786 = In Range and Coerce(upper limit=w1205, x=w1208, lower limit=w1206) -> (coerced(x)=w1207:dbl)  [unwired: 1 out]
        n787 = To Long Integer(number=w1207) -> (32bit integer=w1210:i32)
        n788 = property on="Z Scan Velocity SP steps/sec" class="DigNum (strict)"("Val(Sgnl)"=w1202) -> ()  [unwired: 2 in, 2 out]
        n789 = property on="Z Scan Length SP steps" class="DigNum (strict)"("Val(Sgnl)"=w1210) -> ()  [unwired: 2 in, 2 out]
      }
      event #11 {
        n790 = event-data() -> ()  [unwired: 1 in, 7 out]
        n791 = property on="R steps/rev" class="DigNum (strict)"() -> ("Value"=w1229:u32)  [unwired: 2 in, 2 out]
        n792 = To Double Precision Float(number=w1229) -> (double precision float=w1215:dbl)
        n793 = property on="R Velocity SP step/sec" class="DigNum (strict)"() -> ("Maximum"=w1217:dbl)  [unwired: 2 in, 2 out]
        n794 = property on="R Scan Length SP deg" class="DigNum (strict)"() -> ("Value"=w1227:dbl)  [unwired: 2 in, 2 out]
        n795 = property on="R deg/rev" class="DigNum (strict)"() -> ("Value"=w1214:dbl)  [unwired: 2 in, 2 out]
        n796 = property on="R Scan Velocity SP steps/sec" class="DigNum (strict)"() -> ("Minimum"=w1216:dbl)  [unwired: 2 in, 2 out]
        n797 = property on="R Scan Velocity SP deg/sec" class="DigNum (strict)"() -> ("Value"=w1221:dbl)  [unwired: 2 in, 2 out]
        n798 = Divide(x=w1227, y=w1214) -> (x/y=w1230:dbl)
        n799 = Multiply(x=w1230, y=w1215) -> (x*y=w1226:dbl)
        n800 = Divide(x=w1221, y=w1214) -> (x/y=w1222:dbl)
        n801 = property on="R Step SP" class="DigNum (strict)"() -> ("Maximum"=w1223:dbl)  [unwired: 2 in, 2 out]
        n802 = property on="R Step SP" class="DigNum (strict)"() -> ("Minimum"=w1224:dbl)  [unwired: 2 in, 2 out]
        n803 = Multiply(x=w1222, y=w1215) -> (x*y=w1219:dbl)
        n804 = Absolute Value(x=w1219) -> (abs(x)=w1213:dbl)
        n805 = In Range and Coerce(upper limit=w1223, x=w1226, lower limit=w1224) -> (coerced(x)=w1225:dbl)  [unwired: 1 out]
        n806 = To Long Integer(number=w1225) -> (32bit integer=w1228:i32)
        n807 = In Range and Coerce(upper limit=w1217, x=w1213, lower limit=w1216) -> (coerced(x)=w1218:dbl)  [unwired: 1 out]
        n808 = To Long Integer(number=w1218) -> (32bit integer=w1220:i32)
        n809 = property on="R Scan Length SP steps" class="DigNum (strict)"("Val(Sgnl)"=w1228) -> ()  [unwired: 2 in, 2 out]
        n810 = property on="R Scan Velocity SP steps/sec" class="DigNum (strict)"("Val(Sgnl)"=w1220) -> ()  [unwired: 2 in, 2 out]
      }
      event #12 {
        n811 = event-data() -> ()  [unwired: 1 in, 7 out]
        n812 = flat-sequence {
          tunnel: w1237 -> [w1247]
          tunnel: w1238 -> [w1248]
          tunnel: [w1248] -> w1234
          tunnel: [w1247] -> w1233
          tunnel: [w1251] -> w1236
          tunnel: [w1250] -> w1235
          tunnel: w1234 -> [w1253]
          tunnel: w1233 -> [w1252]
          tunnel: [w1274] -> w1240
          tunnel: [w1269] -> w1239
          tunnel: w1236 -> [w1273]
          tunnel: w1235 -> [w1272]
          tunnel: [w1268] -> w1232
          tunnel: [w1285] -> w1242
          tunnel: [w1280] -> w1241
          tunnel: w1240 -> [w1283]
          tunnel: w1239 -> [w1284]
          tunnel: w1232 -> [w1281]
          tunnel: [w1281] -> w1231
          tunnel: [w1288] -> w1243
          tunnel: [w1291] -> w1244
          tunnel: w1242 -> [w1290]
          tunnel: w1241 -> [w1289]
          tunnel: w1231 -> [w1292]
          frame #0 {
            n813 = property on="Scan Go" class="Bool"("DisabledEnum"=T2."Disabled and Grayed Out" ("Disabled")) -> ()  [unwired: 2 in, 2 out]
            n814 = property on="Y Go" class="Bool"("DisabledEnum"=T2."Disabled and Grayed Out" ("Disabled")) -> ()  [unwired: 2 in, 2 out]
          }
          frame #1 {
            n815 = property on="Y Step SP" class="DigNum (strict)"() -> ("Value"=w1261:i32)  [unwired: 2 in, 2 out]
            n816 = property on="Y Step PV" class="DigNum (strict)"() -> ("Value"=w1260:i32)  [unwired: 2 in, 2 out]
            n817 = property on="Y Backlash" class="DigNum (strict)"() -> ("Value"=w1249:i32)  [unwired: 2 in, 2 out]
            n818 = Subtract(x=w1261, y=w1260) -> (x-y=w1259:i32)
            n819 = Sign(1:w1249) -> (0:w1257:i32)
            n820 = Sign(1:w1259) -> (0:w1258:i32)
            n821 = Multiply(x=w1258, y=w1257) -> (x*y=w1256:i32)
            n822 = Equal?(x=w1256, y=1) -> (x = y?=w1254:bool)
            n823 = case shown="False" w1254 {
              tunnel: w1253 -> [w1264 w1266]
              tunnel: w1252 -> [w1263 w1265]
              tunnel: [w1263 w1265] -> w1251
              tunnel: [w1264 w1266] -> w1250
              frame #0 {
                n824 = property on="Y Backlash corr" class="Bool (strict)"("Val(Sgnl)"=FALSE ("Value (Signaling)")) -> ()  [unwired: 2 in, 2 out]
              }
              frame #1 {
                n825 = property on="Y Backlash corr" class="Bool (strict)"("Val(Sgnl)"=TRUE ("Value (Signaling)")) -> ()  [unwired: 2 in, 2 out]
              }
            }
          }
          frame #2 {
            w1268 = 0.1 ("Delay Time (s)")
            # "Velocity Setting"
            n826 = property on="Y Velocity SP step/sec" class="DigNum (strict)"() -> ("Value"=w1277:i32)  [unwired: 2 in, 2 out]
            n827 = Number To Decimal String(number=w1277) -> ()  [unwired: 1 in, 1 out]
            n828 = property on="Y steps/rev" class="DigNum (strict)"() -> ("Value"=w1276:u32)  [unwired: 2 in, 2 out]
            n829 = Divide(x=w1277, y=w1276) -> (x/y=w1278:dbl)
            n830 = Number To Fractional String(number=w1278) -> (F-format string=w1271:string)  [unwired: 3 in]
            n831 = call "Applied Send Command.vi"("error in (no error)"=w1273, "Extra"=w1271, "Command"=T1."Velocity Setting", "VISA resource name"=w1272) -> ("error out"=w1270:errorcluster, "VISA resource name out"=w1274:refnum<visa-resource-name>)  [unwired: 3 in, 1 out]
            n832 = call "Time Delay22"("error in (no error)"=w1270, "Delay Time (s)"=w1268) -> ("error out"=w1269:errorcluster)  [unwired: 9 in]
          }
          frame #3 {
            # "Move to Abs Position"
            n833 = property on="Y Step SP" class="DigNum (strict)"() -> ("Value"=w1287:i32)  [unwired: 2 in, 2 out]
            n834 = Number To Decimal String(number=w1287) -> (decimal integer string=w1282:string)  [unwired: 1 in]
            n835 = call "Applied Send Command.vi"("error in (no error)"=w1284, "Extra"=w1282, "Command"=T1."Distance or Position", "VISA resource name"=w1283) -> ("error out"=w1279:errorcluster, "VISA resource name out"=w1285:refnum<visa-resource-name>)  [unwired: 3 in, 1 out]
            n836 = call "Time Delay"("error in (no error)"=w1279, "Delay Time (s)"=w1281) -> ("error out"=w1280:errorcluster)  [unwired: 9 in]
          }
          frame #4 {
            n837 = call "Applied Send Command.vi"("error in (no error)"=w1289, "Command"=T1."Feed to Position", "VISA resource name"=w1290) -> ("error out"=w1293:errorcluster, "VISA resource name out"=w1291:refnum<visa-resource-name>)  [unwired: 4 in, 1 out]
            n838 = call "Time Delay23"("error in (no error)"=w1293, "Delay Time (s)"=w1292) -> ("error out"=w1288:errorcluster)  [unwired: 9 in]
          }
        }
      }
      event #13 {
        n839 = event-data() -> ()  [unwired: 1 in, 7 out]
        n840 = flat-sequence {
          tunnel: w1299 -> [w1311]
          tunnel: w1300 -> [w1312]
          tunnel: [w1312] -> w1302
          tunnel: [w1311] -> w1301
          tunnel: [w1315] -> w1304
          tunnel: [w1314] -> w1303
          tunnel: w1302 -> [w1317]
          tunnel: w1301 -> [w1316]
          tunnel: [w1335] -> w1306
          tunnel: [w1333] -> w1305
          tunnel: w1304 -> [w1336]
          tunnel: w1303 -> [w1337]
          tunnel: [w1332] -> w1296
          tunnel: [w1346] -> w1308
          tunnel: [w1345] -> w1307
          tunnel: w1306 -> [w1347]
          tunnel: w1305 -> [w1349]
          tunnel: w1296 -> [w1343]
          tunnel: [w1343] -> w1295
          tunnel: [w1358] -> w1298
          tunnel: [w1354] -> w1297
          tunnel: w1308 -> [w1355]
          tunnel: w1307 -> [w1352]
          tunnel: w1295 -> [w1357]
          frame #0 {
            n841 = property on="Scan Go" class="Bool"("DisabledEnum"=T2."Disabled and Grayed Out" ("Disabled")) -> ()  [unwired: 2 in, 2 out]
            n842 = property on="Z Go" class="Bool"("DisabledEnum"=T2."Disabled and Grayed Out" ("Disabled")) -> ()  [unwired: 2 in, 2 out]
          }
          frame #1 {
            n843 = property on="Z Step SP" class="DigNum (strict)"() -> ("Value"=w1325:i32)  [unwired: 2 in, 2 out]
            n844 = property on="Z Step PV" class="DigNum (strict)"() -> ("Value"=w1324:i32)  [unwired: 2 in, 2 out]
            n845 = property on="Z Backlash" class="DigNum (strict)"() -> ("Value"=w1313:i32)  [unwired: 2 in, 2 out]
            n846 = Subtract(x=w1325, y=w1324) -> (x-y=w1323:i32)
            n847 = Sign(1:w1313) -> (0:w1321:i32)
            n848 = Sign(1:w1323) -> (0:w1322:i32)
            n849 = Multiply(x=w1322, y=w1321) -> (x*y=w1320:i32)
            n850 = Equal?(x=w1320, y=1) -> (x = y?=w1318:bool)
            n851 = case shown="True" w1318 {
              tunnel: w1317 -> [w1328 w1330]
              tunnel: w1316 -> [w1327 w1329]
              tunnel: [w1327 w1329] -> w1315
              tunnel: [w1328 w1330] -> w1314
              frame #0 {
                n852 = property on="Z Backlash corr" class="Bool (strict)"("Val(Sgnl)"=FALSE ("Value (Signaling)")) -> ()  [unwired: 2 in, 2 out]
              }
              frame #1 {
                n853 = property on="Z Backlash corr" class="Bool (strict)"("Val(Sgnl)"=TRUE ("Value (Signaling)")) -> ()  [unwired: 2 in, 2 out]
              }
            }
          }
          frame #2 {
            w1332 = 0.1 ("Delay Time (s)")
            n854 = property on="Z Velocity SP step/sec" class="DigNum (strict)"() -> ("Value"=w1339:i32)  [unwired: 2 in, 2 out]
            n855 = property on="Z steps/rev" class="DigNum (strict)"() -> ("Value"=w1338:u32)  [unwired: 2 in, 2 out]
            n856 = Divide(x=w1339, y=w1338) -> (x/y=w1340:dbl)
            n857 = Number To Fractional String(number=w1340) -> (F-format string=w1341:string)  [unwired: 3 in]
            n858 = call "Applied Send Command.vi"("error in (no error)"=w1336, "Extra"=w1341, "Command"=T1."Velocity Setting", "VISA resource name"=w1337) -> ("error out"=w1334:errorcluster, "VISA resource name out"=w1335:refnum<visa-resource-name>)  [unwired: 3 in, 1 out]
            n859 = call "Time Delay52"("error in (no error)"=w1334, "Delay Time (s)"=w1332) -> ("error out"=w1333:errorcluster)  [unwired: 9 in]
          }
          frame #3 {
            # "Move to Abs Position"
            n860 = property on="Z Step SP" class="DigNum (strict)"() -> ("Value"=w1351:i32)  [unwired: 2 in, 2 out]
            n861 = Number To Decimal String(number=w1351) -> (decimal integer string=w1348:string)  [unwired: 1 in]
            n862 = call "Applied Send Command.vi"("error in (no error)"=w1349, "Extra"=w1348, "Command"=T1."Distance or Position", "VISA resource name"=w1347) -> ("error out"=w1344:errorcluster, "VISA resource name out"=w1346:refnum<visa-resource-name>)  [unwired: 3 in, 1 out]
            n863 = call "Time Delay51"("error in (no error)"=w1344, "Delay Time (s)"=w1343) -> ("error out"=w1345:errorcluster)  [unwired: 9 in]
          }
          frame #4 {
            n864 = call "Applied Send Command.vi"("error in (no error)"=w1352, "Command"=T1."Feed to Position", "VISA resource name"=w1355) -> ("error out"=w1353:errorcluster, "VISA resource name out"=w1354:refnum<visa-resource-name>)  [unwired: 4 in, 1 out]
            n865 = call "Time Delay28"("error in (no error)"=w1353, "Delay Time (s)"=w1357) -> ("error out"=w1358:errorcluster)  [unwired: 9 in]
          }
        }
      }
      event #14 {
        n866 = event-data() -> ()  [unwired: 1 in, 7 out]
        n867 = flat-sequence {
          tunnel: w1363 -> [w1375]
          tunnel: w1364 -> [w1376]
          tunnel: [w1376] -> w1366
          tunnel: [w1375] -> w1365
          tunnel: [w1379] -> w1368
          tunnel: [w1378] -> w1367
          tunnel: w1366 -> [w1381]
          tunnel: w1365 -> [w1380]
          tunnel: [w1397] -> w1370
          tunnel: [w1398] -> w1369
          tunnel: w1368 -> [w1399]
          tunnel: w1367 -> [w1400]
          tunnel: [w1396] -> w1360
          tunnel: [w1410] -> w1372
          tunnel: [w1408] -> w1371
          tunnel: w1370 -> [w1409]
          tunnel: w1369 -> [w1411]
          tunnel: w1360 -> [w1406]
          tunnel: [w1406] -> w1359
          tunnel: [w1421] -> w1362
          tunnel: [w1417] -> w1361
          tunnel: w1372 -> [w1418]
          tunnel: w1371 -> [w1415]
          tunnel: w1359 -> [w1420]
          frame #0 {
            n868 = property on="Scan Go" class="Bool"("DisabledEnum"=T2."Disabled and Grayed Out" ("Disabled")) -> ()  [unwired: 2 in, 2 out]
            n869 = property on="R Go" class="Bool"("DisabledEnum"=T2."Disabled and Grayed Out" ("Disabled")) -> ()  [unwired: 2 in, 2 out]
          }
          frame #1 {
            n870 = property on="R Step SP" class="DigNum (strict)"() -> ("Value"=w1389:i32)  [unwired: 2 in, 2 out]
            n871 = property on="R Step PV" class="DigNum (strict)"() -> ("Value"=w1388:i32)  [unwired: 2 in, 2 out]
            n872 = property on="R Backlash" class="DigNum (strict)"() -> ("Value"=w1377:i32)  [unwired: 2 in, 2 out]
            n873 = Subtract(x=w1389, y=w1388) -> (x-y=w1387:i32)
            n874 = Sign(1:w1377) -> (0:w1385:i32)
            n875 = Sign(1:w1387) -> (0:w1386:i32)
            n876 = Multiply(x=w1386, y=w1385) -> (x*y=w1384:i32)
            n877 = Equal?(x=w1384, y=1) -> (x = y?=w1382:bool)
            n878 = case shown="True" w1382 {
              tunnel: w1381 -> [w1392 w1394]
              tunnel: w1380 -> [w1391 w1393]
              tunnel: [w1391 w1393] -> w1379
              tunnel: [w1392 w1394] -> w1378
              frame #0 {
                n879 = property on="R Backlash corr" class="Bool (strict)"("Val(Sgnl)"=FALSE ("Value (Signaling)")) -> ()  [unwired: 2 in, 2 out]
              }
              frame #1 {
                n880 = property on="R Backlash corr" class="Bool (strict)"("Val(Sgnl)"=TRUE ("Value (Signaling)")) -> ()  [unwired: 2 in, 2 out]
              }
            }
          }
          frame #2 {
            w1396 = 0.1 ("Delay Time (s)")
            # "Velocity Setting"
            n881 = property on="R Velocity SP step/sec" class="DigNum (strict)"() -> ("Value"=w1402:i32)  [unwired: 2 in, 2 out]
            n882 = property on="R steps/rev" class="DigNum (strict)"() -> ("Value"=w1401:u32)  [unwired: 2 in, 2 out]
            n883 = Divide(x=w1402, y=w1401) -> (x/y=w1403:dbl)
            n884 = Number To Fractional String(number=w1403) -> (F-format string=w1404:string)  [unwired: 3 in]
            n885 = call "Applied Send Command.vi"("error in (no error)"=w1399, "Extra"=w1404, "VISA resource name"=w1400) -> ("error out"=w1405:errorcluster, "VISA resource name out"=w1397:refnum<visa-resource-name>)  [unwired: 4 in, 1 out]
            n886 = call "Time Delay54"("error in (no error)"=w1405, "Delay Time (s)"=w1396) -> ("error out"=w1398:errorcluster)  [unwired: 9 in]
          }
          frame #3 {
            # "Distance/Position"
            n887 = property on="R Step SP" class="DigNum (strict)"() -> ("Value"=w1412:i32)  [unwired: 2 in, 2 out]
            n888 = Number To Decimal String(number=w1412) -> (decimal integer string=w1413:string)  [unwired: 1 in]
            n889 = call "Applied Send Command.vi"("error in (no error)"=w1411, "Extra"=w1413, "Command"=T1."Distance or Position", "VISA resource name"=w1409) -> ("error out"=w1407:errorcluster, "VISA resource name out"=w1410:refnum<visa-resource-name>)  [unwired: 3 in, 1 out]
            n890 = call "Time Delay53"("error in (no error)"=w1407, "Delay Time (s)"=w1406) -> ("error out"=w1408:errorcluster)  [unwired: 9 in]
          }
          frame #4 {
            # "Feed to Position"
            n891 = call "Applied Send Command.vi"("error in (no error)"=w1415, "Command"=T1."Feed to Position", "VISA resource name"=w1418) -> ("error out"=w1416:errorcluster, "VISA resource name out"=w1417:refnum<visa-resource-name>)  [unwired: 4 in, 1 out]
            n892 = call "Time Delay29"("error in (no error)"=w1416, "Delay Time (s)"=w1420) -> ("error out"=w1421:errorcluster)  [unwired: 9 in]
          }
        }
      }
      event #15 {
        n893 = event-data() -> ()  [unwired: 1 in, 7 out]
        n894 = flat-sequence {
          tunnel: [w1437] -> w1433
          tunnel: [w1436] -> w1432
          tunnel: w1431 -> [w1437]
          tunnel: w1430 -> [w1436]
          tunnel: [w1442] -> w1435
          tunnel: [w1441] -> w1434
          tunnel: w1433 -> [w1444]
          tunnel: w1432 -> [w1443]
          tunnel: [w1463] -> w1427
          tunnel: [w1460] -> w1425
          tunnel: w1435 -> [w1464]
          tunnel: w1434 -> [w1465]
          tunnel: [w1459] -> w1423
          tunnel: w1427 -> [w1472]
          tunnel: [w1471] -> w1426
          tunnel: w1425 -> [w1473]
          tunnel: [w1474] -> w1424
          tunnel: w1423 -> [w1470]
          tunnel: [w1470] -> w1422
          tunnel: w1426 -> [w1484]
          tunnel: w1424 -> [w1483]
          tunnel: [w1482] -> w1429
          tunnel: [w1481] -> w1428
          tunnel: w1422 -> [w1479]
          frame #0 {
            n895 = property on="Scan Go" class="Bool"("DisabledEnum"=T2."Disabled and Grayed Out" ("Disabled")) -> ()  [unwired: 2 in, 2 out]
            n896 = property on="X Go" class="Bool"("DisabledEnum"=T2."Disabled and Grayed Out" ("Disabled")) -> ()  [unwired: 2 in, 2 out]
          }
          frame #1 {
            n897 = property on="X Step SP" class="DigNum (strict)"() -> ("Value"=w1452:i32)  [unwired: 2 in, 2 out]
            n898 = property on="X Step PV" class="DigNum (strict)"() -> ("Value"=w1451:i32)  [unwired: 2 in, 2 out]
            n899 = property on="X Backlash" class="DigNum (strict)"() -> ("Value"=w1440:i32)  [unwired: 2 in, 2 out]
            n900 = Subtract(x=w1452, y=w1451) -> (x-y=w1450:i32)
            n901 = Sign(1:w1440) -> (0:w1448:i32)
            n902 = Sign(1:w1450) -> (0:w1449:i32)
            n903 = Multiply(x=w1449, y=w1448) -> (x*y=w1447:i32)
            n904 = Equal?(x=w1447, y=1) -> (x = y?=w1445:bool)
            n905 = case shown="True" w1445 {
              tunnel: w1444 -> [w1455 w1457]
              tunnel: w1443 -> [w1454 w1456]
              tunnel: [w1454 w1456] -> w1442
              tunnel: [w1455 w1457] -> w1441
              frame #0 {
                n906 = property on="X Backlash corr" class="Bool (strict)"("Val(Sgnl)"=FALSE ("Value (Signaling)")) -> ()  [unwired: 2 in, 2 out]
              }
              frame #1 {
                n907 = property on="X Backlash corr" class="Bool (strict)"("Val(Sgnl)"=TRUE ("Value (Signaling)")) -> ()  [unwired: 2 in, 2 out]
              }
            }
          }
          frame #2 {
            w1459 = 0.1 ("Delay Time (s)")
            n908 = property on="X Velocity SP step/sec" class="DigNum (strict)"() -> ("Value"=w1462:i32)  [unwired: 2 in, 2 out]
            n909 = property on="X steps/rev" class="DigNum (strict)"() -> ("Value"=w1466:u32)  [unwired: 2 in, 2 out]
            n910 = Divide(x=w1462, y=w1466) -> (x/y=w1467:dbl)
            n911 = Number To Fractional String(number=w1467) -> (F-format string=w1468:string)  [unwired: 3 in]
            n912 = call "Applied Send Command.vi"("error in (no error)"=w1464, "Extra"=w1468, "Command"=T1."Velocity Setting", "VISA resource name"=w1465) -> ("error out"=w1461:errorcluster, "VISA resource name out"=w1463:refnum<visa-resource-name>)  [unwired: 3 in, 1 out]
            n913 = call "Time Delay14"("error in (no error)"=w1461, "Delay Time (s)"=w1459) -> ("error out"=w1460:errorcluster)  [unwired: 9 in]
          }
          frame #3 {
            # "Distance/Position"
            n914 = property on="X Step SP" class="DigNum (strict)"() -> ("Value"=w1475:i32)  [unwired: 2 in, 2 out]
            n915 = Number To Decimal String(number=w1475) -> (decimal integer string=w1477:string)  [unwired: 1 in]
            n916 = call "Applied Send Command.vi"("error in (no error)"=w1473, "Extra"=w1477, "Command"=T1."Distance or Position", "VISA resource name"=w1472) -> ("error out"=w1476:errorcluster, "VISA resource name out"=w1471:refnum<visa-resource-name>)  [unwired: 3 in, 1 out]
            n917 = call "Time Delay31"("error in (no error)"=w1476, "Delay Time (s)"=w1470) -> ("error out"=w1474:errorcluster)  [unwired: 9 in]
          }
          frame #4 {
            # "Feed to Position"
            n918 = call "Applied Send Command.vi"("error in (no error)"=w1483, "Command"=T1."Feed to Position", "VISA resource name"=w1484) -> ("error out"=w1480:errorcluster, "VISA resource name out"=w1482:refnum<visa-resource-name>)  [unwired: 4 in, 1 out]
            n919 = call "Time Delay15"("error in (no error)"=w1480, "Delay Time (s)"=w1479) -> ("error out"=w1481:errorcluster)  [unwired: 9 in]
          }
        }
      }
      event #16 {
        n920 = event-data() -> ()  [unwired: 1 in, 7 out]
        n921 = flat-sequence {
          tunnel: [w1501] -> w1493
          tunnel: [w1512] -> w1492
          tunnel: w1491 -> [w1509]
          tunnel: w1490 -> [w1508]
          tunnel: w1493 -> [w1519]
          tunnel: w1492 -> [w1518]
          tunnel: [w1519] -> w1487
          tunnel: [w1518] -> w1486
          tunnel: [w1521] -> w1488
          tunnel: [w1522] -> w1489
          tunnel: w1487 -> [w1522]
          tunnel: w1486 -> [w1521]
          frame #0 {
            # "VELOCITY"
            n922 = property on="X steps/rev" class="DigNum (strict)"() -> ("Value"=w1494:u32)  [unwired: 2 in, 2 out]
            n923 = property on="X Scan Velocity SP steps/sec" class="DigNum (strict)"() -> ("Value"=w1495:i32)  [unwired: 2 in, 2 out]
            n924 = Divide(x=w1495, y=w1494) -> (x/y=w1496:dbl)
            n925 = Number To Fractional String(number=w1496) -> (F-format string=w1510:string)  [unwired: 3 in]
            n926 = call "Applied Send Command.vi"("error in (no error)"=w1508, "Extra"=w1510, "Command"=T1."Velocity Setting", "VISA resource name"=w1509) -> ("error out"=w1497:errorcluster, "VISA resource name out"=w1498:refnum<visa-resource-name>)  [unwired: 3 in, 1 out]
            n927 = call "Time Delay9"("error in (no error)"=w1497) -> ("error out"=w1499:errorcluster)  [unwired: 10 in]
            n928 = call "Applied Send Command.vi"("error in (no error)"=w1499, "Extra"="", "Command"=T1."Velocity Setting", "VISA resource name"=w1498) -> ("error out"=w1500:errorcluster, "read buffer"=w1505:string, "VISA resource name out"=w1501:refnum<visa-resource-name>)  [unwired: 3 in]
            n929 = call "Time Delay10"("error in (no error)"=w1500) -> ("error out"=w1512:errorcluster)  [unwired: 10 in]
            n930 = Fract/Exp String To Number(string=w1505, offset=3) -> (number=w1503:dbl)  [unwired: 2 in, 1 out]
            n931 = Multiply(x=w1503, y=w1494) -> (x*y=w1502:dbl)
            n932 = property on="X velocity PV step/sec" class="DigNum (strict)"("Val(Sgnl)"=w1502) -> ()  [unwired: 2 in, 2 out]
          }
          frame #1 {
            n933 = property on="X Scan" class="Bool (strict)"("Val(Sgnl)"=TRUE ("Slew Ready 2")) -> ()  [unwired: 2 in, 2 out]
            n934 = property on="Scan Cancel" class="Bool"("DisabledEnum"=T2."Enabled" ("Disabled")) -> ()  [unwired: 2 in, 2 out]
            n935 = property on="Scan Go" class="Bool"("DisabledEnum"=T2."Enabled" ("Disabled")) -> ()  [unwired: 2 in, 2 out]
            n936 = property on="X Scan Length SP steps" class="DigNum (strict)"("DisabledEnum"=T2."Disabled and Grayed Out" ("Disabled")) -> ()  [unwired: 2 in, 2 out]
            n937 = property on="X Scan Velocity SP steps/sec" class="DigNum (strict)"("DisabledEnum"=T2."Disabled and Grayed Out" ("Disabled")) -> ()  [unwired: 2 in, 2 out]
          }
          frame #2 {
            n938 = property on="X Go" class="Bool"("DisabledEnum"=T2."Disabled and Grayed Out" ("Disabled")) -> ()  [unwired: 2 in, 2 out]
          }
        }
      }
      event #17 {
        n939 = event-data() -> ()  [unwired: 1 in, 7 out]
        n940 = flat-sequence {
          tunnel: w1530 -> [w1542]
          tunnel: w1529 -> [w1543]
          tunnel: [w1533] -> w1527
          tunnel: [w1549] -> w1526
          tunnel: w1527 -> [w1556]
          tunnel: w1526 -> [w1555]
          tunnel: [w1556] -> w1524
          tunnel: [w1555] -> w1523
          tunnel: [w1558] -> w1528
          tunnel: [w1559] -> w1525
          tunnel: w1524 -> [w1559]
          tunnel: w1523 -> [w1558]
          frame #0 {
            # "VELOCITY"
            n941 = property on="Y Scan Velocity SP steps/sec" class="DigNum (strict)"() -> ("Value"=w1545:i32)  [unwired: 2 in, 2 out]
            n942 = property on="Y steps/rev" class="DigNum (strict)"() -> ("Value"=w1536:u32)  [unwired: 2 in, 2 out]
            n943 = Divide(x=w1545, y=w1536) -> (x/y=w1546:dbl)
            n944 = Number To Fractional String(number=w1546) -> (F-format string=w1547:string)  [unwired: 3 in]
            n945 = call "Applied Send Command.vi"("error in (no error)"=w1542, "Extra"=w1547, "Command"=T1."Velocity Setting", "VISA resource name"=w1543) -> ("error out"=w1544:errorcluster, "VISA resource name out"=w1534:refnum<visa-resource-name>)  [unwired: 3 in, 1 out]
            n946 = call "Time Delay5"("error in (no error)"=w1544) -> ("error out"=w1535:errorcluster)  [unwired: 10 in]
            n947 = call "Applied Send Command.vi"("error in (no error)"=w1535, "Extra"="", "Command"=T1."Velocity Setting", "VISA resource name"=w1534) -> ("error out"=w1532:errorcluster, "read buffer"=w1539:string, "VISA resource name out"=w1533:refnum<visa-resource-name>)  [unwired: 3 in]
            n948 = Fract/Exp String To Number(string=w1539, offset=3) -> (number=w1538:dbl)  [unwired: 2 in, 1 out]
            n949 = call "Time Delay6"("error in (no error)"=w1532) -> ("error out"=w1549:errorcluster)  [unwired: 10 in]
            n950 = Multiply(x=w1538, y=w1536) -> (x*y=w1537:dbl)
            n951 = property on="Y velocity PV step/sec" class="DigNum (strict)"("Val(Sgnl)"=w1537) -> ()  [unwired: 2 in, 2 out]
          }
          frame #1 {
            n952 = property on="Y Scan" class="Bool (strict)"("Val(Sgnl)"=TRUE ("Slew Ready 2")) -> ()  [unwired: 2 in, 2 out]
            n953 = property on="Scan Cancel" class="Bool"("DisabledEnum"=T2."Enabled" ("Disabled")) -> ()  [unwired: 2 in, 2 out]
            n954 = property on="Scan Go" class="Bool"("DisabledEnum"=T2."Enabled" ("Disabled")) -> ()  [unwired: 2 in, 2 out]
            n955 = property on="Y Scan Length SP steps" class="DigNum (strict)"("DisabledEnum"=T2."Disabled and Grayed Out" ("Disabled")) -> ()  [unwired: 2 in, 2 out]
            n956 = property on="Y Scan Velocity SP steps/sec" class="DigNum (strict)"("DisabledEnum"=T2."Disabled and Grayed Out" ("Disabled")) -> ()  [unwired: 2 in, 2 out]
          }
          frame #2 {
            n957 = property on="Y Go" class="Bool"("DisabledEnum"=T2."Disabled and Grayed Out" ("Disabled")) -> ()  [unwired: 2 in, 2 out]
          }
        }
      }
      event #18 {
        n958 = event-data() -> ()  [unwired: 1 in, 7 out]
        n959 = flat-sequence {
          tunnel: [w1572] -> w1567
          tunnel: [w1586] -> w1566
          tunnel: w1563 -> [w1568]
          tunnel: w1562 -> [w1569]
          tunnel: w1567 -> [w1593]
          tunnel: w1566 -> [w1592]
          tunnel: [w1593] -> w1565
          tunnel: [w1592] -> w1564
          tunnel: [w1595] -> w1561
          tunnel: [w1596] -> w1560
          tunnel: w1565 -> [w1596]
          tunnel: w1564 -> [w1595]
          frame #0 {
            # "VELOCITY"
            n960 = property on="Z Scan Velocity SP steps/sec" class="DigNum (strict)"() -> ("Value"=w1582:i32)  [unwired: 2 in, 2 out]
            n961 = property on="Z steps/rev" class="DigNum (strict)"() -> ("Value"=w1575:u32)  [unwired: 2 in, 2 out]
            n962 = Divide(x=w1582, y=w1575) -> (x/y=w1583:dbl)
            n963 = Number To Fractional String(number=w1583) -> (F-format string=w1584:string)  [unwired: 3 in]
            n964 = call "Applied Send Command.vi"("error in (no error)"=w1569, "Extra"=w1584, "Command"=T1."Velocity Setting", "VISA resource name"=w1568) -> ("error out"=w1581:errorcluster, "VISA resource name out"=w1571:refnum<visa-resource-name>)  [unwired: 3 in, 1 out]
            n965 = call "Time Delay24"("error in (no error)"=w1581) -> ("error out"=w1570:errorcluster)  [unwired: 10 in]
            n966 = call "Applied Send Command.vi"("error in (no error)"=w1570, "Extra"="", "Command"=T1."Velocity Setting", "VISA resource name"=w1571) -> ("error out"=w1573:errorcluster, "read buffer"=w1578:string, "VISA resource name out"=w1572:refnum<visa-resource-name>)  [unwired: 3 in]
            n967 = call "Time Delay25"("error in (no error)"=w1573) -> ("error out"=w1586:errorcluster)  [unwired: 10 in]
            n968 = Fract/Exp String To Number(string=w1578, offset=3) -> (number=w1577:dbl)  [unwired: 2 in, 1 out]
            n969 = Multiply(x=w1577, y=w1575) -> (x*y=w1574:dbl)
            n970 = property on="Z  velocity PV step/sec" class="DigNum (strict)"("Val(Sgnl)"=w1574) -> ()  [unwired: 2 in, 2 out]
          }
          frame #1 {
            n971 = property on="Z Scan" class="Bool (strict)"("Val(Sgnl)"=TRUE ("Slew Ready 2")) -> ()  [unwired: 2 in, 2 out]
            n972 = property on="Scan Cancel" class="Bool"("DisabledEnum"=T2."Enabled" ("Disabled")) -> ()  [unwired: 2 in, 2 out]
            n973 = property on="Scan Go" class="Bool"("DisabledEnum"=T2."Enabled" ("Disabled")) -> ()  [unwired: 2 in, 2 out]
            n974 = property on="Z Scan Length SP steps" class="DigNum (strict)"("DisabledEnum"=T2."Disabled and Grayed Out" ("Disabled")) -> ()  [unwired: 2 in, 2 out]
            n975 = property on="Z Scan Velocity SP steps/sec" class="DigNum (strict)"("DisabledEnum"=T2."Disabled and Grayed Out" ("Disabled")) -> ()  [unwired: 2 in, 2 out]
          }
          frame #2 {
            n976 = property on="Z Go" class="Bool"("DisabledEnum"=T2."Disabled and Grayed Out" ("Disabled")) -> ()  [unwired: 2 in, 2 out]
          }
        }
      }
      event #19 {
        n977 = event-data() -> ()  [unwired: 1 in, 7 out]
        n978 = flat-sequence {
          tunnel: [w1608] -> w1604
          tunnel: [w1623] -> w1603
          tunnel: w1600 -> [w1616]
          tunnel: w1599 -> [w1617]
          tunnel: w1604 -> [w1630]
          tunnel: w1603 -> [w1629]
          tunnel: [w1630] -> w1602
          tunnel: [w1629] -> w1601
          tunnel: [w1632] -> w1597
          tunnel: [w1633] -> w1598
          tunnel: w1602 -> [w1633]
          tunnel: w1601 -> [w1632]
          frame #0 {
            # "VELOCITY"
            n979 = property on="R Scan Velocity SP steps/sec" class="DigNum (strict)"() -> ("Value"=w1618:i32)  [unwired: 2 in, 2 out]
            n980 = property on="R steps/rev" class="DigNum (strict)"() -> ("Value"=w1606:u32)  [unwired: 2 in, 2 out]
            n981 = Divide(x=w1618, y=w1606) -> (x/y=w1620:dbl)
            n982 = Number To Fractional String(number=w1620) -> (F-format string=w1621:string)  [unwired: 3 in]
            n983 = call "Applied Send Command.vi"("error in (no error)"=w1617, "Extra"=w1621, "Command"=T1."Velocity Setting", "VISA resource name"=w1616) -> ("error out"=w1619:errorcluster, "VISA resource name out"=w1610:refnum<visa-resource-name>)  [unwired: 3 in, 1 out]
            n984 = call "Time Delay26"("error in (no error)"=w1619) -> ("error out"=w1609:errorcluster)  [unwired: 10 in]
            n985 = call "Applied Send Command.vi"("error in (no error)"=w1609, "Extra"="", "Command"=T1."Velocity Setting", "VISA resource name"=w1610) -> ("error out"=w1607:errorcluster, "read buffer"=w1613:string, "VISA resource name out"=w1608:refnum<visa-resource-name>)  [unwired: 3 in]
            n986 = call "Time Delay27"("error in (no error)"=w1607) -> ("error out"=w1623:errorcluster)  [unwired: 10 in]
            n987 = Fract/Exp String To Number(string=w1613, offset=3) -> (number=w1612:dbl)  [unwired: 2 in, 1 out]
            n988 = Multiply(x=w1612, y=w1606) -> (x*y=w1605:dbl)
            n989 = property on="R velocity PV step/sec" class="DigNum (strict)"("Val(Sgnl)"=w1605) -> ()  [unwired: 2 in, 2 out]
          }
          frame #1 {
            n990 = property on="R Scan" class="Bool (strict)"("Val(Sgnl)"=TRUE ("Slew Ready 2")) -> ()  [unwired: 2 in, 2 out]
            n991 = property on="Scan Cancel" class="Bool"("DisabledEnum"=T2."Enabled" ("Disabled")) -> ()  [unwired: 2 in, 2 out]
            n992 = property on="Scan Go" class="Bool"("DisabledEnum"=T2."Enabled" ("Disabled")) -> ()  [unwired: 2 in, 2 out]
            n993 = property on="R Scan Length SP steps" class="DigNum (strict)"("DisabledEnum"=T2."Disabled and Grayed Out" ("Disabled")) -> ()  [unwired: 2 in, 2 out]
            n994 = property on="R Scan Velocity SP steps/sec" class="DigNum (strict)"("DisabledEnum"=T2."Disabled and Grayed Out" ("Disabled")) -> ()  [unwired: 2 in, 2 out]
          }
          frame #2 {
            n995 = property on="R Go" class="Bool"("DisabledEnum"=T2."Disabled and Grayed Out" ("Disabled")) -> ()  [unwired: 2 in, 2 out]
          }
        }
      }
      event #20 {
        n996 = event-data() -> ()  [unwired: 1 in, 4 out]
        n997 = event-data() -> ()  [unwired: 3 in, 1 out]
      }
      event #21 {
        n998 = event-data() -> ()  [unwired: 1 in, 7 out]
        n999 = flat-sequence {
          tunnel: [w1664] -> w1647
          tunnel: [w1663] -> w1646
          tunnel: w1645 -> [w1665]
          tunnel: w1644 -> [w1662]
          frame #0 {
            n1000 = call "Applied Send Command.vi"("error in (no error)"=w1662, "Command"=T1."Stop", "VISA resource name"=w1665) -> ("error out"=w1663:errorcluster, "VISA resource name out"=w1664:refnum<visa-resource-name>)  [unwired: 4 in, 1 out]
          }
        }
        n1001 = flat-sequence {
          tunnel: w1651 -> [w1668]
          tunnel: w1650 -> [w1667]
          tunnel: [w1669] -> w1649
          tunnel: [w1670] -> w1648
          frame #0 {
            n1002 = call "Applied Send Command.vi"("error in (no error)"=w1667, "Command"=T1."Stop", "VISA resource name"=w1668) -> ("error out"=w1670:errorcluster, "VISA resource name out"=w1669:refnum<visa-resource-name>)  [unwired: 4 in, 1 out]
          }
        }
        n1003 = flat-sequence {
          tunnel: [w1659] -> w1641
          tunnel: [w1660] -> w1640
          tunnel: w1643 -> [w1657]
          tunnel: w1642 -> [w1658]
          frame #0 {
            n1004 = call "Applied Send Command.vi"("error in (no error)"=w1658, "Command"=T1."Stop", "VISA resource name"=w1657) -> ("error out"=w1660:errorcluster, "VISA resource name out"=w1659:refnum<visa-resource-name>)  [unwired: 4 in, 1 out]
          }
        }
        n1005 = flat-sequence {
          tunnel: w1639 -> [w1652]
          tunnel: w1638 -> [w1653]
          tunnel: [w1655] -> w1637
          tunnel: [w1654] -> w1636
          frame #0 {
            n1006 = call "Applied Send Command.vi"("error in (no error)"=w1653, "Command"=T1."Stop", "VISA resource name"=w1652) -> ("error out"=w1654:errorcluster, "VISA resource name out"=w1655:refnum<visa-resource-name>)  [unwired: 4 in, 1 out]
          }
        }
      }
      event #22 {
        n1007 = event-data() -> ()  [unwired: 1 in, 7 out]
        n1008 = flat-sequence {
          tunnel: w1687 -> [w1725]
          tunnel: w1686 -> [w1724]
          tunnel: [w1727] -> w1689
          tunnel: [w1726] -> w1688
          tunnel: [w1735] -> w1684
          tunnel: [w1736] -> w1685
          tunnel: w1689 -> [w1736]
          tunnel: w1688 -> [w1735]
          frame #0 {
            n1009 = call "Applied Send Command.vi"("error in (no error)"=w1724, "Command"=T1."Stop", "VISA resource name"=w1725) -> ("error out"=w1726:errorcluster, "VISA resource name out"=w1727:refnum<visa-resource-name>)  [unwired: 4 in, 1 out]
          }
          frame #1 {
            n1010 = property on="X Scan" class="Bool (strict)"("Value"=FALSE ("Slew Ready")) -> ()  [unwired: 2 in, 2 out]
            n1011 = property on="X Scan set" class="Bool"("DisabledEnum"=T2."Enabled" ("Disabled")) -> ()  [unwired: 2 in, 2 out]
            n1012 = property on="X Scan Velocity SP steps/sec" class="DigNum (strict)"("DisabledEnum"=T2."Enabled" ("Disabled")) -> ()  [unwired: 2 in, 2 out]
            n1013 = property on="X Scan Length SP steps" class="DigNum (strict)"("DisabledEnum"=T2."Enabled" ("Disabled")) -> ()  [unwired: 2 in, 2 out]
            n1014 = property on="X Go" class="Bool"("DisabledEnum"=T2."Enabled" ("Disabled")) -> ()  [unwired: 2 in, 2 out]
            n1015 = property on="X Scan OK" class="Bool"("DisabledEnum"=T2."Enabled" ("Disabled")) -> ()  [unwired: 2 in, 2 out]
          }
        }
        n1016 = flat-sequence {
          tunnel: w1695 -> [w1738]
          tunnel: w1694 -> [w1737]
          tunnel: [w1740] -> w1691
          tunnel: [w1739] -> w1690
          tunnel: [w1748] -> w1696
          tunnel: [w1749] -> w1697
          tunnel: w1691 -> [w1749]
          tunnel: w1690 -> [w1748]
          frame #0 {
            n1017 = call "Applied Send Command.vi"("error in (no error)"=w1737, "Command"=T1."Stop", "VISA resource name"=w1738) -> ("error out"=w1739:errorcluster, "VISA resource name out"=w1740:refnum<visa-resource-name>)  [unwired: 4 in, 1 out]
          }
          frame #1 {
            n1018 = property on="Y Scan" class="Bool (strict)"("Value"=FALSE ("Slew Ready")) -> ()  [unwired: 2 in, 2 out]
            n1019 = property on="Y Go" class="Bool"("DisabledEnum"=T2."Enabled" ("Disabled")) -> ()  [unwired: 2 in, 2 out]
            n1020 = property on="Y Scan Velocity SP steps/sec" class="DigNum (strict)"("DisabledEnum"=T2."Enabled" ("Disabled")) -> ()  [unwired: 2 in, 2 out]
            n1021 = property on="Y Scan set" class="Bool"("DisabledEnum"=T2."Enabled" ("Disabled")) -> ()  [unwired: 2 in, 2 out]
            n1022 = property on="Y Scan OK" class="Bool"("DisabledEnum"=T2."Enabled" ("Disabled")) -> ()  [unwired: 2 in, 2 out]
            n1023 = property on="Y Scan Length SP steps" class="DigNum (strict)"("DisabledEnum"=T2."Enabled" ("Disabled")) -> ()  [unwired: 2 in, 2 out]
          }
        }
        n1024 = flat-sequence {
          tunnel: [w1714] -> w1683
          tunnel: [w1713] -> w1682
          tunnel: w1681 -> [w1712]
          tunnel: w1680 -> [w1711]
          tunnel: [w1722] -> w1678
          tunnel: [w1723] -> w1679
          tunnel: w1683 -> [w1723]
          tunnel: w1682 -> [w1722]
          frame #0 {
            n1025 = call "Applied Send Command.vi"("error in (no error)"=w1711, "Command"=T1."Stop", "VISA resource name"=w1712) -> ("error out"=w1713:errorcluster, "VISA resource name out"=w1714:refnum<visa-resource-name>)  [unwired: 4 in, 1 out]
          }
          frame #1 {
            n1026 = property on="Z Scan" class="Bool (strict)"("Value"=FALSE ("Slew Ready")) -> ()  [unwired: 2 in, 2 out]
            n1027 = property on="Z Scan set" class="Bool"("DisabledEnum"=T2."Enabled" ("Disabled")) -> ()  [unwired: 2 in, 2 out]
            n1028 = property on="Z Scan Velocity SP steps/sec" class="DigNum (strict)"("DisabledEnum"=T2."Enabled" ("Disabled")) -> ()  [unwired: 2 in, 2 out]
            n1029 = property on="Z Scan Length SP steps" class="DigNum (strict)"("DisabledEnum"=T2."Enabled" ("Disabled")) -> ()  [unwired: 2 in, 2 out]
            n1030 = property on="Z Go" class="Bool"("DisabledEnum"=T2."Enabled" ("Disabled")) -> ()  [unwired: 2 in, 2 out]
            n1031 = property on="Z Scan OK" class="Bool"("DisabledEnum"=T2."Enabled" ("Disabled")) -> ()  [unwired: 2 in, 2 out]
          }
        }
        n1032 = flat-sequence {
          tunnel: [w1701] -> w1677
          tunnel: [w1700] -> w1676
          tunnel: w1675 -> [w1698]
          tunnel: w1674 -> [w1699]
          tunnel: [w1709] -> w1672
          tunnel: [w1710] -> w1673
          tunnel: w1677 -> [w1710]
          tunnel: w1676 -> [w1709]
          frame #0 {
            n1033 = call "Applied Send Command.vi"("error in (no error)"=w1699, "Command"=T1."Stop", "VISA resource name"=w1698) -> ("error out"=w1700:errorcluster, "VISA resource name out"=w1701:refnum<visa-resource-name>)  [unwired: 4 in, 1 out]
          }
          frame #1 {
            n1034 = property on="R Scan" class="Bool (strict)"("Value"=FALSE ("Slew Ready")) -> ()  [unwired: 2 in, 2 out]
            n1035 = property on="R Scan Velocity SP steps/sec" class="DigNum (strict)"("DisabledEnum"=T2."Enabled" ("Disabled")) -> ()  [unwired: 2 in, 2 out]
            n1036 = property on="R Go" class="Bool"("DisabledEnum"=T2."Enabled" ("Disabled")) -> ()  [unwired: 2 in, 2 out]
            n1037 = property on="R Scan OK" class="Bool"("DisabledEnum"=T2."Enabled" ("Disabled")) -> ()  [unwired: 2 in, 2 out]
            n1038 = property on="R Scan Length SP steps" class="DigNum (strict)"("DisabledEnum"=T2."Enabled" ("Disabled")) -> ()  [unwired: 2 in, 2 out]
            n1039 = property on="R Scan set" class="Bool"("DisabledEnum"=T2."Enabled" ("Disabled")) -> ()  [unwired: 2 in, 2 out]
          }
        }
        n1040 = property on="Scan Go" class="Bool"("DisabledEnum"=T2."Disabled and Grayed Out" ("Disabled")) -> ()  [unwired: 2 in, 2 out]
        n1041 = property on="Scan Cancel" class="Bool"("DisabledEnum"=T2."Disabled and Grayed Out" ("Disabled")) -> ()  [unwired: 2 in, 2 out]
      }
      event #23 {
        n1042 = event-data() -> ()  [unwired: 1 in, 7 out]
        n1043 = flat-sequence {
          tunnel: w1785 -> [w1804]
          tunnel: w1784 -> [w1805]
          tunnel: w1783 -> [w1802]
          tunnel: w1782 -> [w1803]
          tunnel: w1781 -> [w1801]
          tunnel: w1780 -> [w1800]
          tunnel: w1779 -> [w1799]
          tunnel: w1778 -> [w1798]
          tunnel: [w1797] -> w1769
          tunnel: [w1796] -> w1767
          tunnel: [w1795] -> w1765
          tunnel: [w1794] -> w1763
          tunnel: [w1793] -> w1761
          tunnel: [w1792] -> w1759
          tunnel: [w1791] -> w1757
          tunnel: [w1790] -> w1755
          tunnel: [w1789] -> w1753
          tunnel: [w1788] -> w1752
          tunnel: [w1787] -> w1751
          tunnel: [w1786] -> w1750
          tunnel: w1769 -> [w1861]
          tunnel: [w1860] -> w1768
          tunnel: w1767 -> [w1859]
          tunnel: [w1858] -> w1766
          tunnel: w1765 -> [w1857]
          tunnel: [w1856] -> w1764
          tunnel: w1763 -> [w1855]
          tunnel: [w1854] -> w1762
          tunnel: w1761 -> [w1853]
          tunnel: [w1852] -> w1760
          tunnel: w1759 -> [w1850]
          tunnel: [w1851] -> w1758
          tunnel: w1757 -> [w1849]
          tunnel: [w1848] -> w1756
          tunnel: w1755 -> [w1847]
          tunnel: [w1846] -> w1754
          tunnel: w1753 -> [w1845]
          tunnel: w1752 -> [w1844]
          tunnel: w1751 -> [w1843]
          tunnel: w1750 -> [w1842]
          tunnel: [w1896] -> w1777
          tunnel: [w1895] -> w1776
          tunnel: [w1894] -> w1775
          tunnel: [w1893] -> w1774
          tunnel: [w1892] -> w1773
          tunnel: [w1891] -> w1772
          tunnel: [w1898] -> w1771
          tunnel: [w1897] -> w1770
          tunnel: w1768 -> [w1898]
          tunnel: w1766 -> [w1897]
          tunnel: w1764 -> [w1896]
          tunnel: w1762 -> [w1895]
          tunnel: w1760 -> [w1894]
          tunnel: w1758 -> [w1893]
          tunnel: w1756 -> [w1892]
          tunnel: w1754 -> [w1891]
          frame #0 {
            n1044 = property on="X Scan" class="Bool (strict)"() -> ("Value"=w1786:bool)  [unwired: 2 in, 2 out]
            n1045 = property on="Y Scan" class="Bool (strict)"() -> ("Value"=w1787:bool)  [unwired: 2 in, 2 out]
            n1046 = property on="Z Scan" class="Bool (strict)"() -> ("Value"=w1788:bool)  [unwired: 2 in, 2 out]
            n1047 = property on="R Scan" class="Bool (strict)"() -> ("Value"=w1789:bool)  [unwired: 2 in, 2 out]
            n1048 = case shown="True" w1786 {
              tunnel: w1805 -> [w1825 w1829]
              tunnel: [w1825 w1828] -> w1796
              tunnel: w1804 -> [w1824 w1827]
              tunnel: [w1824 w1826] -> w1797
              frame #0 {
              }
              frame #1 {
                n1049 = property on="X Scan Length SP steps" class="DigNum (strict)"() -> ("Value"=w1830:i32)  [unwired: 2 in, 2 out]
                n1050 = Number To Decimal String(number=w1830) -> (decimal integer string=w1831:string)  [unwired: 1 in]
                n1051 = call "Applied Send Command.vi"("error in (no error)"=w1829, "Extra"=w1831, "Command"=T1."Distance or Position", "VISA resource name"=w1827) -> ("error out"=w1828:errorcluster, "VISA resource name out"=w1826:refnum<visa-resource-name>)  [unwired: 3 in, 1 out]
              }
            }
            n1052 = case shown="True" w1787 {
              tunnel: w1802 -> [w1834 w1839]
              tunnel: w1803 -> [w1833 w1838]
              tunnel: [w1833 w1835] -> w1794
              tunnel: [w1834 w1836] -> w1795
              frame #0 {
              }
              frame #1 {
                n1053 = property on="Y Scan Length SP steps" class="DigNum (strict)"() -> ("Value"=w1837:i32)  [unwired: 2 in, 2 out]
                n1054 = Number To Decimal String(number=w1837) -> (decimal integer string=w1840:string)  [unwired: 1 in]
                n1055 = call "Applied Send Command.vi"("error in (no error)"=w1838, "Extra"=w1840, "Command"=T1."Distance or Position", "VISA resource name"=w1839) -> ("error out"=w1835:errorcluster, "VISA resource name out"=w1836:refnum<visa-resource-name>)  [unwired: 3 in, 1 out]
              }
            }
            n1056 = case shown="True" w1788 {
              tunnel: w1801 -> [w1816 w1820]
              tunnel: [w1816 w1819] -> w1793
              tunnel: [w1815 w1818] -> w1792
              tunnel: w1800 -> [w1815 w1817]
              frame #0 {
              }
              frame #1 {
                n1057 = property on="Z Scan Length SP steps" class="DigNum (strict)"() -> ("Value"=w1821:i32)  [unwired: 2 in, 2 out]
                n1058 = Number To Decimal String(number=w1821) -> (decimal integer string=w1822:string)  [unwired: 1 in]
                n1059 = call "Applied Send Command.vi"("error in (no error)"=w1817, "Extra"=w1822, "Command"=T1."Distance or Position", "VISA resource name"=w1820) -> ("error out"=w1818:errorcluster, "VISA resource name out"=w1819:refnum<visa-resource-name>)  [unwired: 3 in, 1 out]
              }
            }
            n1060 = case shown="True" w1789 {
              tunnel: w1799 -> [w1807 w1812]
              tunnel: [w1807 w1811] -> w1791
              tunnel: w1798 -> [w1806 w1810]
              tunnel: [w1806 w1809] -> w1790
              frame #0 {
              }
              frame #1 {
                n1061 = property on="R Scan Length SP steps" class="DigNum (strict)"() -> ("Value"=w1808:i32)  [unwired: 2 in, 2 out]
                n1062 = Number To Decimal String(number=w1808) -> (decimal integer string=w1813:string)  [unwired: 1 in]
                n1063 = call "Applied Send Command.vi"("error in (no error)"=w1810, "Extra"=w1813, "Command"=T1."Distance or Position", "VISA resource name"=w1812) -> ("error out"=w1809:errorcluster, "VISA resource name out"=w1811:refnum<visa-resource-name>)  [unwired: 3 in, 1 out]
              }
            }
          }
          frame #1 {
            n1064 = case shown="True" w1842 {
              tunnel: w1861 -> [w1884 w1888]
              tunnel: [w1884 w1887] -> w1860
              tunnel: w1859 -> [w1883 w1886]
              tunnel: [w1883 w1885] -> w1858
              frame #0 {
              }
              frame #1 {
                n1065 = call "Applied Send Command.vi"("error in (no error)"=w1886, "Command"=T1."Feed to Length", "VISA resource name"=w1888) -> ("error out"=w1885:errorcluster, "VISA resource name out"=w1887:refnum<visa-resource-name>)  [unwired: 4 in, 1 out]
              }
            }
            n1066 = case shown="True" w1843 {
              tunnel: w1857 -> [w1877 w1881]
              tunnel: [w1877 w1880] -> w1856
              tunnel: w1855 -> [w1876 w1879]
              tunnel: [w1876 w1878] -> w1854
              frame #0 {
              }
              frame #1 {
                n1067 = call "Applied Send Command.vi"("error in (no error)"=w1879, "Command"=T1."Feed to Length", "VISA resource name"=w1881) -> ("error out"=w1878:errorcluster, "VISA resource name out"=w1880:refnum<visa-resource-name>)  [unwired: 4 in, 1 out]
              }
            }
            n1068 = case shown="False" w1844 {
              tunnel: w1853 -> [w1870 w1874]
              tunnel: [w1870 w1873] -> w1852
              tunnel: [w1869 w1872] -> w1851
              tunnel: w1850 -> [w1869 w1871]
              frame #0 {
              }
              frame #1 {
                n1069 = call "Applied Send Command.vi"("error in (no error)"=w1871, "Command"=T1."Feed to Length", "VISA resource name"=w1874) -> ("error out"=w1872:errorcluster, "VISA resource name out"=w1873:refnum<visa-resource-name>)  [unwired: 4 in, 1 out]
              }
            }
            n1070 = case shown="False" w1845 {
              tunnel: w1849 -> [w1863 w1867]
              tunnel: [w1863 w1866] -> w1848
              tunnel: w1847 -> [w1862 w1865]
              tunnel: [w1862 w1864] -> w1846
              frame #0 {
              }
              frame #1 {
                n1071 = call "Applied Send Command.vi"("error in (no error)"=w1865, "Command"=T1."Feed to Length", "VISA resource name"=w1867) -> ("error out"=w1864:errorcluster, "VISA resource name out"=w1866:refnum<visa-resource-name>)  [unwired: 4 in, 1 out]
              }
            }
          }
          frame #2 {
            n1072 = call "Time Delay7"("Delay Time (s)"=0.1) -> ()  [unwired: 10 in, 1 out]
            n1073 = property on="R Scan" class="Bool (strict)"("Val(Sgnl)"=FALSE ("Slew Ready 2")) -> ()  [unwired: 2 in, 2 out]
            n1074 = property on="Z Scan" class="Bool (strict)"("Val(Sgnl)"=FALSE ("Slew Ready 2")) -> ()  [unwired: 2 in, 2 out]
            n1075 = property on="X Scan" class="Bool (strict)"("Val(Sgnl)"=FALSE ("Slew Ready 2")) -> ()  [unwired: 2 in, 2 out]
            n1076 = property on="Y Scan" class="Bool (strict)"("Val(Sgnl)"=FALSE ("Slew Ready 2")) -> ()  [unwired: 2 in, 2 out]
            n1077 = property on="Z Scan Velocity SP steps/sec" class="DigNum (strict)"("DisabledEnum"=T2."Enabled" ("Disabled")) -> ()  [unwired: 2 in, 2 out]
            n1078 = property on="X Scan Length SP steps" class="DigNum (strict)"("DisabledEnum"=T2."Enabled" ("Disabled")) -> ()  [unwired: 2 in, 2 out]
            n1079 = property on="Y Scan Selocity SP steps/sec" class="DigNum (strict)"("DisabledEnum"=T2."Enabled" ("Disabled")) -> ()  [unwired: 2 in, 2 out]
            n1080 = property on="Z Scan Length SP steps" class="DigNum (strict)"("DisabledEnum"=T2."Enabled" ("Disabled")) -> ()  [unwired: 2 in, 2 out]
            n1081 = property on="Y Scan Length SP steps" class="DigNum (strict)"("DisabledEnum"=T2."Enabled" ("Disabled")) -> ()  [unwired: 2 in, 2 out]
            n1082 = property on="X Scan Velocity SP steps/sec" class="DigNum (strict)"("DisabledEnum"=T2."Enabled" ("Disabled")) -> ()  [unwired: 2 in, 2 out]
            n1083 = property on="R Scan Velocity SP steps/sec" class="DigNum (strict)"("DisabledEnum"=T2."Enabled" ("Disabled")) -> ()  [unwired: 2 in, 2 out]
            n1084 = property on="R Scan Length SP steps" class="DigNum (strict)"("DisabledEnum"=T2."Enabled" ("Disabled")) -> ()  [unwired: 2 in, 2 out]
            n1085 = property on="Scan Go" class="Bool"("DisabledEnum"=T2."Disabled and Grayed Out" ("Disabled")) -> ()  [unwired: 2 in, 2 out]
            n1086 = property on="Scan Cancel" class="Bool"("DisabledEnum"=T2."Disabled and Grayed Out" ("Disabled")) -> ()  [unwired: 2 in, 2 out]
          }
        }
      }
      event #24 {
        n1087 = event-data() -> ()  [unwired: 1 in, 7 out]
        n1088 = flat-sequence {
          tunnel: [w1943] -> w1922
          tunnel: w1923 -> [w1945]
          tunnel: [w1944] -> w1921
          tunnel: w1924 -> [w1946]
          frame #0 {
            n1089 = property on="Reset X Motor Steps" class="DigNum (strict)"() -> ("Value"=w1949:i32)  [unwired: 2 in, 2 out]
            n1090 = Number To Decimal String(number=w1949) -> (decimal integer string=w1947:string)  [unwired: 1 in]
            n1091 = call "Applied Send Command.vi"("error in (no error)"=w1945, "Extra"=w1947, "Command"=T1."Set ABS Position", "VISA resource name"=w1946) -> ("error out"=w1944:errorcluster, "VISA resource name out"=w1943:refnum<visa-resource-name>)  [unwired: 3 in, 1 out]
          }
        }
        n1092 = flat-sequence {
          tunnel: w1928 -> [w1954]
          tunnel: w1927 -> [w1951]
          tunnel: [w1953] -> w1926
          tunnel: [w1952] -> w1925
          frame #0 {
            n1093 = property on="Reset Y Motor Steps" class="DigNum (strict)"() -> ("Value"=w1956:i32)  [unwired: 2 in, 2 out]
            n1094 = Number To Decimal String(number=w1956) -> (decimal integer string=w1955:string)  [unwired: 1 in]
            n1095 = call "Applied Send Command.vi"("error in (no error)"=w1951, "Extra"=w1955, "Command"=T1."Set ABS Position", "VISA resource name"=w1954) -> ("error out"=w1952:errorcluster, "VISA resource name out"=w1953:refnum<visa-resource-name>)  [unwired: 3 in, 1 out]
          }
        }
        n1096 = flat-sequence {
          tunnel: [w1934] -> w1916
          tunnel: [w1933] -> w1915
          tunnel: w1918 -> [w1932]
          tunnel: w1917 -> [w1931]
          frame #0 {
            n1097 = property on="Reset R Motor Steps" class="DigNum (strict)"() -> ("Value"=w1935:i32)  [unwired: 2 in, 2 out]
            n1098 = Number To Decimal String(number=w1935) -> (decimal integer string=w1930:string)  [unwired: 1 in]
            n1099 = call "Applied Send Command.vi"("error in (no error)"=w1931, "Extra"=w1930, "Command"=T1."Set ABS Position", "VISA resource name"=w1932) -> ("error out"=w1933:errorcluster, "VISA resource name out"=w1934:refnum<visa-resource-name>)  [unwired: 3 in, 1 out]
          }
        }
        n1100 = flat-sequence {
          tunnel: [w1941] -> w1914
          tunnel: [w1940] -> w1913
          tunnel: w1920 -> [w1938]
          tunnel: w1919 -> [w1939]
          frame #0 {
            n1101 = property on="Reset Z Motor Steps" class="DigNum (strict)"() -> ("Value"=w1942:i32)  [unwired: 2 in, 2 out]
            n1102 = Number To Decimal String(number=w1942) -> (decimal integer string=w1936:string)  [unwired: 1 in]
            n1103 = call "Applied Send Command.vi"("error in (no error)"=w1939, "Extra"=w1936, "Command"=T1."Set ABS Position", "VISA resource name"=w1938) -> ("error out"=w1940:errorcluster, "VISA resource name out"=w1941:refnum<visa-resource-name>)  [unwired: 3 in, 1 out]
          }
        }
      }
    }
    n1104 = case shown="True" "Delete Button" {
      tunnel: w377 -> [_ w402]
      frame #0 {
      }
      frame #1 {
        n1105 = property on="Preset positions" class="Ring (strict)"() -> ("Value"=w400:i32)  [unwired: 2 in, 2 out]
        n1106 = Delete From Array(array=w402, index=w400) -> (array with subset deleted=w401:string[])  [unwired: 1 in, 1 out]
        n1107 = property on="Presets" class="Arr (strict)"() -> ("Value"=w399:i32[][])  [unwired: 2 in, 2 out]
        n1108 = property on="Preset positions" class="Ring (strict)"("Strings []"=w401) -> ()  [unwired: 2 in, 2 out]
        n1109 = Delete From Array(array=w399, index (row)=w400) -> (array with subset deleted=w398:i32[][])  [unwired: 2 in, 1 out]
        n1110 = property on="Presets" class="Arr (strict)"("Val(Sgnl)"=w398) -> ()  [unwired: 2 in, 2 out]
      }
    }
    n1111 = case shown="True" "Set Button" {
      tunnel: "Preset positions" -> [_ w420]
      frame #0 {
      }
      frame #1 {
        n1112 = property on="Presets" class="Arr (strict)"() -> ("Value"=w417:i32[][])  [unwired: 2 in, 2 out]
        n1113 = Index Array(array=w417, index (row)=w420) -> (element=w419:i32[])  [unwired: 1 in]
        n1114 = Array To Cluster(array=w419) -> (cluster=w418:T4)
        n1115 = Unbundle(w418) -> ("Value[0]"=w416:i32, "Value[1]"=w415:i32, "Value[2]"=w414:i32, "Value[3]"=w413:i32)  [unwired: 5 out]
        n1116 = property on="X Step SP" class="DigNum (strict)"("Val(Sgnl)"=w416) -> ()  [unwired: 2 in, 2 out]
        n1117 = property on="Y Step SP" class="DigNum (strict)"("Val(Sgnl)"=w415) -> ()  [unwired: 2 in, 2 out]
        n1118 = property on="Z Step SP" class="DigNum (strict)"("Val(Sgnl)"=w414) -> ()  [unwired: 2 in, 2 out]
        n1119 = property on="R Step SP" class="DigNum (strict)"("Val(Sgnl)"=w413) -> ()  [unwired: 2 in, 2 out]
      }
    }
    n1120 = case shown="True" "Add Button" {
      tunnel: w377 -> [_ w412]
      frame #0 {
      }
      frame #1 {
        n1121 = property on="X Step PV" class="DigNum (strict)"() -> ("Value"=w407:i32)  [unwired: 2 in, 2 out]
        n1122 = property on="Y Step PV" class="DigNum (strict)"() -> ("Value"=w406:i32)  [unwired: 2 in, 2 out]
        n1123 = property on="Z Step PV" class="DigNum (strict)"() -> ("Value"=w405:i32)  [unwired: 2 in, 2 out]
        n1124 = property on="R Step PV" class="DigNum (strict)"() -> ("Value"=w404:i32)  [unwired: 2 in, 2 out]
        n1125 = Build Array(w407, w406, w405, w404) -> (w410:i32[])
        n1126 = Build Array (concatenate)(w412, "String") -> (w411:string[])
        n1127 = property on="Preset positions" class="Ring (strict)"("Strings []"=w411) -> ()  [unwired: 2 in, 2 out]
        n1128 = property on="Presets" class="Arr (strict)"() -> ("Value"=w409:i32[][])  [unwired: 2 in, 2 out]
        n1129 = Build Array (concatenate)(w409, w410) -> (w403:i32[][])
        n1130 = property on="Presets" class="Arr (strict)"("Val(Sgnl)"=w403) -> ()  [unwired: 2 in, 2 out]
      }
    }
  }
  n1131 = flat-sequence {
    tunnel: w70 -> [w1958]
    tunnel: w69 -> [w1957]
    tunnel: [w1969] -> w46
    frame #0 {
      # "GET CURRENT POSITION"
      n1132 = call "Applied Send Command.vi"("error in (no error)"=w1957, "Extra"="", "Command"=T1."Immediate Position?", "VISA resource name"=w1958) -> ("error out"=w1959:errorcluster, "read buffer"=w1964:string, "VISA resource name out"=w1960:refnum<visa-resource-name>)  [unwired: 3 in]
      n1133 = call "Applied Send Command.vi"("error in (no error)"=w1959, "Command"=T1."Stop & Kill Buffer", "VISA resource name"=w1960) -> ("error out"=w1966:errorcluster, "VISA resource name out"=w1967:refnum<visa-resource-name>)  [unwired: 4 in, 1 out]
      n1134 = Hexadecimal String To Number(string=w1964, offset=3) -> (number=w1961:u32)  [unwired: 1 in, 1 out]
      n1135 = VISA Close(VISA resource name=w1967, error in (no error)=w1966) -> ()  [unwired: 1 out]
      n1136 = To Long Integer(number=w1961) -> (32bit integer=w1969:i32)
    }
  }
  n1137 = flat-sequence {
    tunnel: w50 -> [w1972]
    tunnel: w49 -> [w1971]
    tunnel: [w1970] -> w45
    frame #0 {
      # "GET CURRENT POSITION"
      n1138 = call "Applied Send Command.vi"("error in (no error)"=w1971, "Extra"="", "Command"=T1."Immediate Position?", "VISA resource name"=w1972) -> ("error out"=w1973:errorcluster, "read buffer"=w1978:string, "VISA resource name out"=w1974:refnum<visa-resource-name>)  [unwired: 3 in]
      n1139 = call "Applied Send Command.vi"("error in (no error)"=w1973, "Command"=T1."Stop & Kill Buffer", "VISA resource name"=w1974) -> ("error out"=w1980:errorcluster, "VISA resource name out"=w1981:refnum<visa-resource-name>)  [unwired: 4 in, 1 out]
      n1140 = Hexadecimal String To Number(string=w1978, offset=3) -> (number=w1975:u32)  [unwired: 1 in, 1 out]
      n1141 = VISA Close(VISA resource name=w1981, error in (no error)=w1980) -> ()  [unwired: 1 out]
      n1142 = To Long Integer(number=w1975) -> (32bit integer=w1970:i32)
    }
  }
  n1143 = flat-sequence {
    tunnel: w52 -> [w1984]
    tunnel: w51 -> [w1983]
    tunnel: [w1985] -> w44
    frame #0 {
      # "GET CURRENT POSITION"
      n1144 = call "Applied Send Command.vi"("error in (no error)"=w1983, "Extra"="", "Command"=T1."Immediate Position?", "VISA resource name"=w1984) -> ("error out"=w1986:errorcluster, "read buffer"=w1991:string, "VISA resource name out"=w1987:refnum<visa-resource-name>)  [unwired: 3 in]
      n1145 = call "Applied Send Command.vi"("error in (no error)"=w1986, "Command"=T1."Stop & Kill Buffer", "VISA resource name"=w1987) -> ("error out"=w1993:errorcluster, "VISA resource name out"=w1994:refnum<visa-resource-name>)  [unwired: 4 in, 1 out]
      n1146 = Hexadecimal String To Number(string=w1991, offset=3) -> (number=w1988:u32)  [unwired: 1 in, 1 out]
      n1147 = VISA Close(VISA resource name=w1994, error in (no error)=w1993) -> ()  [unwired: 1 out]
      n1148 = To Long Integer(number=w1988) -> (32bit integer=w1985:i32)
    }
  }
  n1149 = flat-sequence {
    tunnel: w48 -> [w1997]
    tunnel: w47 -> [w1996]
    tunnel: [w1998] -> w43
    frame #0 {
      # "GET CURRENT POSITION"
      n1150 = call "Applied Send Command.vi"("error in (no error)"=w1996, "Extra"="", "Command"=T1."Immediate Position?", "VISA resource name"=w1997) -> ("error out"=w1999:errorcluster, "read buffer"=w2004:string, "VISA resource name out"=w2000:refnum<visa-resource-name>)  [unwired: 3 in]
      n1151 = call "Applied Send Command.vi"("error in (no error)"=w1999, "Command"=T1."Stop & Kill Buffer", "VISA resource name"=w2000) -> ("error out"=w2006:errorcluster, "VISA resource name out"=w2007:refnum<visa-resource-name>)  [unwired: 4 in, 1 out]
      n1152 = Hexadecimal String To Number(string=w2004, offset=3) -> (number=w2001:u32)  [unwired: 1 in, 1 out]
      n1153 = VISA Close(VISA resource name=w2007, error in (no error)=w2006) -> ()  [unwired: 1 out]
      n1154 = To Long Integer(number=w2001) -> (32bit integer=w1998:i32)
    }
  }
  n1155 = flat-sequence {
    tunnel: w46 -> [w2014]
    tunnel: w45 -> [w2013]
    tunnel: w44 -> [w2012]
    tunnel: w43 -> [w2011]
    frame #0 {
      n1156 = Build Array(w2014, w2013, w2012, w2011) -> (w2009:i32[])
      n1157 = call-poly <vilib>:"Write To Spreadsheet File.vi"("1D data"=w2009, "file path (dialog if empty)"=path "S:/LV codes/SCL2/POS.TXT") -> ()  [unwired: 6 in, 1 out]
    }
    frame #1 {
      n1158 = property on="Presets" class="Arr (strict)"() -> ("Value"=w2021:i32[][])  [unwired: 2 in, 2 out]
      n1159 = property on="Preset positions" class="Ring (strict)"() -> ("Strings []"=w2017:string[])  [unwired: 2 in, 2 out]
      n1160 = Number To Decimal String(number=w2021) -> (decimal integer string=w2015:string[][])  [unwired: 1 in]
      n1161 = Transpose 2D Array(2D array=w2015) -> (transposed array=w2016:string[][])
      n1162 = Build Array (concatenate)(w2017, w2016) -> (w2018:string[][])
      n1163 = Transpose 2D Array(2D array=w2018) -> (transposed array=w2019:string[][])
      n1164 = call-poly <vilib>:"Write To Spreadsheet File.vi"("2D data"=w2019, "file path (dialog if empty)"=path "S:/LV codes/SCL2/PRESET.TXT") -> ()  [unwired: 6 in, 1 out]
    }
  }
